vi "MC_8_28_12a_JW - Copy.vi"() -> ()   [LabVIEW 2011]
uses:
  <vilib>/Utility/file.llb/Read From Spreadsheet File (string).vi
  <vilib>/regexp/Match Regular Expression.xnode
  <vilib>/Utility/file.llb/Write To Spreadsheet File (string).vi
  <vilib>/Utility/file.llb/Write To Spreadsheet File (DBL).vi
  <vilib>/Utility/inputDevices.llb/keyboardAcquire.vi
panel:
  out "Vg Column":dbl[](array[numeric])
  out "Data Length":dbl
  out "X Axis Display Type":string
  out "Opj X Axis":string
  in  "Room Temp":dbl=294.0
  out "No Image 2":path=path "\\\\acad1\\physics/Jurchescu-group/JW-PD/Image Not Found.png"
  out "Save1 Array":string[][](array[string])
  out "Lin Vd":dbl
  out "Lin-Vg Array-Used":dbl[](array[numeric])
  out "Lin Id-Used":dbl[](array[numeric])
  out "Rec: Comments":string
  out "Folder Index":dbl caption="Length"
  out "Current \nRecord":string[](array[string])
  out "Transformer \nHeaders":string[](array[string])
  out "Current Device ID":string
  out "Column":string
  out "Row":string
  out "Rec: Concentration":dbl
  out "Rec: Solvent":string
  out "Rec: Method":string
  in  "?":T1(tab)
  in  "Transport File":path
  out "Transport Folder":path
  out "Rec: Material":string
  out "Accel (RPM/s):":dbl
  in  "Transfer File":path
  out "Transfer Folder":path
  in  "Image Folder":path
  out "Image File":path=path "D:/UserData/Desktop/Jeremy/WFU/Research/Programs/VI mods/Image Not Found.png"
  in  "Manual Comments":bool
  in  "Comments:":string
  out "Calc: On/Off":dbl caption="On/Off-Sat" format="%#.2e"
  out "Calc: Off I-Sat":dbl caption="Off I-Sat" format="%#.2e"
  in  "Manuel-Dielectric":bool
  in  "Manuel-Length":bool
  out "Calc: VT-Lin":dbl
  out "New: VT-Lin":dbl
  out "Rec: VT-Lin":dbl caption="VT-Lin" format="%#_3g"
  out "Calc: Trap Density-STS":dbl format="%#.2e"
  out "New: Trap Density-STS":dbl format="%#.2e"
  out "Rec: Trap Density-STS":dbl caption="N-Sat (STS)" format="%#.2e"
  out "Calc: Trap Density-VT":dbl format="%#.2e"
  out "New: Trap Density-VT":dbl format="%#.2e"
  out "Rec: Trap Density-VT":dbl caption="N-Sat (VT)" format="%#.2e"
  out "Calc: Mobility-Lin":dbl format="%#.2e"
  out "New: Mobility-Lin":dbl format="%#_4e"
  out "Rec: Mobility-Lin":dbl caption="Mobility-Lin" format="%#_3e"
  out "Calc: Mobility-Sat":dbl format="%#.2e"
  out "Rec: Length":dbl caption="Length" format="%#_3g"
  out "Rec: Width":dbl caption="Width" format="%#_4g"
  out "Rec: Dielectric (d)":dbl caption="Dielectric (d)" format="%#_3g"
  in  "Cancel Button":bool
  in  "Up Button":bool
  in  "Down Button":bool
  out "Data Name:":string
  in  "Save Changes?":bool
  in  "New: Dielectric":dbl
  in  "New: Length":dbl
  in  "New: Width":dbl
  out "New: Mobility-Sat":dbl format="%#.2e"
  in  "Blank Button":bool
  in  "Zoom":i16(slide)=-3 scale=-5.0..5.0
  out "Image Out 2":T2(plugin-control)
  out "Image Out":T2(plugin-control)
  in  "Magnification":u16(ring) items=["5x", "10x", "20x", "50x", "80x"]
  out "Total Width":dbl
  out "Distances":dbl[](array[numeric])
  in  "Undo Button":bool
  in  "Remove Button":bool
  out "Rec: Mobility-Sat":dbl caption="Mobility-Sat" format="%#.2e"
  in  "Export":bool
  out "Calc: VT-Sat":dbl format="%#.2g"
  out "New: VT-Sat":dbl format="%#.2g"
  in  "Manual-Width":bool caption="Manual"
  out "Calc: STS":dbl format="%#.2g"
  out "New: STS":dbl format="%#.2g"
  out "Rec: VT-Sat":dbl caption="VT-Sat" format="%#.2g"
  out "Rec: STS":dbl caption="STS-Sat" format="%#.2g"
  out "Rec: On/Off":dbl caption="On/Off-Sat" format="%#.2e"
  in  "Save Changes? 2":bool
  in  "Save Changes? 3":bool
  out "Rec: Temp":dbl caption="Sample Temp" format="%.1f"
  in  "New: Temp":dbl format="%.1f"
  out "Rec: Off I-Sat":dbl caption="Off I-Sat" format="%#.2e"
  in  "Independant Variable":string(combo)="Length (um):"
  in  "Transfer Plots":T3(tab)=enum."Saturation"
  in  "Lin-Trans Slider":dbl(slide) step=1.0 scale=-22.0..89.0 scale format="%#_1p"
  out "Sqrt-Lin":cluster{dbl[], dbl[]}[](graph)
  in  "Next Sqrt Lin":bool
  in  "Previous Sqrt Lin":bool
  in  "Sat-Trans Slider":dbl(slide) step=1.0 scale=-40.0..40.0 scale format="%#_1p"
  out "Sqrt-Sat":cluster{dbl[], dbl[]}[](graph)
  in  "Previous Sqrt Sat":bool
  in  "Next Sqrt Sat":bool
  out "Raw- Lin":cluster{dbl[], dbl[]}[](graph)
  out "Raw- Sat":cluster{dbl[], dbl[]}[](graph)
  in  "Log Plots":enum32{"Linear", "Saturation", "Transport"}(tab)=enum."Saturation"
  in  "Lin-Log Slider":dbl(slide) step=1.0 scale=-1.0..82.0 scale format="%#_1p"
  in  "Previous Log Lin":bool
  in  "Next Log Lin":bool
  out "Log-Lin":cluster{dbl[], dbl[]}[](graph)
  in  "Sat-Log Slider":dbl(slide) step=1.0 scale=-1.0..82.0 scale format="%#_1p"
  in  "Previous Log Sat":bool
  in  "Next Log Sat":bool
  out "Sat-Log":cluster{dbl[], dbl[]}[](graph)
  out "Transport":cluster{dbl[], dbl[]}[](graph)
  in  "Manual-Temp":bool caption="Manual"
  out "Date Created":string caption="Fabricated"
  out "Date Recorded":string="Date Recorded" caption="Measured"
  out "Image Name":string
  out "Index":string
  in  "Num Pts":dbl=5.0
  in  "NumPoints Log":dbl=5.0 caption="Num Pts"
  in  "Transport Style Controls":T4 {"Transport Line Size" items=["Extra Small", "Small", "Medium", "Large", "Extra Large"]}
  in  "Origin Project File":path=path "\\\\acad1\\physics/Jurchescu-group/JW-PD/Group Library/Origin Project Files/DeviceData_8_10_12a_JW.opj"
  in  "No Image File":path=path "\\\\acad1\\physics/Jurchescu-group/JW-PD/Mega Awesome/Image Not Found.png"
  in  "Ramp (s):":dbl=3.0
  in  "Fabricator:":string="NaN"
  in  "Sample #:":dbl=1.0
  in  "Wait Time (s):":dbl=nan
  in  "RPM:":dbl=nan
  in  "Time (s):":dbl=nan
  in  "Room Temp (F):":dbl=nan
  in  "Relative Humidity (%):":dbl=nan
  in  "Solution Temp (C):":dbl=nan
  in  "# Drops*:":dbl=inf
  in  "Surface Treatment:":string="NaN"
  in  "Treatment Concentration (mM):":dbl=nan
  out "String":string
  out "Index 2":dbl
  out "Sat Id-Log-Used":dbl[](array[numeric])
  out "Vg Array-Log-Used":dbl[](array[numeric])
  out "ROI Descriptor out":T5 {"Contours"."Type" items=["No Selection", "Point", "Line", "Rectangle", "Oval", "Polygon", "Freehand Region", "Annulus", "Unused2", "Unused3", "Broken Line", "Freehand Line", "Rotated Rectangle"]}
  out "ROI Descriptor":T5 {"Contours"."Type" items=["No Selection", "Point", "Line", "Rectangle", "Oval", "Polygon", "Freehand Region", "Annulus", "Unused2", "Unused3", "Broken Line", "Freehand Line", "Rotated Rectangle"]}
  out "Numeric 3":dbl
  out "Array 6":dbl[][](array[numeric])
  out "Cluster":T6
  out "Array 5":dbl[](array[numeric])
  out "Array 4":dbl[](array[numeric])
  out "Array 3":dbl[](array[numeric])
  out "Numeric 2":dbl
  out "Numeric":dbl
  out "Sat Id-Used":dbl[](array[numeric])
  out "Sat Vg Array-Used":dbl[](array[numeric])
  out "MobVi Index":dbl
  in  "Row Start":dbl=20.0
  # "Data Locations"
  # "Transfer Location"
  # "Image Location"
  # "Recorded"
  # "Calculated"
  # "Re-Calculated"
  # "Manual"
  # "Used points display at y=0"
  # "Slider\nDoesn't\nWork"
  # "Slider\nDoesn't\nWork"
  # "No new points displayed"
  # "Sample Properties"
  # "*     Inf = Full coverage\n   NaN = Unknown or Not Applicable"
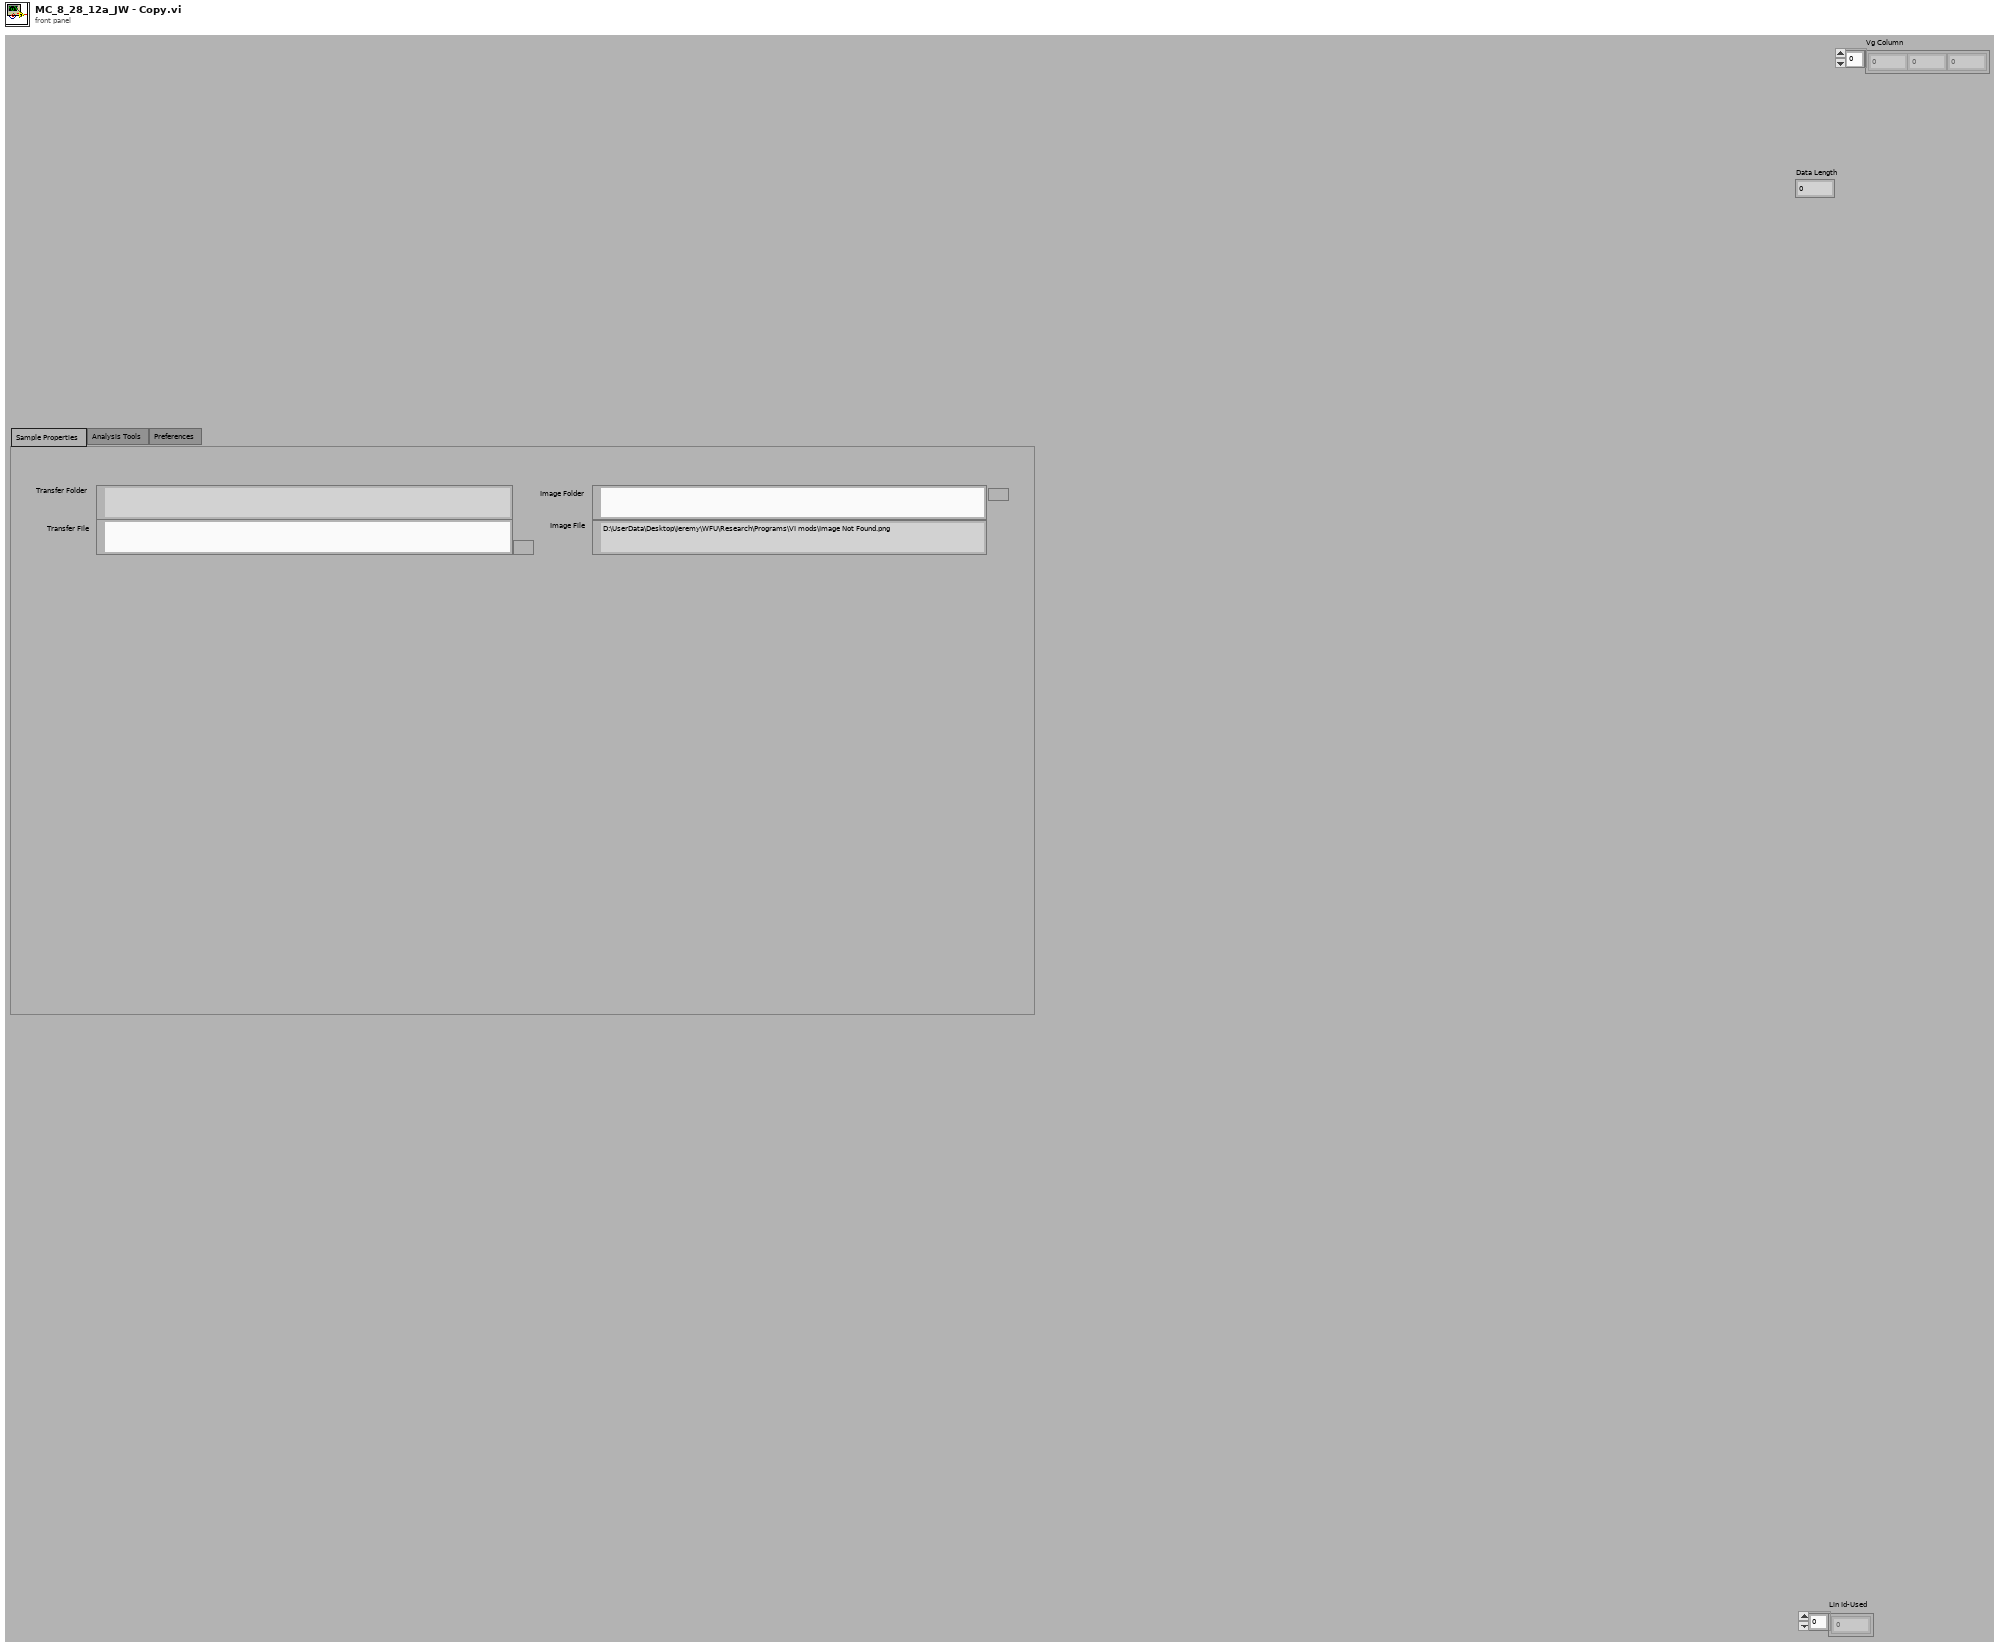
[diagram p1: front panel]
types:
  T1 = enum32{"Sample Properties", "Analysis Tools", "Preferences", "Current Database"}
  T2 = typedef "IMAQ Image.ctl" = refnum<image>
  T3 = enum32{"Linear", "Saturation", "Raw-Linear", "Raw-Saturation"}
  T4 = cluster{"Transport Line Size":u16, "Transport Line Color":u32}
  T5 = typedef "ROI Descriptor" = cluster{"Global Rectangle":i32[], "Contours":cluster{"ID":enum32{"External", "Internal"}, "Type":u32, "Coordinates":i32[]}[]}
  T6 = cluster{"Numeric":dbl, "Numeric 2":dbl, "Numeric 3":dbl, "Numeric 4":dbl}
  T7 = cluster{"Mobility-Sat":dbl, "Moblitity-Lin":dbl, "On/Off":dbl, "Off Current":dbl, "Vt-Sat":dbl, "STS":dbl, "Trap Density-VT":dbl, "Trap Density-STS":dbl}
  T8 = cluster{"Date Recorded":string, "Index":string, "Length":dbl, "Width":dbl, "Sample Temp":dbl}
  T9 = cluster{"Date Created":string, "Material":string, "Solvent":string, "Concentration":dbl, "Method":string, "Dielectric (nm)":dbl, "Treatment":string, "Comments":string}
  T10 = cluster{"Sat Vg Used":dbl[], "Sat Log(Id) Used":dbl[], "Lin Vg Used":dbl[], "Lin Log(Id) Used":dbl[], "STS Index-Sat":dbl, "STS Index-Lin":dbl}
  T11 = cluster{"Raw Sat":cluster{dbl[], dbl[]}[], "Sqrt Sat":cluster{dbl[], dbl[]}[], "Log Sat":cluster{dbl[], dbl[]}[], "Raw Lin":cluster{dbl[], dbl[]}[], "Sqrt Lin":cluster{dbl[], dbl[]}[], "Log Lin":cluster{dbl[], dbl[]}[]}
  T12 = cluster{"Mobility-Sat":dbl, "Vt-Sat":dbl, "Mobility-Lin":dbl, "Vt-Lin":dbl, "Off I-Sat":dbl, "On/Off I-Sat":dbl}
  T13 = cluster{"[0]":cluster{dbl[], dbl[]}, "[1]":cluster{dbl[], dbl[]}, "[2]":cluster{dbl[], dbl[]}, "[3]":cluster{dbl[], dbl[]}, "[4]":cluster{dbl[], dbl[]}, "[5]":cluster{dbl[], dbl[]}, "[6]":cluster{dbl[], dbl[]}, "[7]":cluster{dbl[], dbl[]}, "[8]":cluster{dbl[], dbl[]}}
  T14 = typedef "LVBoundsTypeDef.ctl" = cluster{"Width":u32, "Height":u32}
  T15 = cluster{"Global Rectangle":i32[], "Contours":cluster{"Contour Type":u32, "ROI Type":u32, "Points":i32[]}[]}
  T16 = cluster{"Contour Type":u32, "ROI Type":u32, "Points":i32[]}[]
  T17 = cluster{i32[], cluster{"Contour Type":u32, "ROI Type":u32, "Points":i32[]}[]}
  T18 = enum16{"0", "1", "2", "3", "4", "5", "6", "7", "8", "9", "A", "B", "C", "D", "E", "F", "G", "H", "I", "J", "K", "L", "M", "N", "O", "P", "Q", "R", "S", "T", "U", "V", "W", "X", "Y", "Z", "F1", "F2", "F3", "F4", "F5", "F6", "F7", "F8", "F9", "F10", "F11", "F12", "F13", "F14", "F15", "ADD", "BACK", "BACKSLASH", "CAPITAL", "COMMA", "DECIMAL", "DELETE", "DIVIDE", "DOWN", "END", "EQUALS", "ESCAPE", "GRAVE (`)", "HOME", "INSERT", "LBRACKET", "LCONTROL", "LEFT", "L ALT", "LSHIFT", "LWIN", "MINUS", "MULTIPLY", "NEXT", "NUMLOCK", "NUMPAD_0", "NUMPAD_1", "NUMPAD_2", "NUMPAD_3", "NUMPAD_4", "NUMPAD_5", "NUMPAD_6", "NUMPAD_7", "NUMPAD_8", "NUMPAD_9", "PAUSE", "PERIOD", "PRIOR (PG UP)", "RBRACKET", "RCONTROL", "RETURN", "RIGHT", "R ALT", "RSHIFT", "RWIN", "SCROLL", "SEMICOLON", "SLASH", "SPACE", "SUBTRACT", "TAB", "UP", "ENTER (num pad)", "' (quote)"}[]
  T19 = enum16{"0", "1", "2", "3", "4", "5", "6", "7", "8", "9", "A", "B", "C", "D", "E", "F", "G", "H", "I", "J", "K", "L", "M", "N", "O", "P", "Q", "R", "S", "T", "U", "V", "W", "X", "Y", "Z", "F1", "F2", "F3", "F4", "F5", "F6", "F7", "F8", "F9", "F10", "F11", "F12", "F13", "F14", "F15", "ADD", "BACK", "BACKSLASH", "CAPITAL", "COMMA", "DECIMAL", "DELETE", "DIVIDE", "DOWN", "END", "EQUALS", "ESCAPE", "GRAVE (`)", "HOME", "INSERT", "LBRACKET", "LCONTROL", "LEFT", "L ALT", "LSHIFT", "LWIN", "MINUS", "MULTIPLY", "NEXT", "NUMLOCK", "NUMPAD_0", "NUMPAD_1", "NUMPAD_2", "NUMPAD_3", "NUMPAD_4", "NUMPAD_5", "NUMPAD_6", "NUMPAD_7", "NUMPAD_8", "NUMPAD_9", "PAUSE", "PERIOD", "PRIOR (PG UP)", "RBRACKET", "RCONTROL", "RETURN", "RIGHT", "R ALT", "RSHIFT", "RWIN", "SCROLL", "SEMICOLON", "SLASH", "SPACE", "SUBTRACT", "TAB", "UP", "ENTER (num pad)", "' (quote)"}
  T20 = cluster{"Independant  Variable Indicator":string, "Parameter String Indicator":string}
  T21 = cluster{string, sgl, bool, bool, bool, bool, bool, bool, i32}
  T22 = cluster{i32, cluster{string, sgl, bool, bool, bool, bool, bool, bool, i32}, i32, i32}
  T23 = cluster{"Contour Type":u32, "ROI Type":u32, "Points":i32[]}
  T24 = cluster{"Points[0]":i32, "Points[1]":i32, "Points[2]":i32, "Points[3]":i32, "Points[4]":i32, "Points[5]":i32, "Points[6]":i32, "Points[7]":i32, "Points[8]":i32}
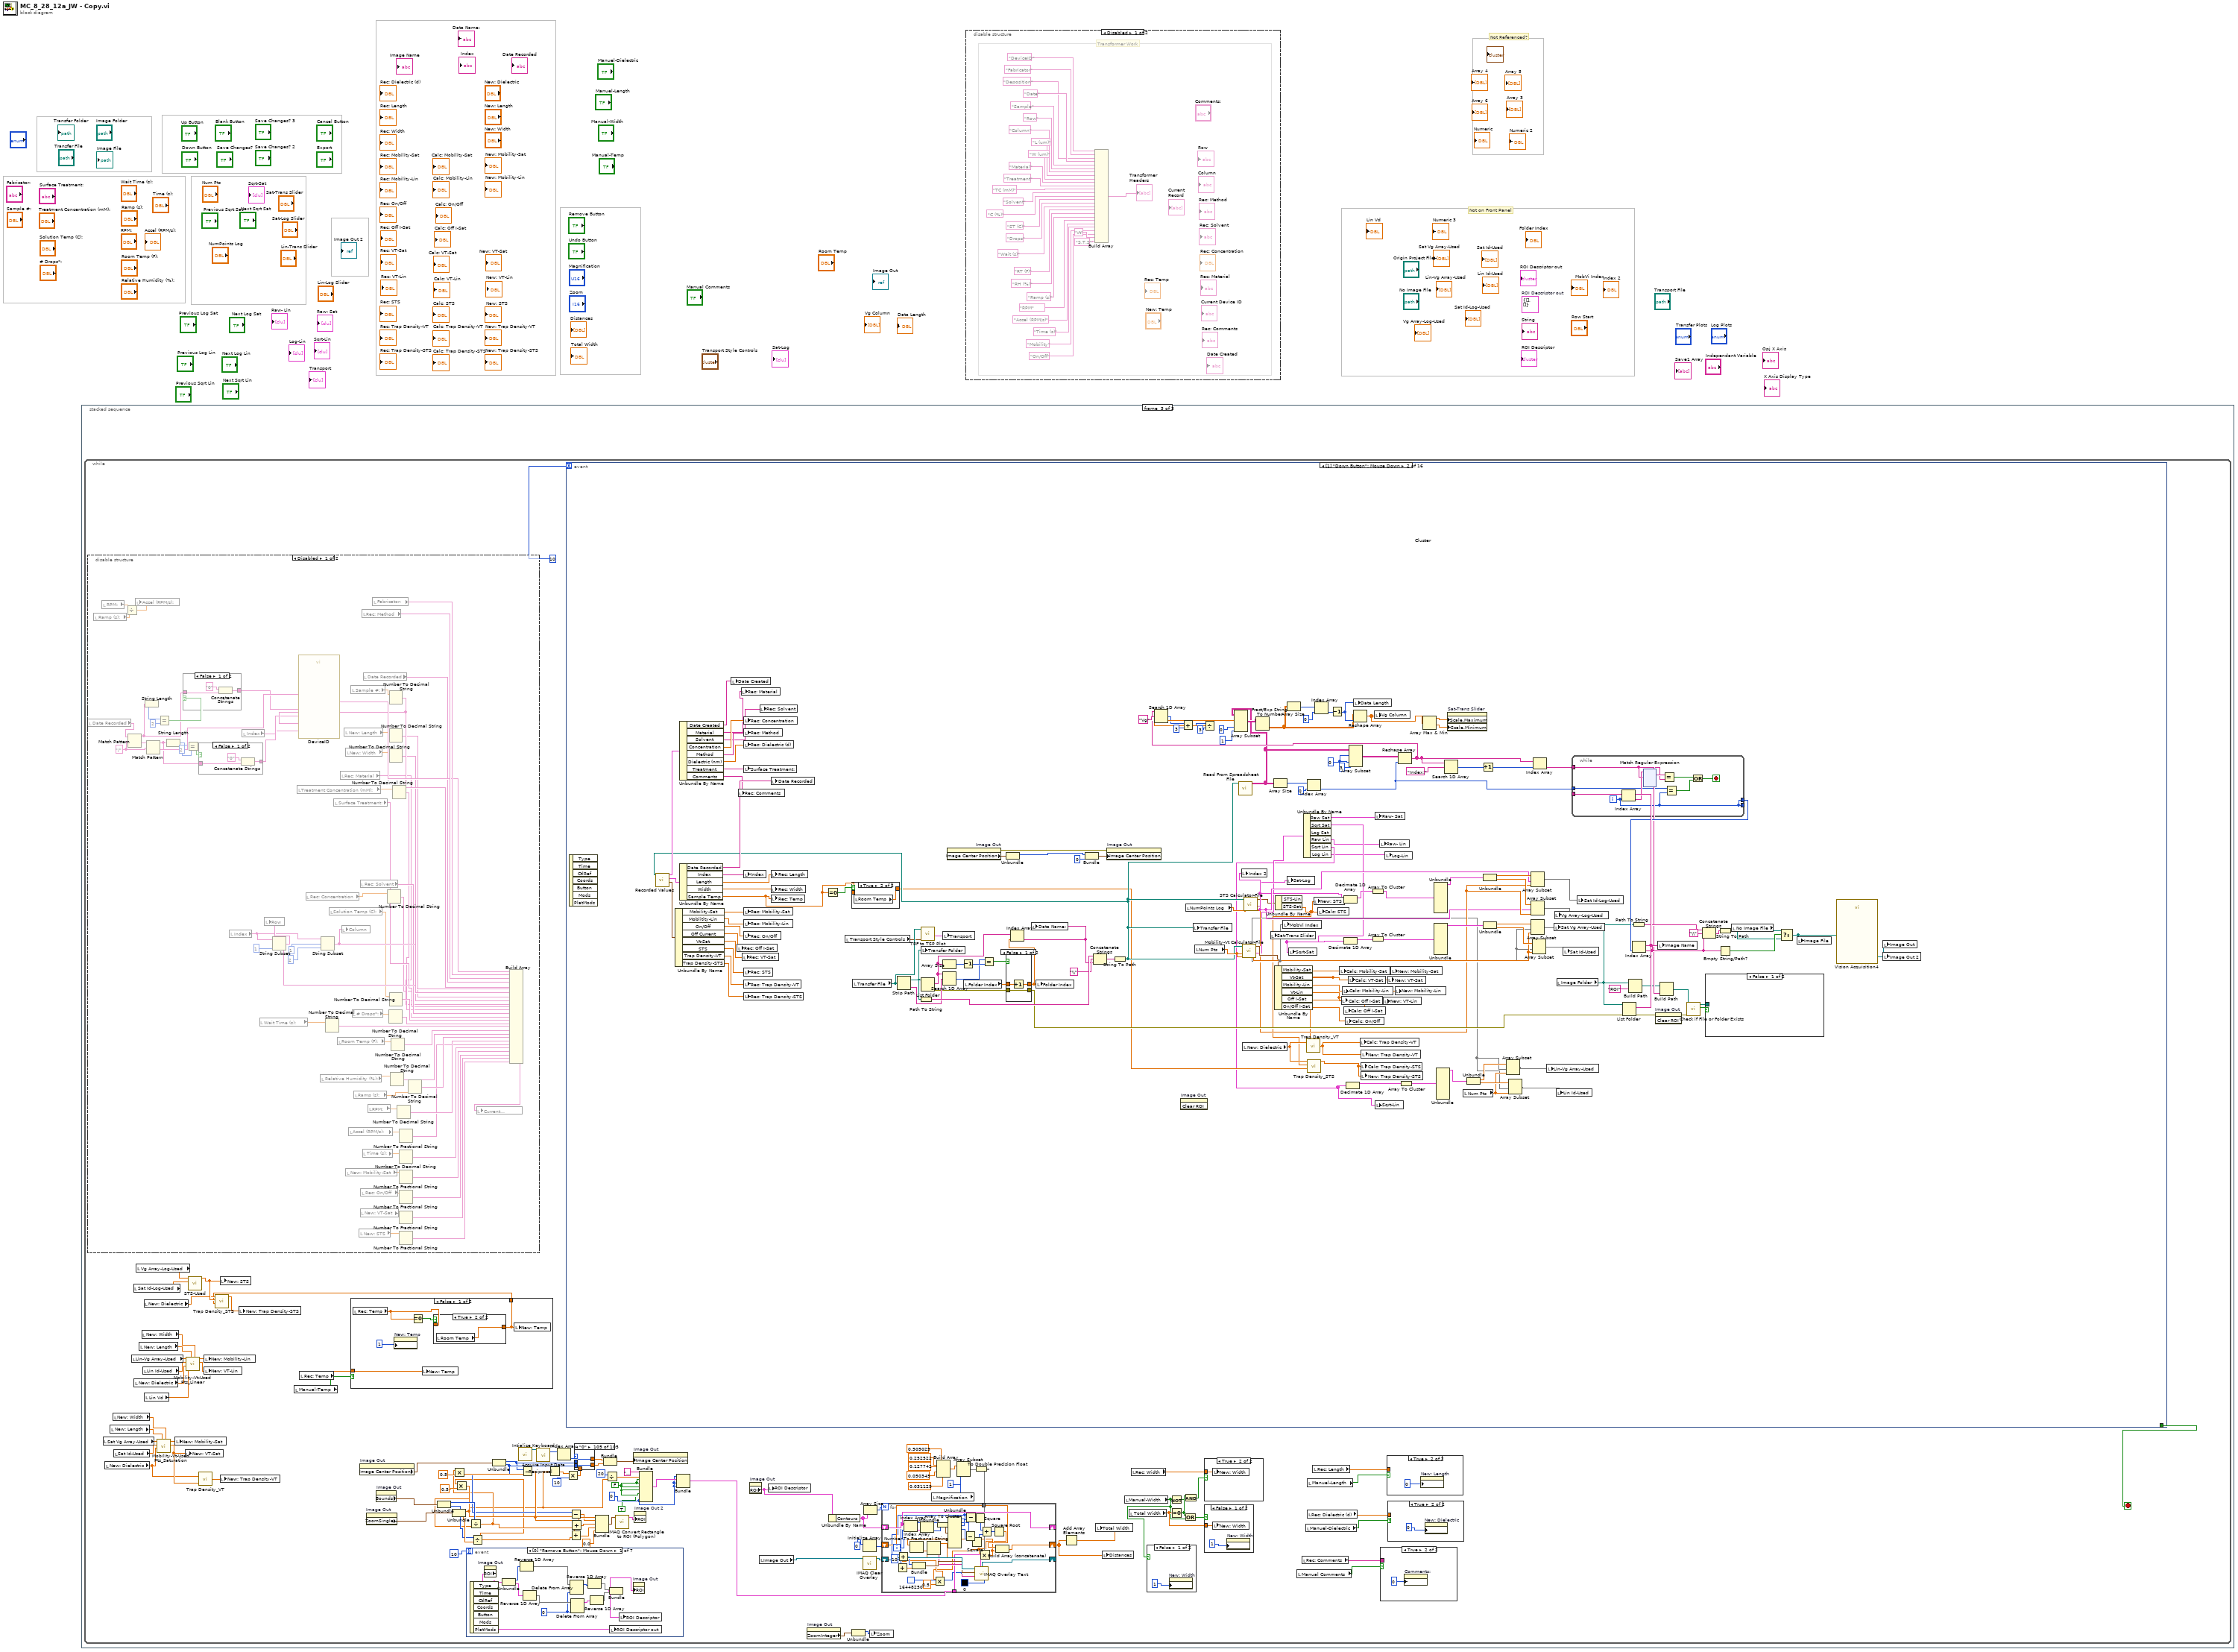
[diagram p0: block diagram]
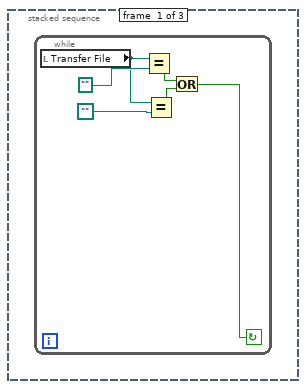
[diagram p3: hidden frame]
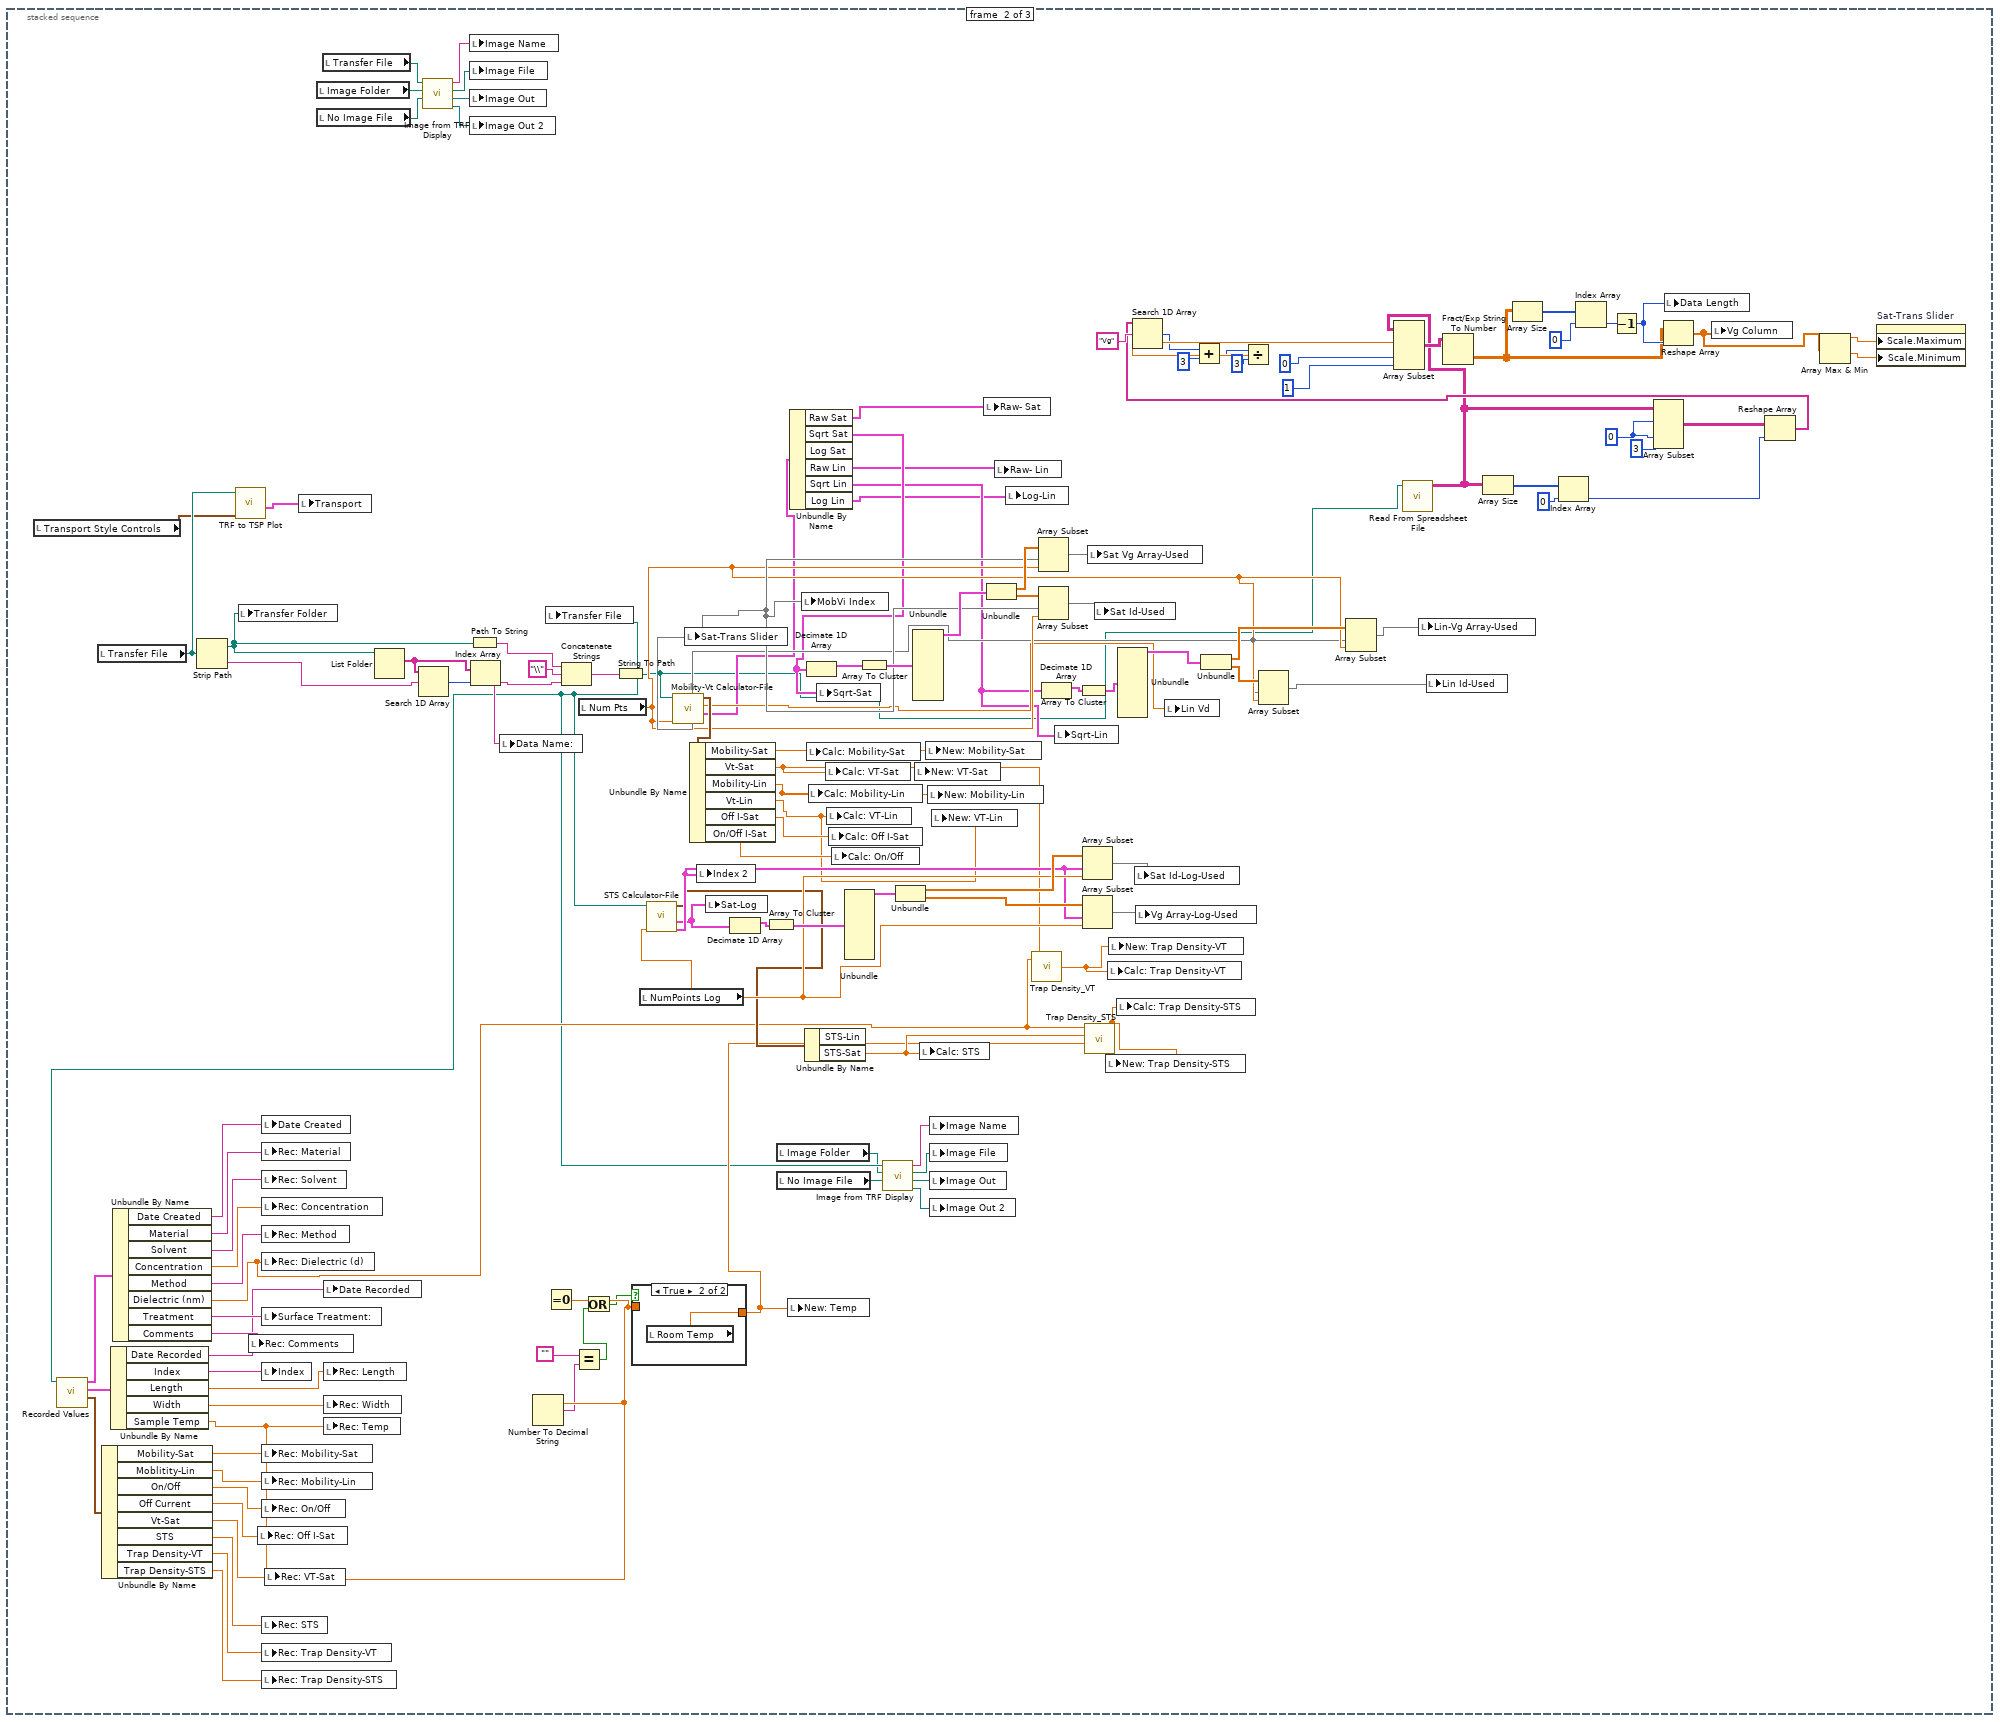
[diagram p4: hidden frame]
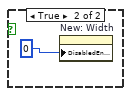
[diagram p9: hidden frame]
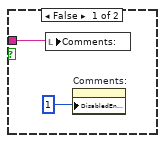
[diagram p10: hidden frame]
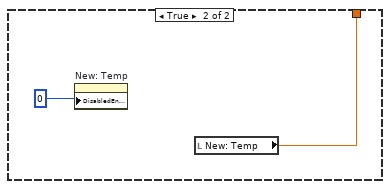
[diagram p12: hidden frame]
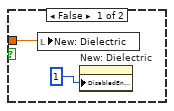
[diagram p13: hidden frame]
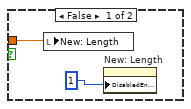
[diagram p14: hidden frame]
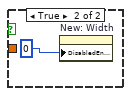
[diagram p16: hidden frame]
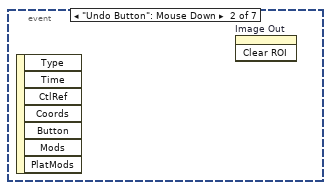
[diagram p17: hidden frame]
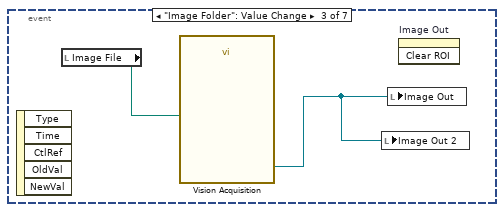
[diagram p18: hidden frame]
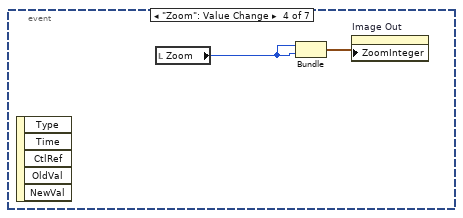
[diagram p19: hidden frame]
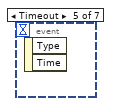
[diagram p20: hidden frame]
diagram:
  (unwired) T5 {"Global Rectangle"=[], "Contours"=[]}  # ROI Descriptor out
  # "Not Referenced?"
  # "Not on Front Panel"
  n1 = stacked-sequence {
    frame #0 {
      n2 = while {
        stop <- w1 continue-if-true
        n3 = local read "Transfer File"() -> (w3:path)
        n4 = Equal?(x=w3, y=path "") -> (x = y?=w5:bool)
        n5 = Equal?(x=w3, y=path "") -> (x = y?=w4:bool)
        n6 = Or(x=w5, y=w4) -> (x .or. y?=w1:bool)
      }
    }
    frame #1 {
      w45 = 0
      n7 = local read "Transport Style Controls"() -> (w7:T4)
      n8 = local read "Transfer File"() -> (w9:path)
      n9 = Strip Path(path=w9) -> (stripped path=w51:path, name=w124:string)
      n10 = call "TRF to TSP Plot.vi"("Transport Graph Properties"=w7, "Transfer File"=w9) -> ("Transport"=w8:cluster{ext[], ext[]}[])  [unwired: 7 in, 2 out]
      n11 = local write "Transfer Folder"(w51) -> ()
      n12 = local write "Transport"(w8) -> ()
      n13 = local read "Image Folder"() -> (w18:path)
      n14 = local read "No Image File"() -> (w17:path)
      n15 = local read "Transfer File"() -> (w23:path)
      n16 = List Folder(path=w51) -> (filenames=w128:string[])  [unwired: 3 in, 3 out]
      n17 = Search 1D Array(1D array=w128, element=w124) -> (index of element=w127:i32)  [unwired: 1 in]
      n18 = call "Image from TRF Display.vi"("No Image File"=w17, "Image Folder"=w18, "Transfer File"=w23) -> ("Image Out 2"=w19:T2, "Image Out"=w20:T2, "Image File"=w21:path, "Image Name"=w22:string)  [unwired: 5 in]
      n19 = local write "Image Name"(w22) -> ()
      n20 = local write "Image File"(w21) -> ()
      n21 = local write "Image Out"(w20) -> ()
      n22 = local write "Image Out 2"(w19) -> ()
      n23 = Path To String(path=w51) -> (string=w123:string)
      n24 = Index Array(array=w128, index=w127) -> (element=w50:string)
      n25 = local write "Data Name:"(w50) -> ()
      n26 = Concatenate Strings(w123, "\\", w50) -> (w125:string)
      n27 = local read "Num Pts"() -> (w80:dbl)
      n28 = String To Path(string=w125) -> (path=w16:path)
      n29 = call "Recorded Values.vi"("Path"=w16) -> ("Recorded Char"=w110:T7, "Recorded Prop"=w109:T8, "Fabrication Prop"=w111:T9)  [unwired: 8 in]
      n30 = Unbundle By Name(w110) -> ("Mobility-Sat"=w98:dbl, "Moblitity-Lin"=w97:dbl, "On/Off"=w96:dbl, "Off Current"=w95:dbl, "Vt-Sat"=w61:dbl, "STS"=w94:dbl, "Trap Density-VT"=w93:dbl, "Trap Density-STS"=w92:dbl)
      n31 = Unbundle By Name(w109) -> ("Date Recorded"=w102:string, "Index"=w101:string, "Length"=w100:dbl, "Width"=w99:dbl, "Sample Temp"=w67:dbl)
      n32 = Unbundle By Name(w111) -> ("Date Created"=w91:string, "Material"=w108:string, "Solvent"=w107:string, "Concentration"=w106:dbl, "Method"=w105:string, "Dielectric (nm)"=w71:dbl, "Treatment"=w104:string, "Comments"=w103:string)
      n33 = local write "Rec: Comments"(w103) -> ()
      n34 = local write "Rec: Off I-Sat"(w95) -> ()
      n35 = local write "Date Created"(w91) -> ()
      n36 = local write "Rec: Material"(w108) -> ()
      n37 = local write "Rec: Solvent"(w107) -> ()
      n38 = local write "Rec: Concentration"(w106) -> ()
      n39 = local write "Rec: Method"(w105) -> ()
      n40 = local write "Rec: Dielectric (d)"(w71) -> ()
      n41 = local write "Surface Treatment:"(w104) -> ()
      n42 = local write "Index"(w101) -> ()
      n43 = local write "Rec: Mobility-Sat"(w98) -> ()
      n44 = local write "Rec: Mobility-Lin"(w97) -> ()
      n45 = local write "Rec: On/Off"(w96) -> ()
      n46 = local write "Rec: STS"(w94) -> ()
      n47 = local write "Rec: Trap Density-VT"(w93) -> ()
      n48 = local write "Rec: Trap Density-STS"(w92) -> ()
      n49 = local write "Rec: VT-Sat"(w61) -> ()
      n50 = local write "Date Recorded"(w102) -> ()
      n51 = local write "Rec: Length"(w100) -> ()
      n52 = local write "Rec: Width"(w99) -> ()
      n53 = local write "Rec: Temp"(w67) -> ()
      n54 = Number To Decimal String(number=w67) -> (decimal integer string=w65:string)  [unwired: 1 in]
      n55 = local write "Transfer File"(w16) -> ()
      n56 = Equal To 0?(x=w67) -> (x = 0?=w66:bool)
      n57 = Equal?(x="", y=w65) -> (x = y?=w63:bool)
      n58 = Or(x=w66, y=w63) -> (x .or. y?=w62:bool)
      n59 = case shown="True" w62 {
        tunnel: [w132 w133] -> w73
        tunnel: w67 -> [w132 _]
        frame False {
        }
        frame True {
          n60 = local read "Room Temp"() -> (w133:dbl)
        }
      }
      n61 = local read "NumPoints Log"() -> (w88:dbl)
      n62 = call "STS Calculator-File.vi"("NumPts"=w88, "Path"=w16) -> ("Used Points"=w87:T10, "XY Graph-Sat"=w49:cluster{dbl[], dbl[]}[], "Ouput"=w86:cluster{"STS-Sat":dbl, "STS-Lin":dbl})  [unwired: 6 in, 1 out]
      n63 = call "Mobility-Vt Calculator-File.vi"("NumPts"=w80, "Path"=w16) -> ("Graph Cluster"=w52:T11, "Lin Vd"=w76:dbl, "Output"=w90:T12, 4:w89, 5:w79)  [unwired: 4 in, 1 out]
      n64 = local write "Sat-Trans Slider"(w89) -> ()
      n65 = Unbundle By Name(w90) -> ("Mobility-Sat"=w70:dbl, "Vt-Sat"=w69:dbl, "Mobility-Lin"=w60:dbl, "Vt-Lin"=w58:dbl, "Off I-Sat"=w75:dbl, "On/Off I-Sat"=w59:dbl)
      n66 = local write "Index 2"(w87) -> ()
      n67 = local write "Sat-Log"(w49) -> ()
      n68 = Decimate 1D Array(w49) -> (w115:cluster{dbl[], dbl[]}[])  [unwired: 1 out]
      n69 = Array To Cluster(array=w115) -> (cluster=w117:T13)
      n70 = local read "Image Folder"() -> (w15:path)
      n71 = local read "No Image File"() -> (w14:path)
      n72 = local write "New: Temp"(w73) -> ()
      n73 = Unbundle By Name(w52) -> ("Raw Sat"=w55:cluster{dbl[], dbl[]}[], "Sqrt Sat"=w57:cluster{dbl[], dbl[]}[], "Raw Lin"=w54:cluster{dbl[], dbl[]}[], "Sqrt Lin"=w56:cluster{dbl[], dbl[]}[], "Log Lin"=w53:cluster{dbl[], dbl[]}[])  [unwired: 1 out]
      n74 = local write "MobVi Index"(w89) -> ()
      n75 = Unbundle By Name(w86) -> ("STS-Sat"=w74:dbl)  [unwired: 1 out]
      n76 = Decimate 1D Array(w57) -> (w131:cluster{dbl[], dbl[]}[])  [unwired: 1 out]
      n77 = local write "Calc: Mobility-Sat"(w70) -> ()
      n78 = local write "Calc: Mobility-Lin"(w60) -> ()
      n79 = local write "Sqrt-Sat"(w57) -> ()
      n80 = local write "Calc: VT-Sat"(w69) -> ()
      n81 = local write "Calc: VT-Lin"(w58) -> ()
      n82 = local write "Calc: Off I-Sat"(w75) -> ()
      n83 = local write "Calc: On/Off"(w59) -> ()
      n84 = Unbundle(w117) -> ("[0]"=w116:cluster{dbl[], dbl[]})  [unwired: 8 out]
      n85 = Array To Cluster(array=w131) -> (cluster=w129:T13)
      n86 = call "Image from TRF Display.vi"("No Image File"=w14, "Image Folder"=w15, "Transfer File"=w16) -> ("Image Out 2"=w10:T2, "Image Out"=w11:T2, "Image File"=w13:path, "Image Name"=w12:string)  [unwired: 5 in]
      n87 = Unbundle(w116) -> (w113:dbl[], w112:dbl[])
      n88 = Unbundle(w129) -> ("[0]"=w130:cluster{dbl[], dbl[]})  [unwired: 8 out]
      n89 = local write "New: VT-Sat"(w69) -> ()
      n90 = local write "Calc: STS"(w74) -> ()
      n91 = local write "New: Mobility-Sat"(w70) -> ()
      n92 = local write "New: Mobility-Lin"(w60) -> ()
      n93 = local write "Image Name"(w12) -> ()
      n94 = local write "Image File"(w13) -> ()
      n95 = local write "Image Out"(w11) -> ()
      n96 = local write "Image Out 2"(w10) -> ()
      n97 = local write "New: VT-Lin"(w58) -> ()
      n98 = local write "Raw- Sat"(w55) -> ()
      n99 = Unbundle(w130) -> (w114:dbl[], w118:dbl[])
      n100 = local write "Raw- Lin"(w54) -> ()
      n101 = local write "Log-Lin"(w53) -> ()
      n102 = call "Trap Density_VT.vi"("VT"=w69, "Dielectric"=w71) -> ("Trap Density-VT"=w68:dbl)
      n103 = Array Subset(array=w114, index=w89, length=w80) -> (w121:dbl[])
      n104 = Array Subset(array=w118, index=w89, length=w80) -> (w122:dbl[])
      n105 = Decimate 1D Array(w56) -> (w85:cluster{dbl[], dbl[]}[])  [unwired: 1 out]
      n106 = local write "Sqrt-Lin"(w56) -> ()
      n107 = Array To Cluster(array=w85) -> (cluster=w84:T13)
      n108 = Array Subset(array=w113, index=w87, length=w88) -> (w120:dbl[])
      n109 = Array Subset(array=w112, index=w87, length=w88) -> (w119:dbl[])
      n110 = call "Trap Density_STS.vi"("Temp (T) [K]"=w73, "S.T.S. (S)"=w74, "Dielectric"=w71) -> ("Trap Density (N)"=w72:dbl)  [unwired: 8 in]
      n111 = local write "Sat Vg Array-Used"(w121) -> ()
      n112 = local write "Sat Id-Used"(w122) -> ()
      n113 = local write "New: Trap Density-STS"(w72) -> ()
      n114 = local write "Calc: Trap Density-VT"(w68) -> ()
      n115 = local write "New: Trap Density-VT"(w68) -> ()
      n116 = local write "Calc: Trap Density-STS"(w72) -> ()
      n117 = Unbundle(w84) -> ("[0]"=w83:cluster{dbl[], dbl[]})  [unwired: 8 out]
      n118 = local write "Sat Id-Log-Used"(w120) -> ()
      n119 = local write "Vg Array-Log-Used"(w119) -> ()
      n120 = local write "Lin Vd"(w76) -> ()
      n121 = Unbundle(w83) -> (w82:dbl[], w81:dbl[])
      n122 = Array Subset(array=w81, index=w79, length=w80) -> (w77:dbl[])
      n123 = Array Subset(array=w82, index=w79, length=w80) -> (w78:dbl[])
      n124 = call-poly <vilib>:"Read From Spreadsheet File.vi"("file path (dialog if empty)"=w16) -> ("all rows"=w27:string[][])  [unwired: 6 in, 4 out]
      n125 = local write "Lin-Vg Array-Used"(w78) -> ()
      n126 = local write "Lin Id-Used"(w77) -> ()
      n127 = Array Size(array=w27) -> (size(s)=w46:i32[])
      n128 = Index Array(array=w46, index=0) -> (element=w44:i32)
      n129 = Array Subset(array=w27, index (row)=w45, index (col)=w45, length (col)=3) -> (w47:string[][])  [unwired: 1 in]
      n130 = Reshape Array(w47, w44) -> (w29:string[])
      n131 = Search 1D Array(1D array=w29, element="Vg") -> (index of element=w33:i32)  [unwired: 1 in]
      n132 = Add(x=w33, y=3) -> (x+y=w31:i32)
      n133 = Divide(x=w31, y=3) -> (x/y=w38:dbl)
      n134 = Array Subset(array=w27, index (row)=w38, index (col)=0, length (col)=1) -> (w37:string[][])  [unwired: 1 in]
      n135 = Fract/Exp String To Number(string=w37) -> (number=w41:dbl[][])  [unwired: 3 in, 1 out]
      n136 = Array Size(array=w41) -> (size(s)=w28:i32[])
      n137 = Index Array(array=w28, index=0) -> (element=w39:i32)
      n138 = Decrement(x=w39) -> (x-1=w42:i32)
      n139 = Reshape Array(w41, w42) -> (w26:dbl[])
      n140 = local write "Data Length"(w42) -> ()
      n141 = local write "Vg Column"(w26) -> ()
      n142 = Array Max & Min(array=w26) -> (max value=w25:dbl, min value=w24:dbl)  [unwired: 2 out]
      n143 = property on="Sat-Trans Slider" class="Slide (strict)"("Scale.Maximum"=w25, "Scale.Minimum"=w24) -> ()  [unwired: 2 in, 2 out]
    }
    frame #2 {
      n144 = while {
        stop <- w233 stop-if-true
        w183 = FALSE
        w181 = 0
        n145 = disable-structure shown="Disabled" {
          frame Disabled {
            w267 = "/"
            n146 = local read "Date Recorded"() -> (w270:string)
            n147 = local read "Ramp (s):"() -> (w237:dbl)
            n148 = local read "RPM:"() -> (w238:dbl)
            n149 = Divide(x=w238, y=w237) -> (x/y=w236:dbl)
            n150 = Match Pattern(string=w270, regular expression=w267) -> (before substring=w261:string, after substring=w268:string)  [unwired: 1 in, 2 out]
            n151 = local write "Accel (RPM/s):"(w236) -> ()
            n152 = String Length(string=w261) -> (length=w264:i32)
            n153 = Match Pattern(string=w268, regular expression=w267) -> (before substring=w255:string, after substring=w266:string)  [unwired: 1 in, 2 out]
            n154 = Equal?(x=w264, y=2) -> (x = y?=w262:bool)
            n155 = String Length(string=w255) -> (length=w257:i32)
            n156 = case shown="False" w262 {
              tunnel: w261 -> [w307 w309]
              tunnel: [w306 w309] -> w260
              frame False {
                n157 = Concatenate Strings("0", w307) -> (w306:string)
              }
              frame True {
              }
            }
            n158 = Equal?(x=w257, y=2) -> (x = y?=w259:bool)
            n159 = case shown="False" w259 {
              tunnel: w255 -> [w303 w305]
              tunnel: [w302 w305] -> w256
              frame False {
                n160 = Concatenate Strings("0", w303) -> (w302:string)
              }
              frame True {
              }
            }
            n161 = local read "Index"() -> (w240:string)
            n162 = local read "Index"() -> (w254:string)
            n163 = local read "Wait Time (s):"() -> (w300:dbl)
            n164 = String Subset(string=w240, length (rest)=1) -> (substring=w295:string)  [unwired: 1 in]
            n165 = local write "Row"(w295) -> ()
            n166 = local read "Treatment Concentration (mM):"() -> (w248:dbl)
            n167 = local read "Rec: Concentration"() -> (w235:dbl)
            n168 = local read "Relative Humidity (%):"() -> (w245:dbl)
            n169 = String Subset(string=w240, offset (0)=1, length (rest)=2) -> (substring=w296:string)
            n170 = Number To Decimal String(number=w300) -> (decimal integer string=w301:string)  [unwired: 1 in]
            n171 = local read "Solution Temp (C):"() -> (w289:dbl)
            n172 = local read "Surface Treatment:"() -> (w247:string)
            n173 = local read "Room Temp (F):"() -> (w293:dbl)
            n174 = local read "Rec: Material"() -> (w243:string)
            n175 = local write "Column"(w296) -> ()
            n176 = local read "New: Length"() -> (w253:dbl)
            n177 = local read "New: Width"() -> (w252:dbl)
            n178 = local read "New: Mobility-Sat"() -> (w282:dbl)
            n179 = local read "Accel (RPM/s):"() -> (w280:dbl)
            n180 = local read "Sample #:"() -> (w272:dbl)
            n181 = local read "# Drops*:"() -> (w290:dbl)
            n182 = local read "Ramp (s):"() -> (w298:dbl)
            n183 = local read "New: STS"() -> (w274:dbl)
            n184 = local read "Rec: Solvent"() -> (w249:string)
            n185 = local read "New: VT-Sat"() -> (w276:dbl)
            n186 = local read "Rec: On/Off"() -> (w278:dbl)
            n187 = local read "Rec: Method"() -> (w273:string)
            n188 = local read "Time (s):"() -> (w285:dbl)
            n189 = local read "Date Recorded"() -> (w269:string)
            n190 = local read "RPM:"() -> (w286:dbl)
            n191 = local read "Fabricator:"() -> (w294:string)
            n192 = Number To Decimal String(number=w235) -> (decimal integer string=w234:string)  [unwired: 1 in]
            n193 = Number To Decimal String(number=w290) -> (decimal integer string=w291:string)  [unwired: 1 in]
            n194 = Number To Decimal String(number=w272) -> (decimal integer string=w265:string)  [unwired: 1 in]
            n195 = call "DeviceID"("Sample"=w265, "Year"=w266, "Month"=w260, "Day"=w256, "Index"=w254) -> ("Result"=w271:string)  [unwired: 9 in, 1 out]
            n196 = Number To Decimal String(number=w253) -> (decimal integer string=w251:string)  [unwired: 1 in]
            n197 = Number To Decimal String(number=w252) -> (decimal integer string=w250:string)  [unwired: 1 in]
            n198 = Number To Decimal String(number=w289) -> (decimal integer string=w288:string)  [unwired: 1 in]
            n199 = Number To Decimal String(number=w245) -> (decimal integer string=w244:string)  [unwired: 1 in]
            n200 = Number To Decimal String(number=w293) -> (decimal integer string=w292:string)  [unwired: 1 in]
            n201 = Number To Decimal String(number=w248) -> (decimal integer string=w246:string)  [unwired: 1 in]
            n202 = Number To Decimal String(number=w286) -> (decimal integer string=w287:string)  [unwired: 1 in]
            n203 = Number To Fractional String(number=w280) -> (F-format string=w281:string)  [unwired: 3 in]
            n204 = Number To Decimal String(number=w285) -> (decimal integer string=w284:string)  [unwired: 1 in]
            n205 = Number To Fractional String(number=w282) -> (F-format string=w283:string)  [unwired: 3 in]
            n206 = Number To Fractional String(number=w278) -> (F-format string=w279:string)  [unwired: 3 in]
            n207 = Number To Fractional String(number=w276) -> (F-format string=w277:string)  [unwired: 3 in]
            n208 = Number To Fractional String(number=w274) -> (F-format string=w275:string)  [unwired: 3 in]
            n209 = Number To Decimal String(number=w298) -> (decimal integer string=w299:string)  [unwired: 1 in]
            n210 = Build Array(w271, w294, w273, w269, w265, w295, w296, w251, w250, w243, w247, w246, w249, w234, w288, w291, w301, w292, w244, w299, w287, w281, w284, w283, w279, w277, w275) -> (w297:string[])
            n211 = local write "Current \nRecord"(w297) -> ()
          }
          frame Enabled {
          }
        }
        n212 = local read "Sat Vg Array-Used"() -> (w157:dbl[])
        n213 = local read "New: Dielectric"() -> (w142:dbl)
        n214 = local read "New: Length"() -> (w158:dbl)
        n215 = local read "New: Width"() -> (w160:dbl)
        n216 = local read "Sat Id-Used"() -> (w156:dbl[])
        n217 = local read "Lin-Vg Array-Used"() -> (w151:dbl[])
        n218 = local read "Sat Id-Log-Used"() -> (w155:dbl[])
        n219 = local read "New: Dielectric"() -> (w148:dbl)
        n220 = local read "Vg Array-Log-Used"() -> (w154:dbl[])
        n221 = local read "New: Length"() -> (w150:dbl)
        n222 = local read "New: Width"() -> (w147:dbl)
        n223 = local read "Lin Id-Used"() -> (w152:dbl[])
        n224 = local read "New: Dielectric"() -> (w144:dbl)
        n225 = local read "Lin Vd"() -> (w146:dbl)
        n226 = call "Mobility-Vt-Used Pts_Saturation.vi"("Width"=w160, "Length"=w158, "Dielectric (d)"=w142, "Sat Id Used"=w156, "Vg Used"=w157) -> ("Vt"=w143:dbl, "Mobility"=w159:dbl)  [unwired: 4 in, 1 out]
        n227 = local write "New: Mobility-Sat"(w159) -> ()
        n228 = local write "New: VT-Sat"(w143) -> ()
        n229 = call "Mobility-Vt-Used Pts_Linear.vi"("Width"=w147, "Length"=w150, "Vd"=w146, "Dielectric (d)"=w148, "Id Used"=w152, "Vg Used"=w151) -> ("Vt"=w153:dbl, "Mobility"=w149:dbl)  [unwired: 3 in, 1 out]
        n230 = call "STS-Used.vi"("Id Used"=w155, "Vg-Used"=w154) -> ("STS"=w145:dbl)  [unwired: 9 in]
        n231 = call "Trap Density_VT.vi"("VT"=w143, "Dielectric"=w142) -> ("Trap Density-VT"=w141:dbl)
        n232 = local write "New: Mobility-Lin"(w149) -> ()
        n233 = local write "New: VT-Lin"(w153) -> ()
        n234 = local write "New: STS"(w145) -> ()
        n235 = local write "New: Trap Density-VT"(w141) -> ()
        n236 = local read "Manual-Temp"() -> (w138:bool)
        n237 = local read "Rec: Temp"() -> (w139:dbl)
        n238 = case shown="False" w138 {
          tunnel: w139 -> [w319 _]
          tunnel: [w316 w323] -> w137
          frame False {
            n239 = local read "Rec: Temp"() -> (w317:dbl)
            n240 = property on="New: Temp" class="DigNum (strict)"("DisabledEnum"=1) -> ()  [unwired: 2 in, 2 out]
            n241 = Equal To 0?(x=w317) -> (x = 0?=w318:bool)
            n242 = local write "New: Temp"(w319) -> ()
            n243 = case shown="True" w318 {
              tunnel: [w320 w321] -> w316
              tunnel: w317 -> [w320 _]
              frame False {
              }
              frame True {
                n244 = local read "Room Temp"() -> (w321:dbl)
              }
            }
            n245 = local write "New: Temp"(w316) -> ()
          }
          frame True {
            n246 = property on="New: Temp" class="DigNum (strict)"("DisabledEnum"=0) -> ()  [unwired: 2 in, 2 out]
            n247 = local read "New: Temp"() -> (w323:dbl)
          }
        }
        n248 = call "Trap Density_STS.vi"("Temp (T) [K]"=w137, "S.T.S. (S)"=w145, "Dielectric"=w144) -> ("Trap Density (N)"=w140:dbl)  [unwired: 8 in]
        n249 = local write "New: Trap Density-STS"(w140) -> ()
        n250 = property on="Image Out" class="ImageControl"() -> ("Image Center Position"=w208:cluster{"X":u32, "Y":u32})  [unwired: 2 in, 2 out]
        n251 = property on="Image Out" class="ImageControl"() -> ("ZoomSingle"=w201:cluster{"X":sgl, "Y":sgl})  [unwired: 2 in, 2 out]
        n252 = property on="Image Out" class="ImageControl"() -> ("Bounds"=w202:T14)  [unwired: 2 in, 2 out]
        n253 = Unbundle(w202) -> ("Width"=w199:u32, "Height"=w198:u32)
        n254 = Unbundle(w201) -> ("X"=w176:sgl, "Y"=w200:sgl)
        n255 = event shown="[0] \"Remove Button\": Mouse Down" {
          selector: _ -> [_ _ _ _ _ _ _]
          dyn-events: _ -> [_ _ _ _ _ _ _]
          timeout: 10 -> [_ _ _ _ _ _ _]
          event "Remove Button": Mouse Down {
            w336 = 0
            n256 = event-data() -> ()  [unwired: 1 in, 7 out]
            n257 = property on="Image Out" class="ImageControl"() -> ("ROI"=w334:T15)  [unwired: 2 in, 2 out]
            n258 = Unbundle(w334) -> ("Global Rectangle"=w337:i32[], "Contours"=w339:T16)
            n259 = Reverse 1D Array(array=w337) -> (reversed array=w338:i32[])
            n260 = Reverse 1D Array(array=w339) -> (reversed array=w340:T16)
            n261 = Delete From Array(array=w338, index=w336) -> (array with subset deleted=w341:i32[])  [unwired: 1 in, 1 out]
            n262 = Delete From Array(array=w340, index=w336) -> (array with subset deleted=w342:T16)  [unwired: 1 in, 1 out]
            n263 = Reverse 1D Array(array=w341) -> (reversed array=w343:i32[])
            n264 = Reverse 1D Array(array=w342) -> (reversed array=w344:T16)
            n265 = Bundle(w343, w344) -> (w335:T17)  [unwired: 1 in]
            n266 = local write "ROI Descriptor out"(w334) -> ()
            n267 = local write "ROI Descriptor"(w335) -> ()
            n268 = property on="Image Out" class="ImageControl"("ROI"=w335) -> ()  [unwired: 2 in, 2 out]
          }
          event "Undo Button": Mouse Down {
            n269 = event-data() -> ()  [unwired: 1 in, 7 out]
            n270 = invoke on="Image Out" class="ImageControl" method="Clear ROI"() -> ()  [unwired: 3 in, 3 out]
          }
          event "Image Folder": Value Change {
            n271 = event-data() -> ()  [unwired: 1 in, 5 out]
            n272 = local read "Image File"() -> (w346:path)
            n273 = call "Vision Acquisition"("Image Path"=w346) -> ("Image Out"=w345:T2)  [unwired: 25 in, 1 out]
            n274 = local write "Image Out 2"(w345) -> ()
            n275 = local write "Image Out"(w345) -> ()
            n276 = invoke on="Image Out" class="ImageControl" method="Clear ROI"() -> ()  [unwired: 3 in, 3 out]
          }
          event "Zoom": Value Change {
            n277 = event-data() -> ()  [unwired: 1 in, 5 out]
            n278 = local read "Zoom"() -> (w347:i16)
            n279 = Bundle("Zoom"=w347, "Zoom"=w347) -> (w348:cluster{"Zoom":i16, "Zoom":i16})  [unwired: 1 in]
            n280 = property on="Image Out" class="ImageControl"("ZoomInteger"=w348) -> ()  [unwired: 2 in, 2 out]
          }
          event Timeout {
            n281 = event-data() -> ()  [unwired: 1 in, 2 out]
          }
          event "Image Out": Mouse Enter {
            (unwired) 6
            n282 = event-data() -> ()  [unwired: 1 in, 3 out]
            n283 = call "Simulate_Keyboard.vi"("Action"=0, "Virtual Key"=162) -> ()  [unwired: 7 in, 1 out]
          }
          event "Image Out": Mouse Leave {
            n284 = event-data() -> ()  [unwired: 1 in, 3 out]
            n285 = flat-sequence {
              frame #0 {
                n286 = Wait (ms)(milliseconds to wait=10) -> ()  [unwired: 1 out]
              }
              frame #1 {
                (unwired) 6
                n287 = call "Simulate_Keyboard.vi"("Action"=2, "Virtual Key"=162) -> ()  [unwired: 7 in, 1 out]
              }
            }
          }
        }
        n288 = Divide(x=w199, y=w176) -> (x/y=w189:sgl)
        n289 = Multiply(x=w189, y=0.5) -> (x*y=w195:dbl)
        n290 = Divide(x=w198, y=w200) -> (x/y=w188:sgl)
        n291 = Multiply(x=w188, y=0.5) -> (x*y=w194:dbl)
        n292 = Unbundle(w208) -> ("X"=w190:u32, "Y"=w191:u32)
        n293 = call <vilib>:"Intialize Keyboard.vi"() -> ("device ID"=w213:refnum<k1>)  [unwired: 10 in, 1 out]
        n294 = Subtract(x=w190, y=w195) -> (x-y=w193:dbl)
        n295 = call-poly <vilib>:"Acquire Input Data.vi"("device ID"=w213) -> ("keys pressed"=w212:T18)  [unwired: 16 in, 2 out]
        n296 = Reciprocal(x=w176) -> (1/x=w175:sgl)
        n297 = Index Array(array=w212) -> (element=w216:T19)  [unwired: 1 in]
        n298 = event shown="[1] \"Down Button\": Mouse Down" {
          selector: _ -> [_ _ _ _ _ _ _ _ _ _ _ _ _ _ _ _]
          dyn-events: _ -> [_ _ _ _ _ _ _ _ _ _ _ _ _ _ _ _]
          timeout: 10 -> [_ _ _ _ _ _ _ _ _ _ _ _ _ _ _ _]
          tunnel: [_ _ _ _ _ _ _ _ _ _ _ _ _ TRUE _ TRUE] -> w233
          event Timeout {
            n299 = event-data() -> ()  [unwired: 1 in, 2 out]
          }
          event "Down Button": Mouse Down {
            w713 = 0
            n300 = event-data() -> ()  [unwired: 1 in, 7 out]
            n301 = local read "Transport Style Controls"() -> (w605:T4)
            n302 = local read "Transfer File"() -> (w606:path)
            n303 = Strip Path(path=w606) -> (stripped path=w627:path, name=w724:string)
            n304 = Path To String(path=w627) -> (string=w725:string)
            n305 = call "TRF to TSP Plot.vi"("Transport Graph Properties"=w605, "Transfer File"=w606) -> ("Transport"=w604:cluster{ext[], ext[]}[])  [unwired: 7 in, 2 out]
            n306 = local write "Transfer Folder"(w627) -> ()
            n307 = List Folder(path=w627) -> (filenames=w721:string[], error out=w667:errorcluster)  [unwired: 3 in, 2 out]
            n308 = local write "Transport"(w604) -> ()
            n309 = Array Size(array=w721) -> (size(s)=w717:i32)
            n310 = Search 1D Array(1D array=w721, element=w724) -> (index of element=w718:i32)  [unwired: 1 in]
            n311 = property on="Image Out" class="ImageControl"() -> (error out=w670:errorcluster, "Image Center Position"=w674:cluster{"X":u32, "Y":u32})  [unwired: 2 in, 1 out]
            n312 = Decrement(x=w717) -> (x-1=w719:i32)
            n313 = local read "Folder Index"() -> (w669:dbl)
            n314 = Equal?(x=w718, y=w719) -> (x = y?=w720:bool)
            n315 = Unbundle(w674) -> ("X"=w672:u32)  [unwired: 1 out]
            n316 = case shown="False" w720 {
              tunnel: w669 -> [w877 _]
              tunnel: [w876 0] -> w668
              tunnel: w667 -> [w875 w878]
              tunnel: [w875 w878] -> w666
              frame False {
                n317 = Increment(x=w877) -> (x+1=w876:dbl)
              }
              frame True {
              }
            }
            n318 = Index Array(array=w721, index=w668) -> (element=w628:string)
            n319 = local write "Data Name:"(w628) -> ()
            n320 = local write "Folder Index"(w668) -> ()
            n321 = Bundle("X"=w672, 0) -> (w673:cluster{"X":u32, i32})  [unwired: 1 in]
            n322 = Concatenate Strings(w725, "\\", w628) -> (w723:string)
            n323 = property on="Image Out" class="ImageControl"(error in=w670, "Image Center Position"=w673) -> ()  [unwired: 1 in, 2 out]
            n324 = String To Path(string=w723) -> (path=w641:path)
            n325 = call "Recorded Values.vi"("Path"=w641) -> ("Recorded Char"=w727:T7, "Recorded Prop"=w728:T8, "Fabrication Prop"=w726:T9)  [unwired: 8 in]
            n326 = Unbundle By Name(w727) -> ("Mobility-Sat"=w740:dbl, "Moblitity-Lin"=w741:dbl, "On/Off"=w742:dbl, "Off Current"=w743:dbl, "Vt-Sat"=w636:dbl, "STS"=w744:dbl, "Trap Density-VT"=w745:dbl, "Trap Density-STS"=w746:dbl)
            n327 = Unbundle By Name(w726) -> ("Date Created"=w747:string, "Material"=w729:string, "Solvent"=w730:string, "Concentration"=w731:dbl, "Method"=w732:string, "Dielectric (nm)"=w733:dbl, "Treatment"=w734:string, "Comments"=w735:string)
            n328 = Unbundle By Name(w728) -> ("Date Recorded"=w736:string, "Index"=w737:string, "Length"=w738:dbl, "Width"=w739:dbl, "Sample Temp"=w638:dbl)
            n329 = local write "Date Created"(w747) -> ()
            n330 = local write "Rec: Off I-Sat"(w743) -> ()
            n331 = local write "Rec: Comments"(w735) -> ()
            n332 = local write "Rec: Material"(w729) -> ()
            n333 = local write "Rec: VT-Sat"(w636) -> ()
            n334 = local write "Rec: Concentration"(w731) -> ()
            n335 = local write "Rec: Method"(w732) -> ()
            n336 = local write "Rec: Dielectric (d)"(w733) -> ()
            n337 = local write "Surface Treatment:"(w734) -> ()
            n338 = local write "Index"(w737) -> ()
            n339 = local write "Rec: Mobility-Sat"(w740) -> ()
            n340 = local write "Rec: Mobility-Lin"(w741) -> ()
            n341 = local write "Rec: On/Off"(w742) -> ()
            n342 = local write "Rec: STS"(w744) -> ()
            n343 = local write "Rec: Trap Density-VT"(w745) -> ()
            n344 = local write "Rec: Trap Density-STS"(w746) -> ()
            n345 = local write "Rec: Solvent"(w730) -> ()
            n346 = local write "Date Recorded"(w736) -> ()
            n347 = local write "Rec: Length"(w738) -> ()
            n348 = local write "Rec: Width"(w739) -> ()
            n349 = local write "Rec: Temp"(w638) -> ()
            n350 = Equal To 0?(x=w638) -> (x = 0?=w639:bool)
            n351 = case shown="True" w639 {
              tunnel: [w748 w749] -> w637
              tunnel: w638 -> [w748 _]
              frame False {
              }
              frame True {
                n352 = local read "Room Temp"() -> (w749:dbl)
              }
            }
            n353 = invoke on="Image Out" class="ImageControl" method="Clear ROI"() -> ()  [unwired: 3 in, 3 out]
            n354 = local read "NumPoints Log"() -> (w662:dbl)
            n355 = local write "Transfer File"(w641) -> ()
            n356 = local read "Num Pts"() -> (w665:dbl)
            n357 = call-poly <vilib>:"Read From Spreadsheet File.vi"("file path (dialog if empty)"=w641) -> ("all rows"=w610:string[][])  [unwired: 6 in, 4 out]
            n358 = call "Mobility-Vt Calculator-File.vi"("NumPts"=w665, "Path"=w641) -> ("Graph Cluster"=w634:T11, "Output"=w664:T12, 4:w663, 5:w649)  [unwired: 4 in, 2 out]
            n359 = local read "New: Dielectric"() -> (w646:dbl)
            n360 = call "STS Calculator-File.vi"("NumPts"=w662, "Path"=w641) -> ("Used Points"=w661:T10, "XY Graph-Sat"=w660:cluster{dbl[], dbl[]}[], "Ouput"=w659:cluster{"STS-Sat":dbl, "STS-Lin":dbl})  [unwired: 6 in, 1 out]
            n361 = local write "Index 2"(w661) -> ()
            n362 = local write "Sat-Trans Slider"(w663) -> ()
            n363 = Array Size(array=w610) -> (size(s)=w714:i32[])
            n364 = Unbundle By Name(w664) -> ("Mobility-Sat"=w658:dbl, "Vt-Sat"=w645:dbl, "Mobility-Lin"=w657:dbl, "Vt-Lin"=w656:dbl, "Off I-Sat"=w642:dbl, "On/Off I-Sat"=w635:dbl)
            n365 = Unbundle By Name(w659) -> ("STS-Sat"=w640:dbl)  [unwired: 1 out]
            n366 = local write "MobVi Index"(w663) -> ()
            n367 = local write "Sat-Log"(w660) -> ()
            n368 = Unbundle By Name(w634) -> ("Raw Sat"=w631:cluster{dbl[], dbl[]}[], "Sqrt Sat"=w633:cluster{dbl[], dbl[]}[], "Raw Lin"=w630:cluster{dbl[], dbl[]}[], "Sqrt Lin"=w632:cluster{dbl[], dbl[]}[], "Log Lin"=w629:cluster{dbl[], dbl[]}[])  [unwired: 1 out]
            n369 = local write "Sqrt-Sat"(w633) -> ()
            n370 = call "Trap Density_VT.vi"("VT"=w645, "Dielectric"=w646) -> ("Trap Density-VT"=w644:dbl)
            n371 = Index Array(array=w714, index=0) -> (element=w698:i32)
            n372 = call "Trap Density_STS.vi"("Temp (T) [K]"=w637, "S.T.S. (S)"=w640, "Dielectric"=w646) -> ("Trap Density (N)"=w643:dbl)  [unwired: 8 in]
            n373 = local write "New: STS"(w640) -> ()
            n374 = local write "Calc: STS"(w640) -> ()
            n375 = local write "Calc: Mobility-Sat"(w658) -> ()
            n376 = local write "Calc: Off I-Sat"(w656) -> ()
            n377 = local write "Calc: Mobility-Lin"(w657) -> ()
            n378 = Decimate 1D Array(w660) -> (w693:cluster{dbl[], dbl[]}[])  [unwired: 1 out]
            n379 = Decimate 1D Array(w633) -> (w701:cluster{dbl[], dbl[]}[])  [unwired: 1 out]
            n380 = local write "Calc: Off I-Sat"(w642) -> ()
            n381 = local write "Calc: On/Off"(w635) -> ()
            n382 = Decimate 1D Array(w632) -> (w655:cluster{dbl[], dbl[]}[])  [unwired: 1 out]
            n383 = local write "Calc: VT-Sat"(w645) -> ()
            n384 = Array Subset(array=w610, index (row)=w713, index (col)=w713, length (col)=3) -> (w715:string[][])  [unwired: 1 in]
            n385 = local write "Calc: Trap Density-VT"(w644) -> ()
            n386 = local write "Calc: Trap Density-STS"(w643) -> ()
            n387 = local write "New: Trap Density-STS"(w643) -> ()
            n388 = local write "New: Trap Density-VT"(w644) -> ()
            n389 = Array To Cluster(array=w693) -> (cluster=w691:T13)
            n390 = Array To Cluster(array=w701) -> (cluster=w703:T13)
            n391 = local write "Raw- Sat"(w631) -> ()
            n392 = local write "Sqrt-Lin"(w632) -> ()
            n393 = local write "Raw- Lin"(w630) -> ()
            n394 = local write "New: VT-Lin"(w656) -> ()
            n395 = local write "Log-Lin"(w629) -> ()
            n396 = local write "New: VT-Sat"(w645) -> ()
            n397 = local write "New: Mobility-Sat"(w658) -> ()
            n398 = local write "New: Mobility-Lin"(w657) -> ()
            n399 = Reshape Array(w715, w698) -> (w612:string[])
            n400 = Search 1D Array(1D array=w612, element="Vg") -> (index of element=w616:i32)  [unwired: 1 in]
            n401 = Add(x=w616, y=3) -> (x+y=w614:i32)
            n402 = Divide(x=w614, y=3) -> (x/y=w621:dbl)
            n403 = Array Subset(array=w610, index (row)=w621, index (col)=0, length (col)=1) -> (w620:string[][])  [unwired: 1 in]
            n404 = Fract/Exp String To Number(string=w620) -> (number=w624:dbl[][])  [unwired: 3 in, 1 out]
            n405 = Array Size(array=w624) -> (size(s)=w611:i32[])
            n406 = Index Array(array=w611, index=0) -> (element=w622:i32)
            n407 = Decrement(x=w622) -> (x-1=w625:i32)
            n408 = Reshape Array(w624, w625) -> (w609:dbl[])
            n409 = local write "Data Length"(w625) -> ()
            n410 = local write "Vg Column"(w609) -> ()
            n411 = Array To Cluster(array=w655) -> (cluster=w654:T13)
            n412 = Array Max & Min(array=w609) -> (max value=w608:dbl, min value=w607:dbl)  [unwired: 2 out]
            n413 = Unbundle(w691) -> ("[0]"=w692:cluster{dbl[], dbl[]})  [unwired: 8 out]
            n414 = Unbundle(w703) -> ("[0]"=w702:cluster{dbl[], dbl[]})  [unwired: 8 out]
            n415 = Unbundle(w654) -> ("[0]"=w651:cluster{dbl[], dbl[]})  [unwired: 8 out]
            n416 = Search 1D Array(1D array=w612, element="Index:") -> (index of element=w710:i32)  [unwired: 1 in]
            n417 = property on="Sat-Trans Slider" class="Slide (strict)"("Scale.Maximum"=w608, "Scale.Minimum"=w607) -> ()  [unwired: 2 in, 2 out]
            n418 = local read "Num Pts"() -> (w650:dbl)
            n419 = Unbundle(w651) -> (w653:dbl[], w652:dbl[])
            n420 = Increment(x=w710) -> (x+1=w711:i32)
            n421 = Unbundle(w692) -> (w690:dbl[], w689:dbl[])
            n422 = Unbundle(w702) -> (w695:dbl[], w694:dbl[])
            n423 = Array Subset(array=w653, index=w649, length=w650) -> (w648:dbl[])
            n424 = Array Subset(array=w652, index=w649, length=w650) -> (w647:dbl[])
            n425 = Array Subset(array=w690, index=w661, length=w662) -> (w697:dbl[])
            n426 = Array Subset(array=w689, index=w661, length=w662) -> (w696:dbl[])
            n427 = Array Subset(array=w695, index=w663, length=w665) -> (w700:dbl[])
            n428 = Array Subset(array=w694, index=w663, length=w665) -> (w699:dbl[])
            n429 = Index Array(array=w612, index=w711) -> (element=w678:string)
            n430 = local write "Lin-Vg Array-Used"(w648) -> ()
            n431 = local write "Sat Vg Array-Used"(w700) -> ()
            n432 = local write "Vg Array-Log-Used"(w696) -> ()
            n433 = local write "Lin Id-Used"(w647) -> ()
            n434 = local read "Image Folder"() -> (w676:path)
            n435 = local write "Sat Id-Used"(w699) -> ()
            n436 = local write "Sat Id-Log-Used"(w697) -> ()
            n437 = List Folder(path=w676, error in=w666) -> (filenames=w709:string[], error out=w679:errorcluster)  [unwired: 2 in, 2 out]
            n438 = while {
              tunnel: w709 -> [w762]
              tunnel: w678 -> [w760]
              tunnel: [w759] -> _
              tunnel: [w759] -> w708
              tunnel: w698 -> [w758]
              i -> [w759]
              stop <- w755 stop-if-true
              n439 = Index Array(array=w762, index=w759) -> (element=w763:string)
              n440 = xnode "Match Regular Expression"("input string"=w763, "regular expression"=w760) -> ("whole match"=w761:string)  [unwired: 4 in, 4 out]
              n441 = Equal?(x=w761, y=w760) -> (x = y?=w757:bool)
              n442 = Equal?(x=w758, y=w759) -> (x = y?=w756:bool)
              n443 = Or(x=w757, y=w756) -> (x .or. y?=w755:bool)
            }
            n444 = Build Path(base path=w676, name or relative path="ROI") -> (appended path=w675:path)
            n445 = Path To String(path=w676) -> (string=w706:string)
            n446 = Index Array(array=w709, index=w708) -> (element=w687:string)
            n447 = invoke on="Image Out" class="ImageControl" method="Clear ROI"(error in=w679) -> (error out=w682:errorcluster)  [unwired: 2 in, 2 out]
            n448 = local write "Image Name"(w687) -> ()
            n449 = Build Path(base path=w675, name or relative path=w678) -> (appended path=w683:path)
            n450 = call <vilib>:"Check if File or Folder Exists.vi"("error in (no error)"=w682, "path"=w683) -> ("file or folder exists?"=w680:bool, "dup path"=w681:path)  [unwired: 7 in, 1 out]
            n451 = Concatenate Strings(w706, "\\", w687) -> (w705:string)
            n452 = case shown="False" w680 {
              tunnel: w681 -> [_ w750]
              frame False {
              }
              frame True {
                n453 = Read from Text File(file (use dialog)=w750) -> (text=w754:string)  [unwired: 3 in, 3 out]
                n454 = property on="Image Out" class="ImageControl"() -> ("ROI"=w751:T15)  [unwired: 2 in, 2 out]
                n455 = Unflatten From String(type=w751, binary string=w754) -> (value=w752:T15, error out=w753:errorcluster)  [unwired: 3 in, 1 out]
                n456 = property on="Image Out" class="ImageControl"(error in=w753, "ROI"=w752) -> ()  [unwired: 1 in, 2 out]
              }
            }
            n457 = String To Path(string=w705) -> (path=w686:path)
            n458 = Empty String/Path?(string/path=w687) -> (empty?=w688:bool)
            n459 = local read "No Image File"() -> (w684:path)
            n460 = Select(t=w684, s=w688, f=w686) -> (s? t:f=w685:path)
            n461 = local write "Image File"(w685) -> ()
            n462 = call "Vision Acquisition4"("Image Path"=w685) -> ("Image Out"=w707:T2)  [unwired: 25 in, 1 out]
            n463 = local write "Image Out"(w707) -> ()
            n464 = local write "Image Out 2"(w707) -> ()
          }
          event "Transfer File": Value Change {
            w905 = 0
            w1016 = 0
            n465 = event-data() -> ()  [unwired: 1 in, 5 out]
            n466 = local read "Transfer File"() -> (w882:path)
            n467 = local read "Transport Style Controls"() -> (w881:T4)
            n468 = Strip Path(path=w882) -> (stripped path=w909:path, name=w1024:string)
            n469 = call "TRF to TSP Plot.vi"("Transport Graph Properties"=w881, "Transfer File"=w882) -> ("Transport"=w880:cluster{ext[], ext[]}[])  [unwired: 7 in, 2 out]
            n470 = local write "Transfer Folder"(w909) -> ()
            n471 = local write "Transport"(w880) -> ()
            n472 = property on="Image Out" class="ImageControl"() -> (error out=w971:errorcluster, "Image Center Position"=w975:cluster{"X":u32, "Y":u32})  [unwired: 2 in, 1 out]
            n473 = List Folder(path=w909) -> (filenames=w1021:string[], error out=w981:errorcluster)  [unwired: 3 in, 2 out]
            n474 = Search 1D Array(1D array=w1021, element=w1024) -> (index of element=w970:i32)  [unwired: 1 in]
            n475 = local write "Folder Index"(w970) -> ()
            n476 = Unbundle(w975) -> ("X"=w973:u32)  [unwired: 1 out]
            n477 = Path To String(path=w909) -> (string=w1025:string)
            n478 = Index Array(array=w1021, index=w970) -> (element=w910:string)
            n479 = Bundle("X"=w973, 0) -> (w974:cluster{"X":u32, i32})  [unwired: 1 in]
            n480 = local write "Data Name:"(w910) -> ()
            n481 = property on="Image Out" class="ImageControl"(error in=w971, "Image Center Position"=w974) -> ()  [unwired: 1 in, 2 out]
            n482 = Concatenate Strings(w1025, "\\", w910) -> (w1023:string)
            n483 = String To Path(string=w1023) -> (path=w883:path)
            n484 = call "Recorded Values.vi"("Path"=w883) -> ("Recorded Char"=w968:T7, "Recorded Prop"=w967:T8, "Fabrication Prop"=w969:T9)  [unwired: 8 in]
            n485 = Unbundle By Name(w968) -> ("Mobility-Sat"=w955:dbl, "Moblitity-Lin"=w954:dbl, "On/Off"=w953:dbl, "Off Current"=w952:dbl, "Vt-Sat"=w919:dbl, "STS"=w951:dbl, "Trap Density-VT"=w950:dbl, "Trap Density-STS"=w949:dbl)
            n486 = Unbundle By Name(w969) -> ("Date Created"=w948:string, "Material"=w966:string, "Solvent"=w965:string, "Concentration"=w964:dbl, "Method"=w963:string, "Dielectric (nm)"=w962:dbl, "Treatment"=w961:string, "Comments"=w960:string)
            n487 = Unbundle By Name(w967) -> ("Date Recorded"=w959:string, "Index"=w958:string, "Length"=w957:dbl, "Width"=w956:dbl, "Sample Temp"=w921:dbl)
            n488 = local write "Date Created"(w948) -> ()
            n489 = local write "Rec: Material"(w966) -> ()
            n490 = local write "Rec: Off I-Sat"(w952) -> ()
            n491 = local write "Rec: Comments"(w960) -> ()
            n492 = local write "Rec: VT-Sat"(w919) -> ()
            n493 = local write "Rec: Concentration"(w964) -> ()
            n494 = local write "Rec: Method"(w963) -> ()
            n495 = local write "Rec: Dielectric (d)"(w962) -> ()
            n496 = local write "Surface Treatment:"(w961) -> ()
            n497 = local write "Index"(w958) -> ()
            n498 = local write "Rec: Mobility-Sat"(w955) -> ()
            n499 = local write "Rec: Mobility-Lin"(w954) -> ()
            n500 = local write "Rec: On/Off"(w953) -> ()
            n501 = local write "Rec: STS"(w951) -> ()
            n502 = local write "Rec: Trap Density-VT"(w950) -> ()
            n503 = local write "Rec: Trap Density-STS"(w949) -> ()
            n504 = local write "Rec: Solvent"(w965) -> ()
            n505 = local write "Date Recorded"(w959) -> ()
            n506 = local write "Rec: Length"(w957) -> ()
            n507 = local write "Rec: Width"(w956) -> ()
            n508 = local write "Rec: Temp"(w921) -> ()
            n509 = Equal To 0?(x=w921) -> (x = 0?=w922:bool)
            n510 = case shown="True" w922 {
              tunnel: [w1026 w1027] -> w920
              tunnel: w921 -> [w1026 _]
              frame False {
              }
              frame True {
                n511 = local read "Room Temp"() -> (w1027:dbl)
              }
            }
            n512 = local read "NumPoints Log"() -> (w944:dbl)
            n513 = local write "Transfer File"(w883) -> ()
            n514 = local read "Num Pts"() -> (w945:dbl)
            n515 = call-poly <vilib>:"Read From Spreadsheet File.vi"("file path (dialog if empty)"=w883) -> ("all rows"=w1018:string[][])  [unwired: 6 in, 4 out]
            n516 = local read "New: Dielectric"() -> (w928:dbl)
            n517 = call "STS Calculator-File.vi"("NumPts"=w944, "Path"=w883) -> ("Used Points"=w942:T10, "XY Graph-Sat"=w943:cluster{dbl[], dbl[]}[], "Ouput"=w941:cluster{"STS-Sat":dbl, "STS-Lin":dbl})  [unwired: 6 in, 1 out]
            n518 = call "Mobility-Vt Calculator-File.vi"("NumPts"=w945, "Path"=w883) -> ("Graph Cluster"=w916:T11, "Output"=w946:T12, 4:w947, 5:w934)  [unwired: 4 in, 2 out]
            n519 = Unbundle By Name(w946) -> ("Mobility-Sat"=w930:dbl, "Vt-Sat"=w924:dbl, "Mobility-Lin"=w929:dbl, "Vt-Lin"=w917:dbl, "Off I-Sat"=w923:dbl, "On/Off I-Sat"=w918:dbl)
            n520 = local write "Index 2"(w942) -> ()
            n521 = Unbundle By Name(w941) -> ("STS-Sat"=w925:dbl)  [unwired: 1 out]
            n522 = local write "MobVi Index"(w947) -> ()
            n523 = local write "Sat-Log"(w943) -> ()
            n524 = local write "Sat-Trans Slider"(w947) -> ()
            n525 = Array Size(array=w1018) -> (size(s)=w1017:i32[])
            n526 = call "Trap Density_VT.vi"("VT"=w924, "Dielectric"=w928) -> ("Trap Density-VT"=w927:dbl)
            n527 = call "Trap Density_STS.vi"("Temp (T) [K]"=w920, "S.T.S. (S)"=w925, "Dielectric"=w928) -> ("Trap Density (N)"=w926:dbl)  [unwired: 8 in]
            n528 = local write "Calc: Mobility-Lin"(w929) -> ()
            n529 = local write "Calc: Mobility-Sat"(w930) -> ()
            n530 = local write "Calc: VT-Sat"(w924) -> ()
            n531 = local write "Calc: Off I-Sat"(w923) -> ()
            n532 = local write "Calc: VT-Lin"(w917) -> ()
            n533 = local write "Calc: On/Off"(w918) -> ()
            n534 = local write "Calc: STS"(w925) -> ()
            n535 = Unbundle By Name(w916) -> ("Raw Sat"=w913:cluster{dbl[], dbl[]}[], "Sqrt Sat"=w914:cluster{dbl[], dbl[]}[], "Raw Lin"=w912:cluster{dbl[], dbl[]}[], "Sqrt Lin"=w915:cluster{dbl[], dbl[]}[], "Log Lin"=w911:cluster{dbl[], dbl[]}[])  [unwired: 1 out]
            n536 = Decimate 1D Array(w915) -> (w940:cluster{dbl[], dbl[]}[])  [unwired: 1 out]
            n537 = local write "Calc: Trap Density-VT"(w927) -> ()
            n538 = local write "Calc: Trap Density-STS"(w926) -> ()
            n539 = local write "New: Trap Density-STS"(w926) -> ()
            n540 = local write "New: Trap Density-VT"(w927) -> ()
            n541 = local write "Sqrt-Lin"(w915) -> ()
            n542 = local write "New: VT-Sat"(w924) -> ()
            n543 = Decimate 1D Array(w943) -> (w996:cluster{dbl[], dbl[]}[])  [unwired: 1 out]
            n544 = Index Array(array=w1017, index=w1016) -> (element=w1000:i32)
            n545 = Decimate 1D Array(w914) -> (w1003:cluster{dbl[], dbl[]}[])  [unwired: 1 out]
            n546 = local write "Sqrt-Sat"(w914) -> ()
            n547 = local write "New: Mobility-Lin"(w929) -> ()
            n548 = Array Subset(array=w1018, index (row)=w1016, index (col)=w1016, length (col)=3) -> (w1019:string[][])  [unwired: 1 in]
            n549 = local write "New: VT-Lin"(w917) -> ()
            n550 = Array To Cluster(array=w940) -> (cluster=w939:T13)
            n551 = local write "New: STS"(w925) -> ()
            n552 = local write "New: Mobility-Sat"(w930) -> ()
            n553 = Array To Cluster(array=w996) -> (cluster=w994:T13)
            n554 = Array To Cluster(array=w1003) -> (cluster=w1005:T13)
            n555 = Reshape Array(w1019, w1000) -> (w1006:string[])
            n556 = local write "Raw- Sat"(w913) -> ()
            n557 = Unbundle(w939) -> ("[0]"=w938:cluster{dbl[], dbl[]})  [unwired: 8 out]
            n558 = local write "Raw- Lin"(w912) -> ()
            n559 = local read "Num Pts"() -> (w935:dbl)
            n560 = local write "Log-Lin"(w911) -> ()
            n561 = Unbundle(w938) -> (w937:dbl[], w936:dbl[])
            n562 = Unbundle(w994) -> ("[0]"=w995:cluster{dbl[], dbl[]})  [unwired: 8 out]
            n563 = Unbundle(w1005) -> ("[0]"=w1004:cluster{dbl[], dbl[]})  [unwired: 8 out]
            n564 = Search 1D Array(1D array=w1006, element="Index:") -> (index of element=w1013:i32)  [unwired: 1 in]
            n565 = local read "Num Pts"() -> (w931:dbl)
            n566 = Array Subset(array=w937, index=w934, length=w935) -> (w933:dbl[])
            n567 = Array Subset(array=w936, index=w934, length=w935) -> (w932:dbl[])
            n568 = Increment(x=w1013) -> (x+1=w1014:i32)
            n569 = Unbundle(w995) -> (w992:dbl[], w991:dbl[])
            n570 = Unbundle(w1004) -> (w993:dbl[], w997:dbl[])
            n571 = local read "Image Folder"() -> (w977:path)
            n572 = local write "Lin-Vg Array-Used"(w933) -> ()
            n573 = Array Subset(array=w992, index=w942, length=w944) -> (w999:dbl[])
            n574 = Array Subset(array=w991, index=w942, length=w944) -> (w998:dbl[])
            n575 = Array Subset(array=w993, index=w947, length=w931) -> (w1002:dbl[])
            n576 = Array Subset(array=w997, index=w947, length=w931) -> (w1001:dbl[])
            n577 = Index Array(array=w1006, index=w1014) -> (element=w979:string)
            n578 = local write "Lin Id-Used"(w932) -> ()
            n579 = local write "Sat Vg Array-Used"(w1002) -> ()
            n580 = local write "Vg Array-Log-Used"(w998) -> ()
            n581 = local write "Sat Id-Log-Used"(w999) -> ()
            n582 = local write "Sat Id-Used"(w1001) -> ()
            n583 = local write "Index"(w979) -> ()
            n584 = List Folder(path=w977, error in=w981) -> (filenames=w1011:string[], error out=w980:errorcluster)  [unwired: 2 in, 2 out]
            n585 = Build Path(base path=w977, name or relative path="ROI") -> (appended path=w976:path)
            n586 = invoke on="Image Out" class="ImageControl" method="Clear ROI"(error in=w980) -> (error out=w984:errorcluster)  [unwired: 2 in, 2 out]
            n587 = Build Path(base path=w976, name or relative path=w979) -> (appended path=w985:path)
            n588 = while {
              tunnel: w1011 -> [w1040]
              tunnel: w979 -> [w1038]
              tunnel: [w1037] -> _
              tunnel: [w1037] -> w1010
              tunnel: w1000 -> [w1036]
              i -> [w1037]
              stop <- w1033 stop-if-true
              n589 = Index Array(array=w1040, index=w1037) -> (element=w1041:string)
              n590 = xnode "Match Regular Expression"("input string"=w1041, "regular expression"=w1038) -> ("whole match"=w1039:string)  [unwired: 4 in, 4 out]
              n591 = Equal?(x=w1039, y=w1038) -> (x = y?=w1035:bool)
              n592 = Equal?(x=w1036, y=w1037) -> (x = y?=w1034:bool)
              n593 = Or(x=w1035, y=w1034) -> (x .or. y?=w1033:bool)
            }
            n594 = call <vilib>:"Check if File or Folder Exists.vi"("error in (no error)"=w984, "path"=w985) -> ("file or folder exists?"=w982:bool, "dup path"=w983:path)  [unwired: 7 in, 1 out]
            n595 = case shown="True" w982 {
              tunnel: w983 -> [_ w1028]
              frame False {
              }
              frame True {
                n596 = Read from Text File(file (use dialog)=w1028) -> (text=w1032:string)  [unwired: 3 in, 3 out]
                n597 = property on="Image Out" class="ImageControl"() -> ("ROI"=w1029:T15)  [unwired: 2 in, 2 out]
                n598 = Unflatten From String(type=w1029, binary string=w1032) -> (value=w1030:T15, error out=w1031:errorcluster)  [unwired: 3 in, 1 out]
                n599 = property on="Image Out" class="ImageControl"(error in=w1031, "ROI"=w1030) -> ()  [unwired: 1 in, 2 out]
              }
            }
            n600 = invoke on="Image Out" class="ImageControl" method="Clear ROI"() -> ()  [unwired: 3 in, 3 out]
            n601 = call-poly <vilib>:"Read From Spreadsheet File.vi"("file path (dialog if empty)"=w883) -> ("all rows"=w887:string[][])  [unwired: 6 in, 4 out]
            n602 = Array Size(array=w887) -> (size(s)=w906:i32[])
            n603 = Index Array(array=w906, index=0) -> (element=w904:i32)
            n604 = Path To String(path=w977) -> (string=w1009:string)
            n605 = Index Array(array=w1011, index=w1010) -> (element=w989:string)
            n606 = Concatenate Strings(w1009, "\\", w989) -> (w1008:string)
            n607 = Array Subset(array=w887, index (row)=w905, index (col)=w905, length (col)=3) -> (w907:string[][])  [unwired: 1 in]
            n608 = local write "Image Name"(w989) -> ()
            n609 = String To Path(string=w1008) -> (path=w988:path)
            n610 = Empty String/Path?(string/path=w989) -> (empty?=w990:bool)
            n611 = local read "No Image File"() -> (w986:path)
            n612 = Reshape Array(w907, w904) -> (w889:string[])
            n613 = Search 1D Array(1D array=w889, element="Vg") -> (index of element=w893:i32)  [unwired: 1 in]
            n614 = Add(x=w893, y=3) -> (x+y=w891:i32)
            n615 = Divide(x=w891, y=3) -> (x/y=w898:dbl)
            n616 = Array Subset(array=w887, index (row)=w898, index (col)=0, length (col)=1) -> (w897:string[][])  [unwired: 1 in]
            n617 = Fract/Exp String To Number(string=w897) -> (number=w901:dbl[][])  [unwired: 3 in, 1 out]
            n618 = Array Size(array=w901) -> (size(s)=w888:i32[])
            n619 = Index Array(array=w888, index=0) -> (element=w899:i32)
            n620 = Decrement(x=w899) -> (x-1=w902:i32)
            n621 = Reshape Array(w901, w902) -> (w886:dbl[])
            n622 = local write "Data Length"(w902) -> ()
            n623 = local write "Vg Column"(w886) -> ()
            n624 = Select(t=w986, s=w990, f=w988) -> (s? t:f=w987:path)
            n625 = local write "Image File"(w987) -> ()
            n626 = Array Max & Min(array=w886) -> (max value=w885:dbl, min value=w884:dbl)  [unwired: 2 out]
            n627 = property on="Sat-Trans Slider" class="Slide (strict)"("Scale.Maximum"=w885, "Scale.Minimum"=w884) -> ()  [unwired: 2 in, 2 out]
            n628 = call "Vision Acquisition3"("Image Path"=w987) -> ("Image Out"=w1012:T2)  [unwired: 25 in, 1 out]
            n629 = local write "Image Out"(w1012) -> ()
            n630 = local write "Image Out 2"(w1012) -> ()
          }
          event "Up Button": Mouse Down {
            w1178 = 0
            w1292 = 0
            n631 = event-data() -> ()  [unwired: 1 in, 5 out]
            n632 = local read "Transfer File"() -> (w1155:path)
            n633 = Strip Path(path=w1155) -> (stripped path=w1182:path, name=w1302:string)
            n634 = local read "Transport Style Controls"() -> (w1154:T4)
            n635 = local write "Transfer Folder"(w1182) -> ()
            n636 = List Folder(path=w1182) -> (filenames=w1297:string[], error out=w1256:errorcluster)  [unwired: 3 in, 2 out]
            n637 = Array Size(array=w1297) -> (size(s)=w1244:i32)
            n638 = Search 1D Array(1D array=w1297, element=w1302) -> (index of element=w1298:i32)  [unwired: 1 in]
            n639 = call "TRF to TSP Plot.vi"("Transport Graph Properties"=w1154, "Transfer File"=w1155) -> ("Transport"=w1153:cluster{ext[], ext[]}[])  [unwired: 7 in, 2 out]
            n640 = Equal To 0?(x=w1298) -> (x = 0?=w1299:bool)
            n641 = local write "Transport"(w1153) -> ()
            n642 = local read "Folder Index"() -> (w1243:dbl)
            n643 = property on="Image Out" class="ImageControl"() -> (error out=w1246:errorcluster, "Image Center Position"=w1250:cluster{"X":u32, "Y":u32})  [unwired: 2 in, 1 out]
            n644 = case shown="True" w1299 {
              tunnel: w1243 -> [w1432 _]
              tunnel: [w1431 w1433] -> w1242
              tunnel: w1244 -> [_ w1434]
              frame False {
                n645 = Decrement(x=w1432) -> (x-1=w1431:dbl)
              }
              frame True {
                n646 = Decrement(x=w1434) -> (x-1=w1433:i32)
              }
            }
            n647 = Unbundle(w1250) -> ("X"=w1248:u32)  [unwired: 1 out]
            n648 = local write "Folder Index"(w1242) -> ()
            n649 = Bundle("X"=w1248, 0) -> (w1249:cluster{"X":u32, i32})  [unwired: 1 in]
            n650 = Path To String(path=w1182) -> (string=w1303:string)
            n651 = Index Array(array=w1297, index=w1242) -> (element=w1183:string)
            n652 = local write "Data Name:"(w1183) -> ()
            n653 = property on="Image Out" class="ImageControl"(error in=w1246, "Image Center Position"=w1249) -> ()  [unwired: 1 in, 2 out]
            n654 = Concatenate Strings(w1303, "\\", w1183) -> (w1301:string)
            n655 = String To Path(string=w1301) -> (path=w1156:path)
            n656 = call "Recorded Values.vi"("Path"=w1156) -> ("Recorded Char"=w1240:T7, "Recorded Prop"=w1239:T8, "Fabrication Prop"=w1241:T9)  [unwired: 8 in]
            n657 = Unbundle By Name(w1240) -> ("Mobility-Sat"=w1227:dbl, "Moblitity-Lin"=w1226:dbl, "On/Off"=w1225:dbl, "Off Current"=w1224:dbl, "Vt-Sat"=w1191:dbl, "STS"=w1223:dbl, "Trap Density-VT"=w1222:dbl, "Trap Density-STS"=w1221:dbl)
            n658 = Unbundle By Name(w1241) -> ("Date Created"=w1220:string, "Material"=w1238:string, "Solvent"=w1237:string, "Concentration"=w1236:dbl, "Method"=w1235:string, "Dielectric (nm)"=w1234:dbl, "Treatment"=w1233:string, "Comments"=w1232:string)
            n659 = Unbundle By Name(w1239) -> ("Date Recorded"=w1231:string, "Index"=w1230:string, "Length"=w1229:dbl, "Width"=w1228:dbl, "Sample Temp"=w1192:dbl)
            n660 = local write "Date Created"(w1220) -> ()
            n661 = local write "Rec: Material"(w1238) -> ()
            n662 = local write "Rec: Off I-Sat"(w1224) -> ()
            n663 = local write "Rec: Comments"(w1232) -> ()
            n664 = local write "Rec: VT-Sat"(w1191) -> ()
            n665 = local write "Rec: Solvent"(w1237) -> ()
            n666 = local write "Rec: Concentration"(w1236) -> ()
            n667 = local write "Rec: Method"(w1235) -> ()
            n668 = local write "Rec: Dielectric (d)"(w1234) -> ()
            n669 = local write "Surface Treatment:"(w1233) -> ()
            n670 = local write "Index"(w1230) -> ()
            n671 = local write "Rec: Mobility-Sat"(w1227) -> ()
            n672 = local write "Rec: Mobility-Lin"(w1226) -> ()
            n673 = local write "Rec: On/Off"(w1225) -> ()
            n674 = local write "Rec: STS"(w1223) -> ()
            n675 = local write "Rec: Trap Density-VT"(w1222) -> ()
            n676 = local write "Rec: Trap Density-STS"(w1221) -> ()
            n677 = local write "Date Recorded"(w1231) -> ()
            n678 = local write "Rec: Length"(w1229) -> ()
            n679 = local write "Rec: Width"(w1228) -> ()
            n680 = local write "Rec: Temp"(w1192) -> ()
            n681 = Equal To 0?(x=w1192) -> (x = 0?=w1194:bool)
            n682 = case shown="False" w1194 {
              tunnel: [w1304 w1305] -> w1193
              tunnel: w1192 -> [w1304 _]
              frame False {
              }
              frame True {
                n683 = local read "Room Temp"() -> (w1305:dbl)
              }
            }
            n684 = local read "NumPoints Log"() -> (w1216:dbl)
            n685 = local write "Transfer File"(w1156) -> ()
            n686 = local read "Num Pts"() -> (w1219:dbl)
            n687 = local read "New: Dielectric"() -> (w1200:dbl)
            n688 = call "Mobility-Vt Calculator-File.vi"("NumPts"=w1219, "Path"=w1156) -> ("Graph Cluster"=w1189:T11, "Output"=w1218:T12, 4:w1217, 5:w1204)  [unwired: 4 in, 2 out]
            n689 = call "STS Calculator-File.vi"("NumPts"=w1216, "Path"=w1156) -> ("Used Points"=w1215:T10, "XY Graph-Sat"=w1214:cluster{dbl[], dbl[]}[], "Ouput"=w1213:cluster{"STS-Sat":dbl, "STS-Lin":dbl})  [unwired: 6 in, 1 out]
            n690 = call-poly <vilib>:"Read From Spreadsheet File.vi"("file path (dialog if empty)"=w1156) -> ("all rows"=w1294:string[][])  [unwired: 6 in, 4 out]
            n691 = Unbundle By Name(w1218) -> ("Mobility-Sat"=w1203:dbl, "Vt-Sat"=w1196:dbl, "Mobility-Lin"=w1202:dbl, "Vt-Lin"=w1201:dbl, "Off I-Sat"=w1195:dbl, "On/Off I-Sat"=w1190:dbl)
            n692 = local write "Sat-Trans Slider"(w1217) -> ()
            n693 = Unbundle By Name(w1213) -> ("STS-Sat"=w1197:dbl)  [unwired: 1 out]
            n694 = local write "Index 2"(w1215) -> ()
            n695 = local write "MobVi Index"(w1217) -> ()
            n696 = local write "Sat-Log"(w1214) -> ()
            n697 = local write "Calc: Mobility-Sat"(w1203) -> ()
            n698 = local write "Calc: VT-Sat"(w1196) -> ()
            n699 = local write "Calc: Mobility-Lin"(w1202) -> ()
            n700 = local write "Calc: Off I-Sat"(w1195) -> ()
            n701 = local write "Calc: On/Off"(w1190) -> ()
            n702 = Array Size(array=w1294) -> (size(s)=w1293:i32[])
            n703 = local write "Calc: VT-Lin"(w1201) -> ()
            n704 = call "Trap Density_VT.vi"("VT"=w1196, "Dielectric"=w1200) -> ("Trap Density-VT"=w1199:dbl)
            n705 = call "Trap Density_STS.vi"("Temp (T) [K]"=w1193, "S.T.S. (S)"=w1197, "Dielectric"=w1200) -> ("Trap Density (N)"=w1198:dbl)  [unwired: 8 in]
            n706 = Unbundle By Name(w1189) -> ("Raw Sat"=w1186:cluster{dbl[], dbl[]}[], "Sqrt Sat"=w1187:cluster{dbl[], dbl[]}[], "Raw Lin"=w1185:cluster{dbl[], dbl[]}[], "Sqrt Lin"=w1188:cluster{dbl[], dbl[]}[], "Log Lin"=w1184:cluster{dbl[], dbl[]}[])  [unwired: 1 out]
            n707 = local write "Sqrt-Sat"(w1187) -> ()
            n708 = local write "Calc: STS"(w1197) -> ()
            n709 = local write "New: STS"(w1197) -> ()
            n710 = Decimate 1D Array(w1188) -> (w1212:cluster{dbl[], dbl[]}[])  [unwired: 1 out]
            n711 = local write "Calc: Trap Density-VT"(w1199) -> ()
            n712 = local write "New: VT-Sat"(w1196) -> ()
            n713 = local write "Calc: Trap Density-STS"(w1198) -> ()
            n714 = local write "New: Trap Density-STS"(w1198) -> ()
            n715 = local write "New: Trap Density-VT"(w1199) -> ()
            n716 = local write "New: VT-Lin"(w1201) -> ()
            n717 = local write "Sqrt-Lin"(w1188) -> ()
            n718 = local write "New: Mobility-Sat"(w1203) -> ()
            n719 = local write "New: Mobility-Lin"(w1202) -> ()
            n720 = Decimate 1D Array(w1214) -> (w1273:cluster{dbl[], dbl[]}[])  [unwired: 1 out]
            n721 = Index Array(array=w1293, index=w1292) -> (element=w1279:i32)
            n722 = Decimate 1D Array(w1187) -> (w1283:cluster{dbl[], dbl[]}[])  [unwired: 1 out]
            n723 = Array To Cluster(array=w1212) -> (cluster=w1211:T13)
            n724 = Array Subset(array=w1294, index (row)=w1292, index (col)=w1292, length (col)=3) -> (w1295:string[][])  [unwired: 1 in]
            n725 = local write "Raw- Sat"(w1186) -> ()
            n726 = local write "Raw- Lin"(w1185) -> ()
            n727 = local write "Log-Lin"(w1184) -> ()
            n728 = Array To Cluster(array=w1273) -> (cluster=w1271:T13)
            n729 = Array To Cluster(array=w1283) -> (cluster=w1285:T13)
            n730 = Reshape Array(w1295, w1279) -> (w1286:string[])
            n731 = Subtract(x=w1279, y=20) -> (x-y=w1278:i32)
            n732 = Unbundle(w1211) -> ("[0]"=w1208:cluster{dbl[], dbl[]})  [unwired: 8 out]
            n733 = property on="Sat-Trans Slider" class="Slide (strict)"("Scale.Maximum"=w1278) -> ()  [unwired: 2 in, 2 out]
            n734 = local read "Num Pts"() -> (w1205:dbl)
            n735 = Unbundle(w1271) -> ("[0]"=w1272:cluster{dbl[], dbl[]})  [unwired: 8 out]
            n736 = Unbundle(w1285) -> ("[0]"=w1284:cluster{dbl[], dbl[]})  [unwired: 8 out]
            n737 = Unbundle(w1208) -> (w1207:dbl[], w1206:dbl[])
            n738 = Search 1D Array(1D array=w1286, element="Index:") -> (index of element=w1289:i32)  [unwired: 1 in]
            n739 = Increment(x=w1289) -> (x+1=w1290:i32)
            n740 = Unbundle(w1272) -> (w1270:dbl[], w1269:dbl[])
            n741 = Unbundle(w1284) -> (w1277:dbl[], w1276:dbl[])
            n742 = Array Subset(array=w1207, index=w1204, length=w1205) -> (w1209:dbl[])
            n743 = Array Subset(array=w1206, index=w1204, length=w1205) -> (w1210:dbl[])
            n744 = local read "Image Folder"() -> (w1245:path)
            n745 = local write "Lin-Vg Array-Used"(w1209) -> ()
            n746 = Array Subset(array=w1270, index=w1215, length=w1216) -> (w1275:dbl[])
            n747 = Array Subset(array=w1269, index=w1215, length=w1216) -> (w1274:dbl[])
            n748 = Array Subset(array=w1277, index=w1217, length=w1219) -> (w1282:dbl[])
            n749 = Array Subset(array=w1276, index=w1217, length=w1219) -> (w1281:dbl[])
            n750 = local write "Lin Id-Used"(w1210) -> ()
            n751 = Index Array(array=w1286, index=w1290) -> (element=w1252:string)
            n752 = local write "Sat Vg Array-Used"(w1282) -> ()
            n753 = local write "Vg Array-Log-Used"(w1274) -> ()
            n754 = local write "Sat Id-Log-Used"(w1275) -> ()
            n755 = local write "Sat Id-Used"(w1281) -> ()
            n756 = local write "Index"(w1252) -> ()
            n757 = List Folder(path=w1245, error in=w1256) -> (filenames=w1288:string[], error out=w1255:errorcluster)  [unwired: 2 in, 2 out]
            n758 = Build Path(base path=w1245, name or relative path="ROI") -> (appended path=w1253:path)
            n759 = invoke on="Image Out" class="ImageControl" method="Clear ROI"(error in=w1255) -> (error out=w1259:errorcluster)  [unwired: 2 in, 2 out]
            n760 = while {
              tunnel: w1288 -> [w1318]
              tunnel: w1252 -> [w1316]
              tunnel: [w1315] -> w1287
              tunnel: w1279 -> [w1314]
              i -> [w1315]
              stop <- w1311 stop-if-true
              n761 = Index Array(array=w1318, index=w1315) -> (element=w1319:string)
              n762 = xnode "Match Regular Expression"("input string"=w1319, "regular expression"=w1316) -> ("whole match"=w1317:string)  [unwired: 4 in, 4 out]
              n763 = Equal?(x=w1317, y=w1316) -> (x = y?=w1313:bool)
              n764 = Equal?(x=w1314, y=w1315) -> (x = y?=w1312:bool)
              n765 = Or(x=w1313, y=w1312) -> (x .or. y?=w1311:bool)
            }
            n766 = Build Path(base path=w1253, name or relative path=w1252) -> (appended path=w1251:path)
            n767 = call <vilib>:"Check if File or Folder Exists.vi"("error in (no error)"=w1259, "path"=w1251) -> ("file or folder exists?"=w1257:bool, "dup path"=w1258:path)  [unwired: 7 in, 1 out]
            n768 = case shown="True" w1257 {
              tunnel: w1258 -> [_ w1306]
              frame False {
              }
              frame True {
                n769 = Read from Text File(file (use dialog)=w1306) -> (text=w1310:string)  [unwired: 3 in, 3 out]
                n770 = property on="Image Out" class="ImageControl"() -> ("ROI"=w1307:T15)  [unwired: 2 in, 2 out]
                n771 = Unflatten From String(type=w1307, binary string=w1310) -> (value=w1308:T15, error out=w1309:errorcluster)  [unwired: 3 in, 1 out]
                n772 = property on="Image Out" class="ImageControl"(error in=w1309, "ROI"=w1308) -> ()  [unwired: 1 in, 2 out]
              }
            }
            n773 = call-poly <vilib>:"Read From Spreadsheet File.vi"("file path (dialog if empty)"=w1156) -> ("all rows"=w1160:string[][])  [unwired: 6 in, 4 out]
            n774 = Array Size(array=w1160) -> (size(s)=w1179:i32[])
            n775 = Index Array(array=w1179, index=0) -> (element=w1177:i32)
            n776 = Index Array(array=w1288, index=w1287) -> (element=w1261:string)
            n777 = local write "Image Name"(w1261) -> ()
            n778 = Array Subset(array=w1160, index (row)=w1178, index (col)=w1178, length (col)=3) -> (w1180:string[][])  [unwired: 1 in]
            n779 = Empty String/Path?(string/path=w1261) -> (empty?=w1268:bool)
            n780 = Build Path(base path=w1245, name or relative path=w1261) -> (appended path=w1260:path)
            n781 = local read "No Image File"() -> (w1267:path)
            n782 = Reshape Array(w1180, w1177) -> (w1162:string[])
            n783 = Search 1D Array(1D array=w1162, element="Vg") -> (index of element=w1166:i32)  [unwired: 1 in]
            n784 = Add(x=w1166, y=3) -> (x+y=w1164:i32)
            n785 = Divide(x=w1164, y=3) -> (x/y=w1171:dbl)
            n786 = Array Subset(array=w1160, index (row)=w1171, index (col)=0, length (col)=1) -> (w1170:string[][])  [unwired: 1 in]
            n787 = Fract/Exp String To Number(string=w1170) -> (number=w1174:dbl[][])  [unwired: 3 in, 1 out]
            n788 = Array Size(array=w1174) -> (size(s)=w1161:i32[])
            n789 = Index Array(array=w1161, index=0) -> (element=w1172:i32)
            n790 = Decrement(x=w1172) -> (x-1=w1175:i32)
            n791 = Reshape Array(w1174, w1175) -> (w1159:dbl[])
            n792 = local write "Data Length"(w1175) -> ()
            n793 = local write "Vg Column"(w1159) -> ()
            n794 = Array Max & Min(array=w1159) -> (max value=w1158:dbl, min value=w1157:dbl)  [unwired: 2 out]
            n795 = Select(t=w1267, s=w1268, f=w1260) -> (s? t:f=w1262:path)
            n796 = call <vilib>:"Get File Extension.vi"("file"=w1262) -> ("lowercase file extension"=w1264:string)  [unwired: 7 in, 3 out]
            n797 = local write "Image File"(w1262) -> ()
            n798 = local write "String"(w1264) -> ()
            n799 = property on="Sat-Trans Slider" class="Slide (strict)"("Scale.Maximum"=w1158, "Scale.Minimum"=w1157) -> ()  [unwired: 2 in, 2 out]
            n800 = Search 1D Array(1D array=string[] ["bmp", "jpeg", "png", "jpg", "gif"], element=w1264) -> (index of element=w1263:i32)  [unwired: 1 in]
            n801 = call "Vision Acquisition5"("Image Path"=w1262) -> ("Image Out"=w1266:T2)  [unwired: 25 in, 1 out]
            n802 = Less Than 0?(x=w1263) -> ()  [unwired: 1 out]
            n803 = local write "Image Out"(w1266) -> ()
            n804 = local write "Image Out 2"(w1266) -> ()
          }
          event "Save Changes? 3": Mouse Down {
            n805 = event-data() -> ()  [unwired: 1 in, 7 out]
            n806 = local read "Image Folder"() -> (w1435:path)
            n807 = Build Path(base path=w1435, name or relative path="ROI") -> (appended path=w1442:path)
            n808 = call <vilib>:"Check if File or Folder Exists.vi"("path"=w1442) -> ("file or folder exists?"=w1444:bool, "dup path"=w1441:path)  [unwired: 8 in, 1 out]
            n809 = case shown="False" w1444 {
              tunnel: w1441 -> [w1446 w1447]
              tunnel: [w1445 w1447] -> w1436
              frame False {
                n810 = Create Folder(path (use dialog)=w1446) -> (created path=w1445:path)  [unwired: 2 in, 2 out]
              }
              frame True {
              }
            }
            n811 = local read "Index"() -> (w1438:string)
            n812 = property on="Image Out" class="ImageControl"() -> ("ROI"=w1440:T15)  [unwired: 2 in, 2 out]
            n813 = Build Path(base path=w1436, name or relative path=w1438) -> (appended path=w1437:path)
            n814 = Flatten To String(anything=w1440) -> (data string=w1439:string)  [unwired: 3 in, 2 out]
            n815 = Write to Text File(file (use dialog)=w1437, text=w1439) -> ()  [unwired: 2 in, 3 out]
          }
          event "Next Sqrt Sat": Mouse Down {
            n816 = event-data() -> ()  [unwired: 1 in, 5 out]
            n817 = local read "Sqrt-Sat"() -> (w1460:cluster{dbl[], dbl[]}[])
            n818 = Decimate 1D Array(w1460) -> (w1456:cluster{dbl[], dbl[]}[], w1455:cluster{dbl[], dbl[]}[])
            n819 = Array To Cluster(array=w1456) -> (cluster=w1466:T13)
            n820 = Unbundle(w1466) -> ("[0]"=w1465:cluster{dbl[], dbl[]})  [unwired: 8 out]
            n821 = local read "MobVi Index"() -> (w1462:dbl)
            n822 = local read "Num Pts"() -> (w1461:dbl)
            n823 = Unbundle(w1465) -> (w1464:dbl[], w1463:dbl[])
            n824 = Increment(x=w1462) -> (x+1=w1457:dbl)
            n825 = local read "New: Dielectric"() -> (w1451:dbl)
            n826 = local read "New: Length"() -> (w1450:dbl)
            n827 = local read "New: Width"() -> (w1449:dbl)
            n828 = local write "MobVi Index"(w1457) -> ()
            n829 = Array Subset(array=w1464, index=w1457, length=w1461) -> (w1453:dbl[])
            n830 = Array Subset(array=w1463, index=w1457, length=w1461) -> (w1452:dbl[])
            n831 = local write "Sat Vg Array-Used"(w1453) -> ()
            n832 = local write "Sat Id-Used"(w1452) -> ()
            n833 = call "Mobility-Vt-Used Pts_Saturation.vi"("Width"=w1449, "Length"=w1450, "Dielectric (d)"=w1451, "Sat Id Used"=w1452, "Vg Used"=w1453) -> ("Vt"=w1448:dbl, "Mobility"=w1454:dbl)  [unwired: 4 in, 1 out]
            n834 = Bundle(w1453, w1452) -> (w1459:cluster{dbl[], dbl[]})  [unwired: 1 in]
            n835 = Build Array (concatenate)(w1456, w1455, w1459) -> (w1458:cluster{dbl[], dbl[]}[])
            n836 = local write "New: Mobility-Sat"(w1454) -> ()
            n837 = local write "New: VT-Sat"(w1448) -> ()
            n838 = local write "Sqrt-Sat"(w1458) -> ()
          }
          event "Next Log Sat": Mouse Down {
            n839 = event-data() -> ()  [unwired: 1 in, 7 out]
            n840 = local read "Sat-Log"() -> (w1475:cluster{dbl[], dbl[]}[])
            n841 = Decimate 1D Array(w1475) -> (w1471:cluster{dbl[], dbl[]}[], w1470:cluster{dbl[], dbl[]}[])
            n842 = Array To Cluster(array=w1471) -> (cluster=w1481:T13)
            n843 = local read "Index 2"() -> (w1477:dbl)
            n844 = local read "NumPoints Log"() -> (w1476:dbl)
            n845 = Unbundle(w1481) -> ("[0]"=w1480:cluster{dbl[], dbl[]})  [unwired: 8 out]
            n846 = Unbundle(w1480) -> (w1479:dbl[], w1478:dbl[])
            n847 = Increment(x=w1477) -> (x+1=w1472:dbl)
            n848 = local write "Index 2"(w1472) -> ()
            n849 = Array Subset(array=w1478, index=w1472, length=w1476) -> (w1467:dbl[])
            n850 = Array Subset(array=w1479, index=w1472, length=w1476) -> (w1468:dbl[])
            n851 = call "STS-Used.vi"("Id Used"=w1468, "Vg-Used"=w1467) -> ("STS"=w1469:dbl)  [unwired: 9 in]
            n852 = Bundle(w1468, w1467) -> (w1474:cluster{dbl[], dbl[]})  [unwired: 1 in]
            n853 = local write "Vg Array-Log-Used"(w1467) -> ()
            n854 = local write "Sat Id-Log-Used"(w1468) -> ()
            n855 = local write "New: STS"(w1469) -> ()
            n856 = Build Array (concatenate)(w1471, w1470, w1474) -> (w1473:cluster{dbl[], dbl[]}[])
            n857 = local write "Sat-Log"(w1473) -> ()
          }
          event "Previous Log Sat": Mouse Down {
            n858 = event-data() -> ()  [unwired: 1 in, 7 out]
            n859 = local read "Sat-Log"() -> (w1491:cluster{dbl[], dbl[]}[])
            n860 = Decimate 1D Array(w1491) -> (w1488:cluster{dbl[], dbl[]}[], w1487:cluster{dbl[], dbl[]}[])
            n861 = Array To Cluster(array=w1488) -> (cluster=w1496:T13)
            n862 = local read "Index 2"() -> (w1484:dbl)
            n863 = local read "NumPoints Log"() -> (w1492:dbl)
            n864 = Unbundle(w1496) -> ("[0]"=w1495:cluster{dbl[], dbl[]})  [unwired: 8 out]
            n865 = Unbundle(w1495) -> (w1494:dbl[], w1493:dbl[])
            n866 = Decrement(x=w1484) -> (x-1=w1485:dbl)
            n867 = local write "Index 2"(w1485) -> ()
            n868 = Array Subset(array=w1494, index=w1485, length=w1492) -> (w1482:dbl[])
            n869 = Array Subset(array=w1493, index=w1485, length=w1492) -> (w1483:dbl[])
            n870 = local write "Sat Id-Log-Used"(w1482) -> ()
            n871 = Bundle(w1482, w1483) -> (w1490:cluster{dbl[], dbl[]})  [unwired: 1 in]
            n872 = call "STS-Used.vi"("Id Used"=w1482, "Vg-Used"=w1483) -> ("STS"=w1486:dbl)  [unwired: 9 in]
            n873 = local write "Vg Array-Log-Used"(w1483) -> ()
            n874 = Build Array (concatenate)(w1488, w1487, w1490) -> (w1489:cluster{dbl[], dbl[]}[])
            n875 = local write "New: STS"(w1486) -> ()
            n876 = local write "Sat-Log"(w1489) -> ()
          }
          event "Previous Sqrt Sat": Mouse Down {
            n877 = event-data() -> ()  [unwired: 1 in, 5 out]
            n878 = local read "Sqrt-Sat"() -> (w1510:cluster{dbl[], dbl[]}[])
            n879 = Decimate 1D Array(w1510) -> (w1507:cluster{dbl[], dbl[]}[], w1506:cluster{dbl[], dbl[]}[])
            n880 = Array To Cluster(array=w1507) -> (cluster=w1515:T13)
            n881 = local read "MobVi Index"() -> (w1505:dbl)
            n882 = Unbundle(w1515) -> ("[0]"=w1514:cluster{dbl[], dbl[]})  [unwired: 8 out]
            n883 = local read "Num Pts"() -> (w1511:dbl)
            n884 = Unbundle(w1514) -> (w1513:dbl[], w1512:dbl[])
            n885 = Decrement(x=w1505) -> (x-1=w1504:dbl)
            n886 = local read "New: Dielectric"() -> (w1498:dbl)
            n887 = local read "New: Length"() -> (w1499:dbl)
            n888 = local read "New: Width"() -> (w1500:dbl)
            n889 = local write "MobVi Index"(w1504) -> ()
            n890 = Array Subset(array=w1513, index=w1504, length=w1511) -> (w1503:dbl[])
            n891 = Array Subset(array=w1512, index=w1504, length=w1511) -> (w1502:dbl[])
            n892 = local write "Sat Vg Array-Used"(w1503) -> ()
            n893 = local write "Sat Id-Used"(w1502) -> ()
            n894 = call "Mobility-Vt-Used Pts_Linear.vi"("Width"=w1500, "Length"=w1499, "Dielectric (d)"=w1498, "Id Used"=w1502, "Vg Used"=w1503) -> ("Vt"=w1497:dbl, "Mobility"=w1501:dbl)  [unwired: 4 in, 1 out]
            n895 = Bundle(w1503, w1502) -> (w1509:cluster{dbl[], dbl[]})  [unwired: 1 in]
            n896 = local write "New: VT-Sat"(w1497) -> ()
            n897 = Build Array (concatenate)(w1507, w1506, w1509) -> (w1508:cluster{dbl[], dbl[]}[])
            n898 = local write "New: Mobility-Sat"(w1501) -> ()
            n899 = local write "Sqrt-Sat"(w1508) -> ()
          }
          event "Sat-Trans Slider": Value Change {
            n900 = event-data() -> ()  [unwired: 1 in, 5 out]
            n901 = local read "Sqrt-Sat"() -> (w1528:cluster{dbl[], dbl[]}[])
            n902 = Decimate 1D Array(w1528) -> (w1525:cluster{dbl[], dbl[]}[], w1524:cluster{dbl[], dbl[]}[])
            n903 = Array To Cluster(array=w1525) -> (cluster=w1533:T13)
            n904 = Unbundle(w1533) -> ("[0]"=w1532:cluster{dbl[], dbl[]})  [unwired: 8 out]
            n905 = local read "Sat-Trans Slider"() -> (w1517:dbl)
            n906 = local read "Num Pts"() -> (w1529:dbl)
            n907 = Unbundle(w1532) -> (w1531:dbl[], w1530:dbl[])
            n908 = local read "New: Dielectric"() -> (w1518:dbl)
            n909 = local read "New: Length"() -> (w1519:dbl)
            n910 = local read "New: Width"() -> (w1520:dbl)
            n911 = local write "MobVi Index"(w1517) -> ()
            n912 = Array Subset(array=w1531, index=w1517, length=w1529) -> (w1523:dbl[])
            n913 = Array Subset(array=w1530, index=w1517, length=w1529) -> (w1522:dbl[])
            n914 = local write "Sat Vg Array-Used"(w1523) -> ()
            n915 = local write "Sat Id-Used"(w1522) -> ()
            n916 = call "Mobility-Vt-Used Pts_Linear.vi"("Width"=w1520, "Length"=w1519, "Dielectric (d)"=w1518, "Id Used"=w1522, "Vg Used"=w1523) -> ("Vt"=w1516:dbl, "Mobility"=w1521:dbl)  [unwired: 4 in, 1 out]
            n917 = Bundle(w1523, w1522) -> (w1527:cluster{dbl[], dbl[]})  [unwired: 1 in]
            n918 = local write "New: VT-Sat"(w1516) -> ()
            n919 = Build Array (concatenate)(w1525, w1524, w1527) -> (w1526:cluster{dbl[], dbl[]}[])
            n920 = local write "New: Mobility-Sat"(w1521) -> ()
            n921 = local write "Sqrt-Sat"(w1526) -> ()
          }
          event "Sat-Log Slider": Value Change {
            n922 = event-data() -> ()  [unwired: 1 in, 5 out]
            n923 = local read "Sat-Log"() -> (w1542:cluster{dbl[], dbl[]}[])
            n924 = Decimate 1D Array(w1542) -> (w1539:cluster{dbl[], dbl[]}[], w1538:cluster{dbl[], dbl[]}[])
            n925 = Array To Cluster(array=w1539) -> (cluster=w1547:T13)
            n926 = Unbundle(w1547) -> ("[0]"=w1546:cluster{dbl[], dbl[]})  [unwired: 8 out]
            n927 = local read "NumPoints Log"() -> (w1543:dbl)
            n928 = local read "Sat-Log Slider"() -> (w1537:dbl)
            n929 = Unbundle(w1546) -> (w1545:dbl[], w1544:dbl[])
            n930 = local write "Index 2"(w1537) -> ()
            n931 = Array Subset(array=w1545, index=w1537, length=w1543) -> (w1535:dbl[])
            n932 = Array Subset(array=w1544, index=w1537, length=w1543) -> (w1534:dbl[])
            n933 = local write "Vg Array-Log-Used"(w1534) -> ()
            n934 = local write "Sat Id-Log-Used"(w1535) -> ()
            n935 = call "STS-Used.vi"("Id Used"=w1535, "Vg-Used"=w1534) -> ("STS"=w1536:dbl)  [unwired: 9 in]
            n936 = Bundle(w1535, w1534) -> (w1541:cluster{dbl[], dbl[]})  [unwired: 1 in]
            n937 = local write "New: STS"(w1536) -> ()
            n938 = Build Array (concatenate)(w1539, w1538, w1541) -> (w1540:cluster{dbl[], dbl[]}[])
            n939 = local write "Sat-Log"(w1540) -> ()
          }
          event "Save Changes?": Mouse Down {
            n940 = event-data() -> ()  [unwired: 1 in, 5 out]
            n941 = flat-sequence {
              tunnel: [w1554] -> w1552
              tunnel: [w1562] -> w1551
              tunnel: [w1555] -> w1550
              tunnel: w1552 -> [w2094]
              tunnel: w1551 -> [w2091]
              tunnel: [w2092] -> w1549
              tunnel: w1550 -> [w2092]
              tunnel: [w2091] -> w1548
              tunnel: w1549 -> [w2099]
              tunnel: w1548 -> [w2098]
              frame #0 {
                n942 = Wait (ms)(milliseconds to wait=1) -> ()  [unwired: 1 out]
              }
              frame #1 {
                n943 = local read "Transfer File"() -> (w1554:path)
                n944 = local read "New: Temp"() -> (w1556:dbl)
                n945 = local read "New: Length"() -> (w1560:dbl)
                n946 = local read "New: Width"() -> (w1558:dbl)
                n947 = To Single Precision Float(number=w1556) -> (single precision float=w1557:sgl)
                n948 = Number To Decimal String(number=w1557) -> (decimal integer string=w1565:string)  [unwired: 1 in]
                n949 = To Single Precision Float(number=w1558) -> (single precision float=w1559:sgl)
                n950 = To Single Precision Float(number=w1560) -> (single precision float=w1561:sgl)
                n951 = local read "Index"() -> (w1570:string)
                n952 = Strip Path(path=w1554) -> (stripped path=w1575:path)  [unwired: 1 out]
                n953 = Number To Decimal String(number=w1561) -> (decimal integer string=w1568:string)  [unwired: 1 in]
                n954 = Number To Decimal String(number=w1559) -> (decimal integer string=w1569:string)  [unwired: 1 in]
                n955 = Concatenate Strings("_", w1565, "K") -> (w1563:string)
                n956 = call "Build Text"("Temp"=w1563, "Index"=w1570, "Length"=w1568, "Width"=w1569) -> ("Result"=w1571:string)  [unwired: 10 in, 1 out]
                n957 = flat-sequence {
                  tunnel: [w2048] -> w1567
                  tunnel: w1567 -> [w2065]
                  frame #0 {
                    # "Makes Empty File for Transformer Data"
                    n958 = local read "Transfer Folder"() -> (w2037:path)
                    n959 = Build Path(base path=w2037, name or relative path="Stats") -> (appended path=w2039:path)
                    n960 = call <vilib>:"Check if File or Folder Exists.vi"("path"=w2039) -> ("file or folder exists?"=w2040:bool, "dup path"=w2041:path)  [unwired: 8 in, 1 out]
                    n961 = case shown="False" w2040 {
                      tunnel: [w2045 w2047] -> w2042
                      tunnel: w2041 -> [w2046 w2047]
                      frame False {
                        n962 = Create Folder(path (use dialog)=w2046) -> (created path=w2045:path)  [unwired: 2 in, 2 out]
                      }
                      frame True {
                      }
                    }
                    n963 = Build Path(base path=w2042, name or relative path="Tranformer Data.txt") -> (appended path=w2044:path)
                    n964 = call-poly <vilib>:"Write To Spreadsheet File.vi"("append to file? (new file:F)"=TRUE, "file path (dialog if empty)"=w2044) -> ()  [unwired: 6 in, 1 out]
                  }
                  frame #1 {
                    # "Adds Headers if they don't exist"
                    n965 = local read "Transfer Folder"() -> (w2054:path)
                    n966 = Concatenate Strings("Stats\\", "Tranformer Data.txt") -> (w2055:string)
                    n967 = Build Path(base path=w2054, name or relative path=w2055) -> (appended path=w2048:path)
                    n968 = call-poly <vilib>:"Read From Spreadsheet File.vi"("file path (dialog if empty)"=w2048) -> ("first row"=w2053:string[])  [unwired: 6 in, 4 out]
                    n969 = Search 1D Array(1D array=w2053, element="DeviceID") -> (index of element=w2051:i32)  [unwired: 1 in]
                    n970 = Equal?(x=w2051, y=0) -> (x = y?=w2049:bool)
                    n971 = case shown="False" w2049 {
                      tunnel: w2048 -> [w2059 _]
                      frame False {
                        n972 = local read "Transformer \nHeaders"() -> (w2058:string[])
                        n973 = call-poly <vilib>:"Write To Spreadsheet File.vi"("1D data"=w2058, "file path (dialog if empty)"=w2059) -> ()  [unwired: 6 in, 1 out]
                      }
                      frame True {
                      }
                    }
                  }
                  frame #2 {
                    # "Adds current device if it doesn't exist"
                    n974 = local read "Current \nRecord"() -> (w2064:string[])
                    n975 = Index Array(array=w2064, index=0) -> (element=w2063:string)
                    n976 = local read "Transfer Folder"() -> (w2067:path)
                    n977 = Concatenate Strings("Stats\\", "Tranformer Data.txt") -> (w2068:string)
                    n978 = local write "Current Device ID"(w2063) -> ()
                    n979 = local read "Current Device ID"() -> (w2073:string)
                    n980 = Build Path(base path=w2067, name or relative path=w2068) -> (appended path=w2066:path)
                    n981 = call-poly <vilib>:"Read From Spreadsheet File.vi"("file path (dialog if empty)"=w2066) -> ("all rows"=w2060:string[][])  [unwired: 6 in, 4 out]
                    n982 = Index Array(array=w2060, index (col)=0) -> (element=w2061:string[])  [unwired: 1 in]
                    n983 = Search 1D Array(1D array=w2061, element=w2073) -> (index of element=w2062:i32)  [unwired: 1 in]
                    n984 = Equal?(x=w2062, y=-1) -> (x = y?=w2075:bool)
                    n985 = case shown="False" w2075 {
                      tunnel: w2065 -> [w2078 w2089]
                      tunnel: w2062 -> [w2081 _]
                      tunnel: w2060 -> [w2082 _]
                      frame False {
                        n986 = local read "Current \nRecord"() -> (w2080:string[])
                        n987 = Replace Array Subset(array=w2082, new element=w2080, index (row)=w2081) -> (w2079:string[][])  [unwired: 1 in]
                        n988 = flat-sequence {
                          tunnel: w2078 -> [w2083]
                          tunnel: w2079 -> [w2084]
                          tunnel: [w2084] -> w2077
                          tunnel: [w2083] -> w2076
                          tunnel: w2077 -> [w2086]
                          tunnel: w2076 -> [w2085]
                          frame #0 {
                            n989 = Delete(path (use dialog)=w2083) -> ()  [unwired: 4 in, 3 out]
                          }
                          frame #1 {
                            n990 = call-poly <vilib>:"Write To Spreadsheet File.vi"("append to file? (new file:F)"=TRUE, "2D data"=w2086, "file path (dialog if empty)"=w2085) -> ()  [unwired: 5 in, 1 out]
                          }
                        }
                      }
                      frame True {
                        n991 = local read "Current \nRecord"() -> (w2088:string[])
                        n992 = call-poly <vilib>:"Write To Spreadsheet File.vi"("append to file? (new file:F)"=TRUE, "1D data"=w2088, "file path (dialog if empty)"=w2089) -> ()  [unwired: 5 in, 1 out]
                      }
                    }
                  }
                }
                n993 = Path To String(path=w1575) -> (string=w1573:string)
                n994 = stacked-sequence {
                  tunnel: [_ _ _ _ _ _ _ _ _ _ _ _ _ w2008] -> w1555
                  tunnel: w1554 -> [w1577 _ _ _ _ _ _ _ _ _ _ _ _ _]
                  frame #0 {
                    n995 = call-poly <vilib>:"Read From Spreadsheet File.vi"("file path (dialog if empty)"=w1577) -> ("all rows"=w1576:string[][])  [unwired: 6 in, 4 out]
                    n996 = Array Size(array=w1576) -> (size(s)=w1581:i32[])
                    n997 = Array Subset(array=w1576, index (row)=0, index (col)=0, length (col)=3) -> (w1585:string[][])  [unwired: 1 in]
                    n998 = Index Array(array=w1581, index=0) -> (element=w1579:i32)
                    n999 = Reshape Array(w1585, w1579) -> (w1578:string[])
                    n1000 = Search 1D Array(1D array=w1578, element="Dielectric (nm):") -> (index of element=w1588:i32)  [unwired: 1 in]
                    n1001 = Equal?(x=w1588, y=-1) -> (x = y?=w1587:bool)
                    n1002 = case shown="False" w1587 {
                      tunnel: w1576 -> [w1596 w1600]
                      tunnel: w1588 -> [w1592 _]
                      tunnel: [w1591 w1600] -> w1586
                      frame False {
                        n1003 = local read "New: Dielectric"() -> (w1598:dbl)
                        n1004 = Number To Fractional String(number=w1598) -> (F-format string=w1593:string)  [unwired: 3 in]
                        n1005 = Divide(x=w1592, y=3) -> (x/y=w1595:dbl)
                        n1006 = To Word Integer(number=w1595) -> (16bit integer=w1594:i16)
                        n1007 = Replace Array Subset(array=w1596, new element=w1593, index (row)=w1594, index (col)=1) -> (w1591:string[][])
                      }
                      frame True {
                      }
                    }
                    n1008 = local write "Save1 Array"(w1586) -> ()
                  }
                  frame #1 {
                    n1009 = local read "Save1 Array"() -> (w1602:string[][])
                    n1010 = Array Size(array=w1602) -> (size(s)=w1605:i32[])
                    n1011 = Array Subset(array=w1602, index (row)=0, index (col)=0, length (col)=3) -> (w1609:string[][])  [unwired: 1 in]
                    n1012 = Index Array(array=w1605, index=0) -> (element=w1603:i32)
                    n1013 = Reshape Array(w1609, w1603) -> (w1601:string[])
                    n1014 = Search 1D Array(1D array=w1601, element="Comments:") -> (index of element=w1612:i32)  [unwired: 1 in]
                    n1015 = Equal?(x=w1612, y=-1) -> (x = y?=w1611:bool)
                    n1016 = case shown="False" w1611 {
                      tunnel: w1602 -> [w1620 w1623]
                      tunnel: w1612 -> [w1617 _]
                      tunnel: [w1616 w1623] -> w1610
                      frame False {
                        n1017 = local read "Comments:"() -> (w1615:string)
                        n1018 = Divide(x=w1617, y=3) -> (x/y=w1619:dbl)
                        n1019 = To Word Integer(number=w1619) -> (16bit integer=w1618:i16)
                        n1020 = Replace Array Subset(array=w1620, new element=w1615, index (row)=w1618, index (col)=1) -> (w1616:string[][])
                      }
                      frame True {
                      }
                    }
                    n1021 = local write "Save1 Array"(w1610) -> ()
                  }
                  frame #2 {
                    n1022 = local read "Save1 Array"() -> (w1625:string[][])
                    n1023 = Array Size(array=w1625) -> (size(s)=w1628:i32[])
                    n1024 = Array Subset(array=w1625, index (row)=0, index (col)=0, length (col)=3) -> (w1632:string[][])  [unwired: 1 in]
                    n1025 = Index Array(array=w1628, index=0) -> (element=w1626:i32)
                    n1026 = Reshape Array(w1632, w1626) -> (w1624:string[])
                    n1027 = Search 1D Array(1D array=w1624, element="Length (um):") -> (index of element=w1635:i32)  [unwired: 1 in]
                    n1028 = Equal?(x=w1635, y=-1) -> (x = y?=w1634:bool)
                    n1029 = case shown="False" w1634 {
                      tunnel: w1625 -> [w1645 w1648]
                      tunnel: w1635 -> [w1642 _]
                      tunnel: [w1641 w1648] -> w1633
                      frame False {
                        n1030 = local read "New: Length"() -> (w1638:dbl)
                        n1031 = Divide(x=w1642, y=3) -> (x/y=w1644:dbl)
                        n1032 = Format Value(format string="%#g", value (0)=w1638) -> (output string=w1639:string)  [unwired: 1 in]
                        n1033 = To Word Integer(number=w1644) -> (16bit integer=w1643:i16)
                        n1034 = Replace Array Subset(array=w1645, new element=w1639, index (row)=w1643, index (col)=1) -> (w1641:string[][])
                      }
                      frame True {
                      }
                    }
                    n1035 = local write "Save1 Array"(w1633) -> ()
                  }
                  frame #3 {
                    n1036 = local read "Save1 Array"() -> (w1650:string[][])
                    n1037 = Array Size(array=w1650) -> (size(s)=w1655:i32[])
                    n1038 = Array Subset(array=w1650, index (row)=0, index (col)=0, length (col)=3) -> (w1651:string[][])  [unwired: 1 in]
                    n1039 = Index Array(array=w1655, index=0) -> (element=w1657:i32)
                    n1040 = Reshape Array(w1651, w1657) -> (w1649:string[])
                    n1041 = Search 1D Array(1D array=w1649, element="Width (um):") -> (index of element=w1660:i32)  [unwired: 1 in]
                    n1042 = Equal?(x=w1660, y=-1) -> (x = y?=w1659:bool)
                    n1043 = case shown="False" w1659 {
                      tunnel: w1660 -> [w1668 _]
                      tunnel: w1650 -> [w1667 w1673]
                      tunnel: [w1666 w1673] -> w1658
                      frame False {
                        n1044 = local read "New: Width"() -> (w1663:dbl)
                        n1045 = Divide(x=w1668, y=3) -> (x/y=w1670:dbl)
                        n1046 = To Word Integer(number=w1670) -> (16bit integer=w1669:i16)
                        n1047 = Format Value(format string="%#g", value (0)=w1663) -> (output string=w1664:string)  [unwired: 1 in]
                        n1048 = Replace Array Subset(array=w1667, new element=w1664, index (row)=w1669, index (col)=1) -> (w1666:string[][])
                      }
                      frame True {
                      }
                    }
                    n1049 = local write "Save1 Array"(w1658) -> ()
                  }
                  frame #4 {
                    w1683 = "Sample Temp (K):"
                    n1050 = local read "Save1 Array"() -> (w1675:string[][])
                    n1051 = Array Size(array=w1675) -> (size(s)=w1680:i32[])
                    n1052 = Array Subset(array=w1675, index (row)=0, index (col)=0, length (col)=3) -> (w1676:string[][])  [unwired: 1 in]
                    n1053 = Index Array(array=w1680, index=0) -> (element=w1682:i32)
                    n1054 = Reshape Array(w1676, w1682) -> (w1674:string[])
                    n1055 = Search 1D Array(1D array=w1674, element=w1683) -> (index of element=w1686:i32)  [unwired: 1 in]
                    n1056 = Equal?(x=w1686, y=-1) -> (x = y?=w1685:bool)
                    n1057 = case shown="True" w1685 {
                      tunnel: w1675 -> [w1695 w1709]
                      tunnel: w1686 -> [w1692 _]
                      tunnel: [w1691 w1708] -> w1684
                      tunnel: w1674 -> [_ w1711]
                      tunnel: w1683 -> [_ w1698]
                      frame False {
                        n1058 = local read "New: Temp"() -> (w1689:dbl)
                        n1059 = Divide(x=w1692, y=3) -> (x/y=w1694:dbl)
                        n1060 = Format Value(format string="%#g", value (0)=w1689) -> (output string=w1688:string)  [unwired: 1 in]
                        n1061 = To Word Integer(number=w1694) -> (16bit integer=w1693:i16)
                        n1062 = Replace Array Subset(array=w1695, new element=w1688, index (row)=w1693, index (col)=1) -> (w1691:string[][])
                      }
                      frame True {
                        n1063 = local read "New: Temp"() -> (w1700:dbl)
                        n1064 = Search 1D Array(1D array=w1711, element="Width (um):") -> (index of element=w1705:i32)  [unwired: 1 in]
                        n1065 = Divide(x=w1705, y=3) -> (x/y=w1706:dbl)
                        n1066 = To Word Integer(number=w1706) -> (16bit integer=w1704:i16)
                        n1067 = Format Value(format string="%#g", value (0)=w1700) -> (output string=w1699:string)  [unwired: 1 in]
                        n1068 = Build Array(w1698, w1699) -> (w1702:string[])
                        n1069 = Increment(x=w1704) -> (x+1=w1703:i16)
                        n1070 = Insert Into Array(array=w1709, index (row)=w1703, new element=w1702) -> (w1708:string[][])  [unwired: 1 in]
                      }
                    }
                    n1071 = local write "Save1 Array"(w1684) -> ()
                  }
                  frame #5 {
                    w1721 = "Mobility-Sat (cm^2/Vs):"
                    n1072 = local read "Save1 Array"() -> (w1713:string[][])
                    n1073 = Array Size(array=w1713) -> (size(s)=w1718:i32[])
                    n1074 = Array Subset(array=w1713, index (row)=0, index (col)=0, length (col)=3) -> (w1714:string[][])  [unwired: 1 in]
                    n1075 = Index Array(array=w1718, index=0) -> (element=w1720:i32)
                    n1076 = Reshape Array(w1714, w1720) -> (w1712:string[])
                    n1077 = Search 1D Array(1D array=w1712, element=w1721) -> (index of element=w1724:i32)  [unwired: 1 in]
                    n1078 = Equal?(x=w1724, y=-1) -> (x = y?=w1723:bool)
                    n1079 = case shown="True" w1723 {
                      tunnel: w1713 -> [w1733 w1741]
                      tunnel: w1724 -> [w1730 _]
                      tunnel: [w1729 w1740] -> w1722
                      tunnel: w1712 -> [_ w1738]
                      tunnel: w1721 -> [_ w1736]
                      frame False {
                        n1080 = local read "New: Mobility-Sat"() -> (w1726:dbl)
                        n1081 = Divide(x=w1730, y=3) -> (x/y=w1732:dbl)
                        n1082 = To Word Integer(number=w1732) -> (16bit integer=w1731:i16)
                        n1083 = Format Value(format string="%#g", value (0)=w1726) -> (output string=w1727:string)  [unwired: 1 in]
                        n1084 = Replace Array Subset(array=w1733, new element=w1727, index (row)=w1731, index (col)=1) -> (w1729:string[][])
                      }
                      frame True {
                        n1085 = local read "New: Mobility-Sat"() -> (w1742:dbl)
                        n1086 = Search 1D Array(1D array=w1738, element="Mobility (cm^2/Vs):") -> (index of element=w1745:i32)  [unwired: 1 in]
                        n1087 = Divide(x=w1745, y=3) -> (x/y=w1746:dbl)
                        n1088 = To Word Integer(number=w1746) -> (16bit integer=w1737:i16)
                        n1089 = Format Value(format string="%#g", value (0)=w1742) -> (output string=w1739:string)  [unwired: 1 in]
                        n1090 = Build Array(w1736, w1739) -> (w1744:string[])
                        n1091 = Replace Array Subset(array=w1741, new element=w1744, index (row)=w1737) -> (w1740:string[][])  [unwired: 1 in]
                      }
                    }
                    n1092 = local write "Save1 Array"(w1722) -> ()
                  }
                  frame #6 {
                    w1758 = "Mobility-Lin (cm^2/Vs):"
                    n1093 = local read "Save1 Array"() -> (w1749:string[][])
                    n1094 = Array Size(array=w1749) -> (size(s)=w1755:i32[])
                    n1095 = Array Subset(array=w1749, index (row)=0, index (col)=0, length (col)=3) -> (w1751:string[][])  [unwired: 1 in]
                    n1096 = Index Array(array=w1755, index=0) -> (element=w1757:i32)
                    n1097 = Reshape Array(w1751, w1757) -> (w1750:string[])
                    n1098 = Search 1D Array(1D array=w1750, element=w1758) -> (index of element=w1761:i32)  [unwired: 1 in]
                    n1099 = Equal?(x=w1761, y=-1) -> (x = y?=w1760:bool)
                    n1100 = case shown="True" w1760 {
                      tunnel: w1749 -> [w1770 w1776]
                      tunnel: w1761 -> [w1767 _]
                      tunnel: [w1766 w1775] -> w1759
                      tunnel: w1750 -> [_ w1774]
                      tunnel: w1758 -> [_ w1773]
                      frame False {
                        n1101 = local read "Calc: Mobility-Lin"() -> (w1763:dbl)
                        n1102 = Divide(x=w1767, y=3) -> (x/y=w1769:dbl)
                        n1103 = To Word Integer(number=w1769) -> (16bit integer=w1768:i16)
                        n1104 = Format Value(format string="%#g", value (0)=w1763) -> (output string=w1764:string)  [unwired: 1 in]
                        n1105 = Replace Array Subset(array=w1770, new element=w1764, index (row)=w1768, index (col)=1) -> (w1766:string[][])
                      }
                      frame True {
                        n1106 = local read "Calc: Mobility-Lin"() -> (w1777:dbl)
                        n1107 = Search 1D Array(1D array=w1774, element="Mobility-Sat (cm^2/Vs):") -> (index of element=w1782:i32)  [unwired: 1 in]
                        n1108 = Divide(x=w1782, y=3) -> (x/y=w1783:dbl)
                        n1109 = To Word Integer(number=w1783) -> (16bit integer=w1781:i16)
                        n1110 = Format Value(format string="%#g", value (0)=w1777) -> (output string=w1786:string)  [unwired: 1 in]
                        n1111 = Build Array(w1773, w1786) -> (w1779:string[])
                        n1112 = Increment(x=w1781) -> (x+1=w1780:i16)
                        n1113 = Insert Into Array(array=w1776, index (row)=w1780, new element=w1779) -> (w1775:string[][])  [unwired: 1 in]
                      }
                    }
                    n1114 = local write "Save1 Array"(w1759) -> ()
                  }
                  frame #7 {
                    w1796 = "On/Off I-Sat:"
                    n1115 = local read "Save1 Array"() -> (w1787:string[][])
                    n1116 = Array Size(array=w1787) -> (size(s)=w1793:i32[])
                    n1117 = Array Subset(array=w1787, index (row)=0, index (col)=0, length (col)=3) -> (w1789:string[][])  [unwired: 1 in]
                    n1118 = Index Array(array=w1793, index=0) -> (element=w1795:i32)
                    n1119 = Reshape Array(w1789, w1795) -> (w1788:string[])
                    n1120 = Search 1D Array(1D array=w1788, element=w1796) -> (index of element=w1799:i32)  [unwired: 1 in]
                    n1121 = Equal?(x=w1799, y=-1) -> (x = y?=w1798:bool)
                    n1122 = case shown="True" w1798 {
                      tunnel: w1787 -> [w1808 w1815]
                      tunnel: w1799 -> [w1805 _]
                      tunnel: [w1804 w1816] -> w1797
                      tunnel: w1788 -> [_ w1813]
                      tunnel: w1796 -> [_ w1811]
                      frame False {
                        n1123 = local read "Calc: On/Off"() -> (w1801:dbl)
                        n1124 = Divide(x=w1805, y=3) -> (x/y=w1807:dbl)
                        n1125 = To Word Integer(number=w1807) -> (16bit integer=w1806:i16)
                        n1126 = Format Value(format string="%#g", value (0)=w1801) -> (output string=w1802:string)  [unwired: 1 in]
                        n1127 = Replace Array Subset(array=w1808, new element=w1802, index (row)=w1806, index (col)=1) -> (w1804:string[][])
                      }
                      frame True {
                        n1128 = local read "Calc: On/Off"() -> (w1817:dbl)
                        n1129 = Search 1D Array(1D array=w1813, element="On/Off Current:") -> (index of element=w1820:i32)  [unwired: 1 in]
                        n1130 = Divide(x=w1820, y=3) -> (x/y=w1821:dbl)
                        n1131 = To Word Integer(number=w1821) -> (16bit integer=w1812:i16)
                        n1132 = Format Value(format string="%#g", value (0)=w1817) -> (output string=w1814:string)  [unwired: 1 in]
                        n1133 = Build Array(w1811, w1814) -> (w1819:string[])
                        n1134 = Replace Array Subset(array=w1815, new element=w1819, index (row)=w1812) -> (w1816:string[][])  [unwired: 1 in]
                      }
                    }
                    n1135 = local write "Save1 Array"(w1797) -> ()
                  }
                  frame #8 {
                    w1833 = "Off I-Sat (A):"
                    n1136 = local read "Save1 Array"() -> (w1824:string[][])
                    n1137 = Array Size(array=w1824) -> (size(s)=w1830:i32[])
                    n1138 = Array Subset(array=w1824, index (row)=0, index (col)=0, length (col)=3) -> (w1826:string[][])  [unwired: 1 in]
                    n1139 = Index Array(array=w1830, index=0) -> (element=w1832:i32)
                    n1140 = Reshape Array(w1826, w1832) -> (w1825:string[])
                    n1141 = Search 1D Array(1D array=w1825, element=w1833) -> (index of element=w1836:i32)  [unwired: 1 in]
                    n1142 = Equal?(x=w1836, y=-1) -> (x = y?=w1835:bool)
                    n1143 = case shown="True" w1835 {
                      tunnel: w1824 -> [w1845 w1851]
                      tunnel: w1836 -> [w1842 _]
                      tunnel: [w1841 w1850] -> w1834
                      tunnel: w1825 -> [_ w1849]
                      tunnel: w1833 -> [_ w1848]
                      frame False {
                        n1144 = local read "Calc: Off I-Sat"() -> (w1840:dbl)
                        n1145 = Divide(x=w1842, y=3) -> (x/y=w1844:dbl)
                        n1146 = Format Value(format string="%#g", value (0)=w1840) -> (output string=w1838:string)  [unwired: 1 in]
                        n1147 = To Word Integer(number=w1844) -> (16bit integer=w1843:i16)
                        n1148 = Replace Array Subset(array=w1845, new element=w1838, index (row)=w1843, index (col)=1) -> (w1841:string[][])
                      }
                      frame True {
                        n1149 = local read "Calc: Off I-Sat"() -> (w1852:dbl)
                        n1150 = Search 1D Array(1D array=w1849, element="On/Off I-Sat:") -> (index of element=w1857:i32)  [unwired: 1 in]
                        n1151 = Divide(x=w1857, y=3) -> (x/y=w1858:dbl)
                        n1152 = To Word Integer(number=w1858) -> (16bit integer=w1856:i16)
                        n1153 = Format Value(format string="%#g", value (0)=w1852) -> (output string=w1861:string)  [unwired: 1 in]
                        n1154 = Build Array(w1848, w1861) -> (w1854:string[])
                        n1155 = Increment(x=w1856) -> (x+1=w1855:i16)
                        n1156 = Insert Into Array(array=w1851, index (row)=w1855, new element=w1854) -> (w1850:string[][])  [unwired: 1 in]
                      }
                    }
                    n1157 = local write "Save1 Array"(w1834) -> ()
                  }
                  frame #9 {
                    w1863 = "Vt-Sat (V):"
                    n1158 = local read "Save1 Array"() -> (w1864:string[][])
                    n1159 = Array Size(array=w1864) -> (size(s)=w1869:i32[])
                    n1160 = Array Subset(array=w1864, index (row)=0, index (col)=0, length (col)=3) -> (w1865:string[][])  [unwired: 1 in]
                    n1161 = Index Array(array=w1869, index=0) -> (element=w1871:i32)
                    n1162 = Reshape Array(w1865, w1871) -> (w1862:string[])
                    n1163 = Search 1D Array(1D array=w1862, element=w1863) -> (index of element=w1874:i32)  [unwired: 1 in]
                    n1164 = Equal?(x=w1874, y=-1) -> (x = y?=w1873:bool)
                    n1165 = case shown="True" w1873 {
                      tunnel: w1864 -> [w1881 w1890]
                      tunnel: w1874 -> [w1877 _]
                      tunnel: [w1876 w1889] -> w1872
                      tunnel: w1863 -> [_ w1888]
                      tunnel: w1862 -> [_ w1887]
                      frame False {
                        n1166 = local read "New: VT-Sat"() -> (w1883:dbl)
                        n1167 = Number To Fractional String(number=w1883) -> (F-format string=w1878:string)  [unwired: 3 in]
                        n1168 = Divide(x=w1877, y=3) -> (x/y=w1880:dbl)
                        n1169 = To Word Integer(number=w1880) -> (16bit integer=w1879:i16)
                        n1170 = Replace Array Subset(array=w1881, new element=w1878, index (row)=w1879, index (col)=1) -> (w1876:string[][])
                      }
                      frame True {
                        n1171 = local read "New: VT-Sat"() -> (w1891:dbl)
                        n1172 = Search 1D Array(1D array=w1887, element="Threshold V (V):") -> (index of element=w1886:i32)  [unwired: 1 in]
                        n1173 = Divide(x=w1886, y=3) -> (x/y=w1894:dbl)
                        n1174 = To Word Integer(number=w1894) -> (16bit integer=w1885:i16)
                        n1175 = Format Value(format string="%#g", value (0)=w1891) -> (output string=w1897:string)  [unwired: 1 in]
                        n1176 = Build Array(w1888, w1897) -> (w1893:string[])
                        n1177 = Replace Array Subset(array=w1890, new element=w1893, index (row)=w1885) -> (w1889:string[][])  [unwired: 1 in]
                      }
                    }
                    n1178 = local write "Save1 Array"(w1872) -> ()
                  }
                  frame #10 {
                    n1179 = local read "Save1 Array"() -> (w1898:string[][])
                    n1180 = Array Size(array=w1898) -> (size(s)=w1904:i32[])
                    n1181 = Array Subset(array=w1898, index (row)=0, index (col)=0, length (col)=3) -> (w1900:string[][])  [unwired: 1 in]
                    n1182 = Index Array(array=w1904, index=0) -> (element=w1906:i32)
                    n1183 = Reshape Array(w1900, w1906) -> (w1899:string[])
                    n1184 = Search 1D Array(1D array=w1899, element="VT-Lin (V):") -> (index of element=w1909:i32)  [unwired: 1 in]
                    n1185 = Equal?(x=w1909, y=-1) -> (x = y?=w1908:bool)
                    n1186 = case shown="False" w1908 {
                      tunnel: w1898 -> [w1919 w1922]
                      tunnel: w1909 -> [w1916 _]
                      tunnel: [w1915 w1922] -> w1907
                      frame False {
                        n1187 = local read "New: VT-Lin"() -> (w1913:dbl)
                        n1188 = Divide(x=w1916, y=3) -> (x/y=w1918:dbl)
                        n1189 = Format Value(format string="%#g", value (0)=w1913) -> (output string=w1912:string)  [unwired: 1 in]
                        n1190 = To Word Integer(number=w1918) -> (16bit integer=w1917:i16)
                        n1191 = Replace Array Subset(array=w1919, new element=w1912, index (row)=w1917, index (col)=1) -> (w1915:string[][])
                      }
                      frame True {
                      }
                    }
                    n1192 = local write "Save1 Array"(w1907) -> ()
                  }
                  frame #11 {
                    w1923 = "STS-Sat (V/decade):"
                    n1193 = local read "Save1 Array"() -> (w1925:string[][])
                    n1194 = Array Size(array=w1925) -> (size(s)=w1930:i32[])
                    n1195 = Array Subset(array=w1925, index (row)=0, index (col)=0, length (col)=3) -> (w1926:string[][])  [unwired: 1 in]
                    n1196 = Index Array(array=w1930, index=0) -> (element=w1932:i32)
                    n1197 = Reshape Array(w1926, w1932) -> (w1924:string[])
                    n1198 = Search 1D Array(1D array=w1924, element=w1923) -> (index of element=w1935:i32)  [unwired: 1 in]
                    n1199 = Equal?(x=w1935, y=-1) -> (x = y?=w1934:bool)
                    n1200 = case shown="True" w1934 {
                      tunnel: w1925 -> [w1944 w1950]
                      tunnel: w1935 -> [w1941 _]
                      tunnel: [w1940 w1951] -> w1933
                      tunnel: w1924 -> [_ w1949]
                      tunnel: w1923 -> [_ w1948]
                      frame False {
                        n1201 = local read "New: STS"() -> (w1938:dbl)
                        n1202 = Divide(x=w1941, y=3) -> (x/y=w1943:dbl)
                        n1203 = Format Value(format string="%#g", value (0)=w1938) -> (output string=w1937:string)  [unwired: 1 in]
                        n1204 = To Word Integer(number=w1943) -> (16bit integer=w1942:i16)
                        n1205 = Replace Array Subset(array=w1944, new element=w1937, index (row)=w1942, index (col)=1) -> (w1940:string[][])
                      }
                      frame True {
                        n1206 = local read "New: STS"() -> (w1952:dbl)
                        n1207 = Search 1D Array(1D array=w1949, element="S.T.S. (V/decade):") -> (index of element=w1955:i32)  [unwired: 1 in]
                        n1208 = Divide(x=w1955, y=3) -> (x/y=w1956:dbl)
                        n1209 = To Word Integer(number=w1956) -> (16bit integer=w1947:i16)
                        n1210 = Format Value(format string="%#g", value (0)=w1952) -> (output string=w1959:string)  [unwired: 1 in]
                        n1211 = Build Array(w1948, w1959) -> (w1954:string[])
                        n1212 = Replace Array Subset(array=w1950, new element=w1954, index (row)=w1947) -> (w1951:string[][])  [unwired: 1 in]
                      }
                    }
                    n1213 = local write "Save1 Array"(w1933) -> ()
                  }
                  frame #12 {
                    w1960 = "Trap Density-VT (Traps/Vcm^2):"
                    n1214 = local read "Save1 Array"() -> (w1962:string[][])
                    n1215 = Array Size(array=w1962) -> (size(s)=w1967:i32[])
                    n1216 = Array Subset(array=w1962, index (row)=0, index (col)=0, length (col)=3) -> (w1963:string[][])  [unwired: 1 in]
                    n1217 = Index Array(array=w1967, index=0) -> (element=w1969:i32)
                    n1218 = Reshape Array(w1963, w1969) -> (w1961:string[])
                    n1219 = Search 1D Array(1D array=w1961, element=w1960) -> (index of element=w1972:i32)  [unwired: 1 in]
                    n1220 = Equal?(x=w1972, y=-1) -> (x = y?=w1971:bool)
                    n1221 = case shown="True" w1971 {
                      tunnel: w1962 -> [w1981 w1986]
                      tunnel: w1972 -> [w1977 _]
                      tunnel: [w1976 w1987] -> w1970
                      tunnel: w1961 -> [_ w1985]
                      tunnel: w1960 -> [_ w1984]
                      frame False {
                        n1222 = local read "New: Trap Density-VT"() -> (w1975:dbl)
                        n1223 = Format Value(format string="%#g", value (0)=w1975) -> (output string=w1978:string)  [unwired: 1 in]
                        n1224 = Divide(x=w1977, y=3) -> (x/y=w1980:dbl)
                        n1225 = To Word Integer(number=w1980) -> (16bit integer=w1979:i16)
                        n1226 = Replace Array Subset(array=w1981, new element=w1978, index (row)=w1979, index (col)=1) -> (w1976:string[][])
                      }
                      frame True {
                        n1227 = local read "New: Trap Density-VT"() -> (w1997:dbl)
                        n1228 = Search 1D Array(1D array=w1985, element="STS-Sat (V/decade):") -> (index of element=w1992:i32)  [unwired: 1 in]
                        n1229 = Divide(x=w1992, y=3) -> (x/y=w1991:dbl)
                        n1230 = To Word Integer(number=w1991) -> (16bit integer=w1993:i16)
                        n1231 = Format Value(format string="%#g", value (0)=w1997) -> (output string=w1988:string)  [unwired: 1 in]
                        n1232 = Build Array(w1984, w1988) -> (w1995:string[])
                        n1233 = Increment(x=w1993) -> (x+1=w1994:i16)
                        n1234 = Insert Into Array(array=w1986, index (row)=w1994, new element=w1995) -> (w1987:string[][])  [unwired: 1 in]
                      }
                    }
                    n1235 = local write "Save1 Array"(w1970) -> ()
                  }
                  frame #13 {
                    w1998 = "Trap Density-STS (Traps/Vcm^2):"
                    n1236 = local read "Save1 Array"() -> (w2000:string[][])
                    n1237 = Array Size(array=w2000) -> (size(s)=w2005:i32[])
                    n1238 = Array Subset(array=w2000, index (row)=0, index (col)=0, length (col)=3) -> (w2001:string[][])  [unwired: 1 in]
                    n1239 = Index Array(array=w2005, index=0) -> (element=w2007:i32)
                    n1240 = Reshape Array(w2001, w2007) -> (w1999:string[])
                    n1241 = Search 1D Array(1D array=w1999, element=w1998) -> (index of element=w2010:i32)  [unwired: 1 in]
                    n1242 = Equal?(x=w2010, y=-1) -> (x = y?=w2009:bool)
                    n1243 = case shown="True" w2009 {
                      tunnel: w2000 -> [w2019 w2024]
                      tunnel: w2010 -> [w2016 _]
                      tunnel: [w2015 w2025] -> w2008
                      tunnel: w1999 -> [_ w2023]
                      tunnel: w1998 -> [_ w2022]
                      frame False {
                        n1244 = local read "New: Trap Density-STS"() -> (w2013:dbl)
                        n1245 = Divide(x=w2016, y=3) -> (x/y=w2018:dbl)
                        n1246 = To Word Integer(number=w2018) -> (16bit integer=w2017:i16)
                        n1247 = Format Value(format string="%#g", value (0)=w2013) -> (output string=w2012:string)  [unwired: 1 in]
                        n1248 = Replace Array Subset(array=w2019, new element=w2012, index (row)=w2017, index (col)=1) -> (w2015:string[][])
                      }
                      frame True {
                        n1249 = local read "New: Trap Density-STS"() -> (w2026:dbl)
                        n1250 = Search 1D Array(1D array=w2023, element="Trap Density-VT (Traps/Vcm^2):") -> (index of element=w2031:i32)  [unwired: 1 in]
                        n1251 = Divide(x=w2031, y=3) -> (x/y=w2032:dbl)
                        n1252 = To Word Integer(number=w2032) -> (16bit integer=w2030:i16)
                        n1253 = Format Value(format string="%#g", value (0)=w2026) -> (output string=w2035:string)  [unwired: 1 in]
                        n1254 = Build Array(w2022, w2035) -> (w2028:string[])
                        n1255 = Increment(x=w2030) -> (x+1=w2029:i16)
                        n1256 = Insert Into Array(array=w2024, index (row)=w2029, new element=w2028) -> (w2025:string[][])  [unwired: 1 in]
                      }
                    }
                    n1257 = local write "Save1 Array"(w2008) -> ()
                  }
                }
                n1258 = Concatenate Strings(w1573, "\\", w1571) -> (w1572:string)
                n1259 = String To Path(string=w1572) -> (path=w1562:path)
                n1260 = disable-structure shown="Disabled" {
                  frame Disabled {
                  }
                  frame Enabled {
                  }
                }
              }
              frame #2 {
                n1261 = Equal?(x=w2094, y=w2091) -> (x = y?=w2093:bool)
                n1262 = case shown="False" w2093 {
                  tunnel: w2094 -> [w2097 _]
                  tunnel: w2091 -> [w2096 _]
                  frame False {
                    n1263 = Move(source path=w2097, 9:TRUE, 10:w2096) -> ()  [unwired: 2 in, 3 out]
                  }
                  frame True {
                  }
                }
              }
              frame #3 {
                n1264 = local write "Transfer File"(w2098) -> ()
                n1265 = call-poly <vilib>:"Write To Spreadsheet File.vi"("2D data"=w2099, "file path (dialog if empty)"=w2098) -> ()  [unwired: 6 in, 1 out]
              }
            }
          }
          event "Save Changes? 2": Mouse Down {
            n1266 = event-data() -> ()  [unwired: 1 in, 5 out]
            n1267 = stacked-sequence {
              seq-local: [w2157 _ _ _ _] -> [_ w2640 _ _ _]
              seq-local: [w2156 _ _ _ _] -> [_ w2641 _ _ _]
              seq-local: [w2156 _ _ _ _] -> [_ w2639 _ _ _]
              seq-local: [w2158 _ _ _ _] -> [_ w2637 _ _ _]
              seq-local: [_ w2641 _ _ _] -> [_ _ w2646 _ _]
              seq-local: [_ w2637 _ _ _] -> [_ _ w2645 _ _]
              frame #0 {
                n1268 = local read "Transfer File"() -> (w2157:path)
                n1269 = local read "New: Temp"() -> (w2160:dbl)
                n1270 = local read "New: Length"() -> (w2163:dbl)
                n1271 = local read "New: Width"() -> (w2161:dbl)
                n1272 = To Word Integer(number=w2160) -> (16bit integer=w2159:i16)
                n1273 = Number To Decimal String(number=w2159) -> (decimal integer string=w2167:string)  [unwired: 1 in]
                n1274 = To Single Precision Float(number=w2161) -> (single precision float=w2162:sgl)
                n1275 = To Single Precision Float(number=w2163) -> (single precision float=w2164:sgl)
                n1276 = local read "Index"() -> (w2171:string)
                n1277 = Strip Path(path=w2157) -> (stripped path=w2176:path)  [unwired: 1 out]
                n1278 = Number To Decimal String(number=w2164) -> (decimal integer string=w2169:string)  [unwired: 1 in]
                n1279 = Number To Decimal String(number=w2162) -> (decimal integer string=w2170:string)  [unwired: 1 in]
                n1280 = Concatenate Strings("_", w2167, "K") -> (w2165:string)
                n1281 = call "Build Text2"("Temp"=w2165, "Index"=w2171, "Length"=w2169, "Width"=w2170) -> ("Result"=w2172:string)  [unwired: 10 in, 1 out]
                n1282 = Path To String(path=w2176) -> (string=w2174:string)
                n1283 = Concatenate Strings(w2174, "\\", w2172) -> (w2173:string)
                n1284 = stacked-sequence {
                  tunnel: [_ _ _ _ _ _ _ _ _ _ _ _ _ w2599] -> _
                  tunnel: w2157 -> [w2178 _ _ _ _ _ _ _ _ _ _ _ _ _]
                  tunnel: [_ _ _ _ _ _ _ _ _ _ _ _ _ w2599] -> w2158
                  frame #0 {
                    n1285 = call-poly <vilib>:"Read From Spreadsheet File.vi"("file path (dialog if empty)"=w2178) -> ("all rows"=w2177:string[][])  [unwired: 6 in, 4 out]
                    n1286 = Array Size(array=w2177) -> (size(s)=w2182:i32[])
                    n1287 = Array Subset(array=w2177, index (row)=0, index (col)=0, length (col)=3) -> (w2186:string[][])  [unwired: 1 in]
                    n1288 = Index Array(array=w2182, index=0) -> (element=w2180:i32)
                    n1289 = Reshape Array(w2186, w2180) -> (w2179:string[])
                    n1290 = Search 1D Array(1D array=w2179, element="Dielectric (nm):") -> (index of element=w2189:i32)  [unwired: 1 in]
                    n1291 = Equal?(x=w2189, y=-1) -> (x = y?=w2188:bool)
                    n1292 = case shown="False" w2188 {
                      tunnel: w2177 -> [w2197 w2201]
                      tunnel: w2189 -> [w2193 _]
                      tunnel: [w2192 w2201] -> w2187
                      frame False {
                        n1293 = local read "New: Dielectric"() -> (w2199:dbl)
                        n1294 = Number To Fractional String(number=w2199) -> (F-format string=w2194:string)  [unwired: 3 in]
                        n1295 = Divide(x=w2193, y=3) -> (x/y=w2196:dbl)
                        n1296 = To Word Integer(number=w2196) -> (16bit integer=w2195:i16)
                        n1297 = Replace Array Subset(array=w2197, new element=w2194, index (row)=w2195, index (col)=1) -> (w2192:string[][])
                      }
                      frame True {
                      }
                    }
                    n1298 = local write "Save1 Array"(w2187) -> ()
                  }
                  frame #1 {
                    n1299 = local read "Save1 Array"() -> (w2203:string[][])
                    n1300 = Array Size(array=w2203) -> (size(s)=w2206:i32[])
                    n1301 = Array Subset(array=w2203, index (row)=0, index (col)=0, length (col)=3) -> (w2210:string[][])  [unwired: 1 in]
                    n1302 = Index Array(array=w2206, index=0) -> (element=w2204:i32)
                    n1303 = Reshape Array(w2210, w2204) -> (w2202:string[])
                    n1304 = Search 1D Array(1D array=w2202, element="Comments:") -> (index of element=w2213:i32)  [unwired: 1 in]
                    n1305 = Equal?(x=w2213, y=-1) -> (x = y?=w2212:bool)
                    n1306 = case shown="False" w2212 {
                      tunnel: w2203 -> [w2221 w2224]
                      tunnel: w2213 -> [w2218 _]
                      tunnel: [w2217 w2224] -> w2211
                      frame False {
                        n1307 = local read "Comments:"() -> (w2216:string)
                        n1308 = Divide(x=w2218, y=3) -> (x/y=w2220:dbl)
                        n1309 = To Word Integer(number=w2220) -> (16bit integer=w2219:i16)
                        n1310 = Replace Array Subset(array=w2221, new element=w2216, index (row)=w2219, index (col)=1) -> (w2217:string[][])
                      }
                      frame True {
                      }
                    }
                    n1311 = local write "Save1 Array"(w2211) -> ()
                  }
                  frame #2 {
                    n1312 = local read "Save1 Array"() -> (w2226:string[][])
                    n1313 = Array Size(array=w2226) -> (size(s)=w2229:i32[])
                    n1314 = Array Subset(array=w2226, index (row)=0, index (col)=0, length (col)=3) -> (w2233:string[][])  [unwired: 1 in]
                    n1315 = Index Array(array=w2229, index=0) -> (element=w2227:i32)
                    n1316 = Reshape Array(w2233, w2227) -> (w2225:string[])
                    n1317 = Search 1D Array(1D array=w2225, element="Length (um):") -> (index of element=w2236:i32)  [unwired: 1 in]
                    n1318 = Equal?(x=w2236, y=-1) -> (x = y?=w2235:bool)
                    n1319 = case shown="False" w2235 {
                      tunnel: w2226 -> [w2246 w2249]
                      tunnel: w2236 -> [w2243 _]
                      tunnel: [w2242 w2249] -> w2234
                      frame False {
                        n1320 = local read "New: Length"() -> (w2239:dbl)
                        n1321 = Divide(x=w2243, y=3) -> (x/y=w2245:dbl)
                        n1322 = Format Value(format string="%#g", value (0)=w2239) -> (output string=w2240:string)  [unwired: 1 in]
                        n1323 = To Word Integer(number=w2245) -> (16bit integer=w2244:i16)
                        n1324 = Replace Array Subset(array=w2246, new element=w2240, index (row)=w2244, index (col)=1) -> (w2242:string[][])
                      }
                      frame True {
                      }
                    }
                    n1325 = local write "Save1 Array"(w2234) -> ()
                  }
                  frame #3 {
                    n1326 = local read "Save1 Array"() -> (w2251:string[][])
                    n1327 = Array Size(array=w2251) -> (size(s)=w2256:i32[])
                    n1328 = Array Subset(array=w2251, index (row)=0, index (col)=0, length (col)=3) -> (w2252:string[][])  [unwired: 1 in]
                    n1329 = Index Array(array=w2256, index=0) -> (element=w2258:i32)
                    n1330 = Reshape Array(w2252, w2258) -> (w2250:string[])
                    n1331 = Search 1D Array(1D array=w2250, element="Width (um):") -> (index of element=w2261:i32)  [unwired: 1 in]
                    n1332 = Equal?(x=w2261, y=-1) -> (x = y?=w2260:bool)
                    n1333 = case shown="False" w2260 {
                      tunnel: w2261 -> [w2269 _]
                      tunnel: w2251 -> [w2268 w2274]
                      tunnel: [w2267 w2274] -> w2259
                      frame False {
                        n1334 = local read "New: Width"() -> (w2264:dbl)
                        n1335 = Divide(x=w2269, y=3) -> (x/y=w2271:dbl)
                        n1336 = To Word Integer(number=w2271) -> (16bit integer=w2270:i16)
                        n1337 = Format Value(format string="%#g", value (0)=w2264) -> (output string=w2265:string)  [unwired: 1 in]
                        n1338 = Replace Array Subset(array=w2268, new element=w2265, index (row)=w2270, index (col)=1) -> (w2267:string[][])
                      }
                      frame True {
                      }
                    }
                    n1339 = local write "Save1 Array"(w2259) -> ()
                  }
                  frame #4 {
                    w2284 = "Sample Temp (K):"
                    n1340 = local read "Save1 Array"() -> (w2276:string[][])
                    n1341 = Array Size(array=w2276) -> (size(s)=w2281:i32[])
                    n1342 = Array Subset(array=w2276, index (row)=0, index (col)=0, length (col)=3) -> (w2277:string[][])  [unwired: 1 in]
                    n1343 = Index Array(array=w2281, index=0) -> (element=w2283:i32)
                    n1344 = Reshape Array(w2277, w2283) -> (w2275:string[])
                    n1345 = Search 1D Array(1D array=w2275, element=w2284) -> (index of element=w2287:i32)  [unwired: 1 in]
                    n1346 = Equal?(x=w2287, y=-1) -> (x = y?=w2286:bool)
                    n1347 = case shown="True" w2286 {
                      tunnel: w2276 -> [w2296 w2310]
                      tunnel: w2287 -> [w2293 _]
                      tunnel: [w2292 w2309] -> w2285
                      tunnel: w2275 -> [_ w2312]
                      tunnel: w2284 -> [_ w2299]
                      frame False {
                        n1348 = local read "New: Temp"() -> (w2290:dbl)
                        n1349 = Divide(x=w2293, y=3) -> (x/y=w2295:dbl)
                        n1350 = Format Value(format string="%#g", value (0)=w2290) -> (output string=w2289:string)  [unwired: 1 in]
                        n1351 = To Word Integer(number=w2295) -> (16bit integer=w2294:i16)
                        n1352 = Replace Array Subset(array=w2296, new element=w2289, index (row)=w2294, index (col)=1) -> (w2292:string[][])
                      }
                      frame True {
                        n1353 = local read "New: Temp"() -> (w2301:dbl)
                        n1354 = Search 1D Array(1D array=w2312, element="Width (um):") -> (index of element=w2306:i32)  [unwired: 1 in]
                        n1355 = Divide(x=w2306, y=3) -> (x/y=w2307:dbl)
                        n1356 = To Word Integer(number=w2307) -> (16bit integer=w2305:i16)
                        n1357 = Format Value(format string="%#g", value (0)=w2301) -> (output string=w2300:string)  [unwired: 1 in]
                        n1358 = Build Array(w2299, w2300) -> (w2303:string[])
                        n1359 = Increment(x=w2305) -> (x+1=w2304:i16)
                        n1360 = Insert Into Array(array=w2310, index (row)=w2304, new element=w2303) -> (w2309:string[][])  [unwired: 1 in]
                      }
                    }
                    n1361 = local write "Save1 Array"(w2285) -> ()
                  }
                  frame #5 {
                    w2322 = "Mobility-Sat (cm^2/Vs):"
                    n1362 = local read "Save1 Array"() -> (w2314:string[][])
                    n1363 = Array Size(array=w2314) -> (size(s)=w2319:i32[])
                    n1364 = Array Subset(array=w2314, index (row)=0, index (col)=0, length (col)=3) -> (w2315:string[][])  [unwired: 1 in]
                    n1365 = Index Array(array=w2319, index=0) -> (element=w2321:i32)
                    n1366 = Reshape Array(w2315, w2321) -> (w2313:string[])
                    n1367 = Search 1D Array(1D array=w2313, element=w2322) -> (index of element=w2325:i32)  [unwired: 1 in]
                    n1368 = Equal?(x=w2325, y=-1) -> (x = y?=w2324:bool)
                    n1369 = case shown="True" w2324 {
                      tunnel: w2314 -> [w2334 w2342]
                      tunnel: w2325 -> [w2331 _]
                      tunnel: [w2330 w2341] -> w2323
                      tunnel: w2313 -> [_ w2339]
                      tunnel: w2322 -> [_ w2337]
                      frame False {
                        n1370 = local read "New: Mobility-Sat"() -> (w2327:dbl)
                        n1371 = Divide(x=w2331, y=3) -> (x/y=w2333:dbl)
                        n1372 = To Word Integer(number=w2333) -> (16bit integer=w2332:i16)
                        n1373 = Format Value(format string="%#g", value (0)=w2327) -> (output string=w2328:string)  [unwired: 1 in]
                        n1374 = Replace Array Subset(array=w2334, new element=w2328, index (row)=w2332, index (col)=1) -> (w2330:string[][])
                      }
                      frame True {
                        n1375 = local read "New: Mobility-Sat"() -> (w2343:dbl)
                        n1376 = Search 1D Array(1D array=w2339, element="Mobility (cm^2/Vs):") -> (index of element=w2346:i32)  [unwired: 1 in]
                        n1377 = Divide(x=w2346, y=3) -> (x/y=w2347:dbl)
                        n1378 = To Word Integer(number=w2347) -> (16bit integer=w2338:i16)
                        n1379 = Format Value(format string="%#g", value (0)=w2343) -> (output string=w2340:string)  [unwired: 1 in]
                        n1380 = Build Array(w2337, w2340) -> (w2345:string[])
                        n1381 = Replace Array Subset(array=w2342, new element=w2345, index (row)=w2338) -> (w2341:string[][])  [unwired: 1 in]
                      }
                    }
                    n1382 = local write "Save1 Array"(w2323) -> ()
                  }
                  frame #6 {
                    w2359 = "Mobility-Lin (cm^2/Vs):"
                    n1383 = local read "Save1 Array"() -> (w2350:string[][])
                    n1384 = Array Size(array=w2350) -> (size(s)=w2356:i32[])
                    n1385 = Array Subset(array=w2350, index (row)=0, index (col)=0, length (col)=3) -> (w2352:string[][])  [unwired: 1 in]
                    n1386 = Index Array(array=w2356, index=0) -> (element=w2358:i32)
                    n1387 = Reshape Array(w2352, w2358) -> (w2351:string[])
                    n1388 = Search 1D Array(1D array=w2351, element=w2359) -> (index of element=w2362:i32)  [unwired: 1 in]
                    n1389 = Equal?(x=w2362, y=-1) -> (x = y?=w2361:bool)
                    n1390 = case shown="True" w2361 {
                      tunnel: w2350 -> [w2371 w2377]
                      tunnel: w2362 -> [w2368 _]
                      tunnel: [w2367 w2376] -> w2360
                      tunnel: w2351 -> [_ w2375]
                      tunnel: w2359 -> [_ w2374]
                      frame False {
                        n1391 = local read "Calc: Mobility-Lin"() -> (w2364:dbl)
                        n1392 = Divide(x=w2368, y=3) -> (x/y=w2370:dbl)
                        n1393 = To Word Integer(number=w2370) -> (16bit integer=w2369:i16)
                        n1394 = Format Value(format string="%#g", value (0)=w2364) -> (output string=w2365:string)  [unwired: 1 in]
                        n1395 = Replace Array Subset(array=w2371, new element=w2365, index (row)=w2369, index (col)=1) -> (w2367:string[][])
                      }
                      frame True {
                        n1396 = local read "Calc: Mobility-Lin"() -> (w2378:dbl)
                        n1397 = Search 1D Array(1D array=w2375, element="Mobility-Sat (cm^2/Vs):") -> (index of element=w2383:i32)  [unwired: 1 in]
                        n1398 = Divide(x=w2383, y=3) -> (x/y=w2384:dbl)
                        n1399 = To Word Integer(number=w2384) -> (16bit integer=w2382:i16)
                        n1400 = Format Value(format string="%#g", value (0)=w2378) -> (output string=w2387:string)  [unwired: 1 in]
                        n1401 = Build Array(w2374, w2387) -> (w2380:string[])
                        n1402 = Increment(x=w2382) -> (x+1=w2381:i16)
                        n1403 = Insert Into Array(array=w2377, index (row)=w2381, new element=w2380) -> (w2376:string[][])  [unwired: 1 in]
                      }
                    }
                    n1404 = local write "Save1 Array"(w2360) -> ()
                  }
                  frame #7 {
                    w2397 = "On/Off I-Sat:"
                    n1405 = local read "Save1 Array"() -> (w2388:string[][])
                    n1406 = Array Size(array=w2388) -> (size(s)=w2394:i32[])
                    n1407 = Array Subset(array=w2388, index (row)=0, index (col)=0, length (col)=3) -> (w2390:string[][])  [unwired: 1 in]
                    n1408 = Index Array(array=w2394, index=0) -> (element=w2396:i32)
                    n1409 = Reshape Array(w2390, w2396) -> (w2389:string[])
                    n1410 = Search 1D Array(1D array=w2389, element=w2397) -> (index of element=w2400:i32)  [unwired: 1 in]
                    n1411 = Equal?(x=w2400, y=-1) -> (x = y?=w2399:bool)
                    n1412 = case shown="True" w2399 {
                      tunnel: w2388 -> [w2409 w2416]
                      tunnel: w2400 -> [w2406 _]
                      tunnel: [w2405 w2417] -> w2398
                      tunnel: w2389 -> [_ w2414]
                      tunnel: w2397 -> [_ w2412]
                      frame False {
                        n1413 = local read "Calc: On/Off"() -> (w2402:dbl)
                        n1414 = Divide(x=w2406, y=3) -> (x/y=w2408:dbl)
                        n1415 = To Word Integer(number=w2408) -> (16bit integer=w2407:i16)
                        n1416 = Format Value(format string="%#g", value (0)=w2402) -> (output string=w2403:string)  [unwired: 1 in]
                        n1417 = Replace Array Subset(array=w2409, new element=w2403, index (row)=w2407, index (col)=1) -> (w2405:string[][])
                      }
                      frame True {
                        n1418 = local read "Calc: On/Off"() -> (w2418:dbl)
                        n1419 = Search 1D Array(1D array=w2414, element="On/Off Current:") -> (index of element=w2421:i32)  [unwired: 1 in]
                        n1420 = Divide(x=w2421, y=3) -> (x/y=w2422:dbl)
                        n1421 = To Word Integer(number=w2422) -> (16bit integer=w2413:i16)
                        n1422 = Format Value(format string="%#g", value (0)=w2418) -> (output string=w2415:string)  [unwired: 1 in]
                        n1423 = Build Array(w2412, w2415) -> (w2420:string[])
                        n1424 = Replace Array Subset(array=w2416, new element=w2420, index (row)=w2413) -> (w2417:string[][])  [unwired: 1 in]
                      }
                    }
                    n1425 = local write "Save1 Array"(w2398) -> ()
                  }
                  frame #8 {
                    w2434 = "Off I-Sat (A):"
                    n1426 = local read "Save1 Array"() -> (w2425:string[][])
                    n1427 = Array Size(array=w2425) -> (size(s)=w2431:i32[])
                    n1428 = Array Subset(array=w2425, index (row)=0, index (col)=0, length (col)=3) -> (w2427:string[][])  [unwired: 1 in]
                    n1429 = Index Array(array=w2431, index=0) -> (element=w2433:i32)
                    n1430 = Reshape Array(w2427, w2433) -> (w2426:string[])
                    n1431 = Search 1D Array(1D array=w2426, element=w2434) -> (index of element=w2437:i32)  [unwired: 1 in]
                    n1432 = Equal?(x=w2437, y=-1) -> (x = y?=w2436:bool)
                    n1433 = case shown="True" w2436 {
                      tunnel: w2425 -> [w2446 w2452]
                      tunnel: w2437 -> [w2443 _]
                      tunnel: [w2442 w2451] -> w2435
                      tunnel: w2426 -> [_ w2450]
                      tunnel: w2434 -> [_ w2449]
                      frame False {
                        n1434 = local read "Calc: Off I-Sat"() -> (w2441:dbl)
                        n1435 = Divide(x=w2443, y=3) -> (x/y=w2445:dbl)
                        n1436 = Format Value(format string="%#g", value (0)=w2441) -> (output string=w2439:string)  [unwired: 1 in]
                        n1437 = To Word Integer(number=w2445) -> (16bit integer=w2444:i16)
                        n1438 = Replace Array Subset(array=w2446, new element=w2439, index (row)=w2444, index (col)=1) -> (w2442:string[][])
                      }
                      frame True {
                        n1439 = local read "Calc: Off I-Sat"() -> (w2453:dbl)
                        n1440 = Search 1D Array(1D array=w2450, element="On/Off I-Sat:") -> (index of element=w2458:i32)  [unwired: 1 in]
                        n1441 = Divide(x=w2458, y=3) -> (x/y=w2459:dbl)
                        n1442 = To Word Integer(number=w2459) -> (16bit integer=w2457:i16)
                        n1443 = Format Value(format string="%#g", value (0)=w2453) -> (output string=w2462:string)  [unwired: 1 in]
                        n1444 = Build Array(w2449, w2462) -> (w2455:string[])
                        n1445 = Increment(x=w2457) -> (x+1=w2456:i16)
                        n1446 = Insert Into Array(array=w2452, index (row)=w2456, new element=w2455) -> (w2451:string[][])  [unwired: 1 in]
                      }
                    }
                    n1447 = local write "Save1 Array"(w2435) -> ()
                  }
                  frame #9 {
                    w2464 = "Vt-Sat (V):"
                    n1448 = local read "Save1 Array"() -> (w2465:string[][])
                    n1449 = Array Size(array=w2465) -> (size(s)=w2470:i32[])
                    n1450 = Array Subset(array=w2465, index (row)=0, index (col)=0, length (col)=3) -> (w2466:string[][])  [unwired: 1 in]
                    n1451 = Index Array(array=w2470, index=0) -> (element=w2472:i32)
                    n1452 = Reshape Array(w2466, w2472) -> (w2463:string[])
                    n1453 = Search 1D Array(1D array=w2463, element=w2464) -> (index of element=w2475:i32)  [unwired: 1 in]
                    n1454 = Equal?(x=w2475, y=-1) -> (x = y?=w2474:bool)
                    n1455 = case shown="True" w2474 {
                      tunnel: w2465 -> [w2482 w2491]
                      tunnel: w2475 -> [w2478 _]
                      tunnel: [w2477 w2490] -> w2473
                      tunnel: w2464 -> [_ w2489]
                      tunnel: w2463 -> [_ w2488]
                      frame False {
                        n1456 = local read "New: VT-Sat"() -> (w2484:dbl)
                        n1457 = Number To Fractional String(number=w2484) -> (F-format string=w2479:string)  [unwired: 3 in]
                        n1458 = Divide(x=w2478, y=3) -> (x/y=w2481:dbl)
                        n1459 = To Word Integer(number=w2481) -> (16bit integer=w2480:i16)
                        n1460 = Replace Array Subset(array=w2482, new element=w2479, index (row)=w2480, index (col)=1) -> (w2477:string[][])
                      }
                      frame True {
                        n1461 = local read "New: VT-Sat"() -> (w2492:dbl)
                        n1462 = Search 1D Array(1D array=w2488, element="Threshold V (V):") -> (index of element=w2487:i32)  [unwired: 1 in]
                        n1463 = Divide(x=w2487, y=3) -> (x/y=w2495:dbl)
                        n1464 = To Word Integer(number=w2495) -> (16bit integer=w2486:i16)
                        n1465 = Format Value(format string="%#g", value (0)=w2492) -> (output string=w2498:string)  [unwired: 1 in]
                        n1466 = Build Array(w2489, w2498) -> (w2494:string[])
                        n1467 = Replace Array Subset(array=w2491, new element=w2494, index (row)=w2486) -> (w2490:string[][])  [unwired: 1 in]
                      }
                    }
                    n1468 = local write "Save1 Array"(w2473) -> ()
                  }
                  frame #10 {
                    n1469 = local read "Save1 Array"() -> (w2499:string[][])
                    n1470 = Array Size(array=w2499) -> (size(s)=w2505:i32[])
                    n1471 = Array Subset(array=w2499, index (row)=0, index (col)=0, length (col)=3) -> (w2501:string[][])  [unwired: 1 in]
                    n1472 = Index Array(array=w2505, index=0) -> (element=w2507:i32)
                    n1473 = Reshape Array(w2501, w2507) -> (w2500:string[])
                    n1474 = Search 1D Array(1D array=w2500, element="VT-Lin (V):") -> (index of element=w2510:i32)  [unwired: 1 in]
                    n1475 = Equal?(x=w2510, y=-1) -> (x = y?=w2509:bool)
                    n1476 = case shown="False" w2509 {
                      tunnel: w2499 -> [w2520 w2523]
                      tunnel: w2510 -> [w2517 _]
                      tunnel: [w2516 w2523] -> w2508
                      frame False {
                        n1477 = local read "New: VT-Lin"() -> (w2514:dbl)
                        n1478 = Divide(x=w2517, y=3) -> (x/y=w2519:dbl)
                        n1479 = Format Value(format string="%#g", value (0)=w2514) -> (output string=w2513:string)  [unwired: 1 in]
                        n1480 = To Word Integer(number=w2519) -> (16bit integer=w2518:i16)
                        n1481 = Replace Array Subset(array=w2520, new element=w2513, index (row)=w2518, index (col)=1) -> (w2516:string[][])
                      }
                      frame True {
                      }
                    }
                    n1482 = local write "Save1 Array"(w2508) -> ()
                  }
                  frame #11 {
                    w2524 = "STS-Sat (V/decade):"
                    n1483 = local read "Save1 Array"() -> (w2526:string[][])
                    n1484 = Array Size(array=w2526) -> (size(s)=w2531:i32[])
                    n1485 = Array Subset(array=w2526, index (row)=0, index (col)=0, length (col)=3) -> (w2527:string[][])  [unwired: 1 in]
                    n1486 = Index Array(array=w2531, index=0) -> (element=w2533:i32)
                    n1487 = Reshape Array(w2527, w2533) -> (w2525:string[])
                    n1488 = Search 1D Array(1D array=w2525, element=w2524) -> (index of element=w2536:i32)  [unwired: 1 in]
                    n1489 = Equal?(x=w2536, y=-1) -> (x = y?=w2535:bool)
                    n1490 = case shown="True" w2535 {
                      tunnel: w2526 -> [w2545 w2551]
                      tunnel: w2536 -> [w2542 _]
                      tunnel: [w2541 w2552] -> w2534
                      tunnel: w2525 -> [_ w2550]
                      tunnel: w2524 -> [_ w2549]
                      frame False {
                        n1491 = local read "New: STS"() -> (w2539:dbl)
                        n1492 = Divide(x=w2542, y=3) -> (x/y=w2544:dbl)
                        n1493 = Format Value(format string="%#g", value (0)=w2539) -> (output string=w2538:string)  [unwired: 1 in]
                        n1494 = To Word Integer(number=w2544) -> (16bit integer=w2543:i16)
                        n1495 = Replace Array Subset(array=w2545, new element=w2538, index (row)=w2543, index (col)=1) -> (w2541:string[][])
                      }
                      frame True {
                        n1496 = local read "New: STS"() -> (w2553:dbl)
                        n1497 = Search 1D Array(1D array=w2550, element="S.T.S. (V/decade):") -> (index of element=w2556:i32)  [unwired: 1 in]
                        n1498 = Divide(x=w2556, y=3) -> (x/y=w2557:dbl)
                        n1499 = To Word Integer(number=w2557) -> (16bit integer=w2548:i16)
                        n1500 = Format Value(format string="%#g", value (0)=w2553) -> (output string=w2560:string)  [unwired: 1 in]
                        n1501 = Build Array(w2549, w2560) -> (w2555:string[])
                        n1502 = Replace Array Subset(array=w2551, new element=w2555, index (row)=w2548) -> (w2552:string[][])  [unwired: 1 in]
                      }
                    }
                    n1503 = local write "Save1 Array"(w2534) -> ()
                  }
                  frame #12 {
                    w2561 = "Trap Density-VT (Traps/Vcm^2):"
                    n1504 = local read "Save1 Array"() -> (w2563:string[][])
                    n1505 = Array Size(array=w2563) -> (size(s)=w2568:i32[])
                    n1506 = Array Subset(array=w2563, index (row)=0, index (col)=0, length (col)=3) -> (w2564:string[][])  [unwired: 1 in]
                    n1507 = Index Array(array=w2568, index=0) -> (element=w2570:i32)
                    n1508 = Reshape Array(w2564, w2570) -> (w2562:string[])
                    n1509 = Search 1D Array(1D array=w2562, element=w2561) -> (index of element=w2573:i32)  [unwired: 1 in]
                    n1510 = Equal?(x=w2573, y=-1) -> (x = y?=w2572:bool)
                    n1511 = case shown="True" w2572 {
                      tunnel: w2563 -> [w2582 w2587]
                      tunnel: w2573 -> [w2578 _]
                      tunnel: [w2577 w2588] -> w2571
                      tunnel: w2562 -> [_ w2586]
                      tunnel: w2561 -> [_ w2585]
                      frame False {
                        n1512 = local read "New: Trap Density-VT"() -> (w2576:dbl)
                        n1513 = Format Value(format string="%#g", value (0)=w2576) -> (output string=w2579:string)  [unwired: 1 in]
                        n1514 = Divide(x=w2578, y=3) -> (x/y=w2581:dbl)
                        n1515 = To Word Integer(number=w2581) -> (16bit integer=w2580:i16)
                        n1516 = Replace Array Subset(array=w2582, new element=w2579, index (row)=w2580, index (col)=1) -> (w2577:string[][])
                      }
                      frame True {
                        n1517 = local read "New: Trap Density-VT"() -> (w2598:dbl)
                        n1518 = Search 1D Array(1D array=w2586, element="STS-Sat (V/decade):") -> (index of element=w2593:i32)  [unwired: 1 in]
                        n1519 = Divide(x=w2593, y=3) -> (x/y=w2592:dbl)
                        n1520 = To Word Integer(number=w2592) -> (16bit integer=w2594:i16)
                        n1521 = Format Value(format string="%#g", value (0)=w2598) -> (output string=w2589:string)  [unwired: 1 in]
                        n1522 = Build Array(w2585, w2589) -> (w2596:string[])
                        n1523 = Increment(x=w2594) -> (x+1=w2595:i16)
                        n1524 = Insert Into Array(array=w2587, index (row)=w2595, new element=w2596) -> (w2588:string[][])  [unwired: 1 in]
                      }
                    }
                    n1525 = local write "Save1 Array"(w2571) -> ()
                  }
                  frame #13 {
                    w2600 = "Trap Density-STS (Traps/Vcm^2):"
                    n1526 = local read "Save1 Array"() -> (w2602:string[][])
                    n1527 = Array Size(array=w2602) -> (size(s)=w2607:i32[])
                    n1528 = Array Subset(array=w2602, index (row)=0, index (col)=0, length (col)=3) -> (w2603:string[][])  [unwired: 1 in]
                    n1529 = Index Array(array=w2607, index=0) -> (element=w2609:i32)
                    n1530 = Reshape Array(w2603, w2609) -> (w2601:string[])
                    n1531 = Search 1D Array(1D array=w2601, element=w2600) -> (index of element=w2611:i32)  [unwired: 1 in]
                    n1532 = Equal?(x=w2611, y=-1) -> (x = y?=w2610:bool)
                    n1533 = case shown="True" w2610 {
                      tunnel: w2602 -> [w2620 w2625]
                      tunnel: w2611 -> [w2617 _]
                      tunnel: [w2616 w2626] -> w2599
                      tunnel: w2601 -> [_ w2624]
                      tunnel: w2600 -> [_ w2623]
                      frame False {
                        n1534 = local read "New: Trap Density-STS"() -> (w2614:dbl)
                        n1535 = Divide(x=w2617, y=3) -> (x/y=w2619:dbl)
                        n1536 = To Word Integer(number=w2619) -> (16bit integer=w2618:i16)
                        n1537 = Format Value(format string="%#g", value (0)=w2614) -> (output string=w2613:string)  [unwired: 1 in]
                        n1538 = Replace Array Subset(array=w2620, new element=w2613, index (row)=w2618, index (col)=1) -> (w2616:string[][])
                      }
                      frame True {
                        n1539 = local read "New: Trap Density-STS"() -> (w2627:dbl)
                        n1540 = Search 1D Array(1D array=w2624, element="Trap Density-VT (Traps/Vcm^2):") -> (index of element=w2632:i32)  [unwired: 1 in]
                        n1541 = Divide(x=w2632, y=3) -> (x/y=w2633:dbl)
                        n1542 = To Word Integer(number=w2633) -> (16bit integer=w2631:i16)
                        n1543 = Format Value(format string="%#g", value (0)=w2627) -> (output string=w2636:string)  [unwired: 1 in]
                        n1544 = Build Array(w2623, w2636) -> (w2629:string[])
                        n1545 = Increment(x=w2631) -> (x+1=w2630:i16)
                        n1546 = Insert Into Array(array=w2625, index (row)=w2630, new element=w2629) -> (w2626:string[][])  [unwired: 1 in]
                      }
                    }
                    n1547 = local write "Save1 Array"(w2599) -> ()
                  }
                }
                n1548 = String To Path(string=w2173) -> (path=w2156:path)
                "No Image 2" <- w2156
              }
              frame #1 {
                n1549 = Equal?(x=w2640, y=w2639) -> (x = y?=w2638:bool)
                n1550 = case shown="False" w2638 {
                  tunnel: w2640 -> [w2644 _]
                  tunnel: w2639 -> [w2643 _]
                  frame False {
                    n1551 = Move(source path=w2644, 9:TRUE, 10:w2643) -> ()  [unwired: 2 in, 3 out]
                  }
                  frame True {
                  }
                }
              }
              frame #2 {
                n1552 = local write "Transfer File"(w2646) -> ()
                n1553 = call-poly <vilib>:"Write To Spreadsheet File.vi"("2D data"=w2645, "file path (dialog if empty)"=w2646) -> ()  [unwired: 6 in, 1 out]
              }
              frame #3 {
                w2672 = 0
                w2779 = 0
                # "Moves to next file and displays new image/data"
                n1554 = property on="Image Out" class="ImageControl"() -> (error out=w2742:errorcluster, "Image Center Position"=w2746:cluster{"X":u32, "Y":u32})  [unwired: 2 in, 1 out]
                n1555 = local read "Transfer File"() -> (w2649:path)
                n1556 = Strip Path(path=w2649) -> (stripped path=w2677:path, name=w2791:string)
                n1557 = Unbundle(w2746) -> ("X"=w2744:u32)  [unwired: 1 out]
                n1558 = local write "Transfer Folder"(w2677) -> ()
                n1559 = Bundle("X"=w2744, 0) -> (w2745:cluster{"X":u32, i32})  [unwired: 1 in]
                n1560 = local read "Transport Style Controls"() -> (w2648:T4)
                n1561 = property on="Image Out" class="ImageControl"(error in=w2742, "Image Center Position"=w2745) -> ()  [unwired: 1 in, 2 out]
                n1562 = List Folder(path=w2677) -> (filenames=w2788:string[])  [unwired: 3 in, 3 out]
                n1563 = call "TRF to TSP Plot.vi"("Transport Graph Properties"=w2648, "Transfer File"=w2649) -> ("Transport"=w2647:cluster{ext[], ext[]}[])  [unwired: 7 in, 2 out]
                n1564 = Search 1D Array(1D array=w2788, element=w2791) -> (index of element=w2785:i32)  [unwired: 1 in]
                n1565 = Array Size(array=w2788) -> (size(s)=w2784:i32)
                n1566 = Decrement(x=w2784) -> (x-1=w2786:i32)
                n1567 = local write "Transport"(w2647) -> ()
                n1568 = Equal?(x=w2785, y=w2786) -> (x = y?=w2787:bool)
                n1569 = local read "Folder Index"() -> (w2738:dbl)
                n1570 = case shown="False" w2787 {
                  tunnel: w2738 -> [w2916 _]
                  tunnel: [w2915 0] -> w2737
                  frame False {
                    n1571 = Increment(x=w2916) -> (x+1=w2915:dbl)
                  }
                  frame True {
                  }
                }
                n1572 = invoke on="Image Out" class="ImageControl" method="Clear ROI"() -> ()  [unwired: 3 in, 3 out]
                n1573 = local write "Folder Index"(w2737) -> ()
                n1574 = Path To String(path=w2677) -> (string=w2792:string)
                n1575 = Index Array(array=w2788, index=w2737) -> (element=w2676:string)
                n1576 = local write "Data Name:"(w2676) -> ()
                n1577 = Concatenate Strings(w2792, "\\", w2676) -> (w2790:string)
                n1578 = String To Path(string=w2790) -> (path=w2650:path)
                n1579 = call "Recorded Values.vi"("Path"=w2650) -> ("Recorded Char"=w2693:T7, "Recorded Prop"=w2694:T8, "Fabrication Prop"=w2692:T9)  [unwired: 8 in]
                n1580 = Unbundle By Name(w2693) -> ("Mobility-Sat"=w2706:dbl, "Moblitity-Lin"=w2707:dbl, "On/Off"=w2708:dbl, "Off Current"=w2709:dbl, "Vt-Sat"=w2686:dbl, "STS"=w2710:dbl, "Trap Density-VT"=w2711:dbl, "Trap Density-STS"=w2712:dbl)
                n1581 = Unbundle By Name(w2694) -> ("Date Recorded"=w2702:string, "Index"=w2703:string, "Length"=w2704:dbl, "Width"=w2705:dbl, "Sample Temp"=w2689:dbl)
                n1582 = Unbundle By Name(w2692) -> ("Date Created"=w2713:string, "Material"=w2695:string, "Solvent"=w2696:string, "Concentration"=w2697:dbl, "Method"=w2698:string, "Dielectric (nm)"=w2699:dbl, "Treatment"=w2700:string, "Comments"=w2701:string)
                n1583 = local write "Rec: Off I-Sat"(w2709) -> ()
                n1584 = local write "Rec: Comments"(w2701) -> ()
                n1585 = local write "Rec: VT-Sat"(w2686) -> ()
                n1586 = local write "Date Created"(w2713) -> ()
                n1587 = local write "Rec: Material"(w2695) -> ()
                n1588 = local write "Rec: Solvent"(w2696) -> ()
                n1589 = local write "Rec: Concentration"(w2697) -> ()
                n1590 = local write "Rec: Method"(w2698) -> ()
                n1591 = local write "Rec: Dielectric (d)"(w2699) -> ()
                n1592 = local write "Surface Treatment:"(w2700) -> ()
                n1593 = local write "Index"(w2703) -> ()
                n1594 = local write "Rec: Mobility-Sat"(w2706) -> ()
                n1595 = local write "Rec: Mobility-Lin"(w2707) -> ()
                n1596 = local write "Rec: On/Off"(w2708) -> ()
                n1597 = local write "Rec: STS"(w2710) -> ()
                n1598 = local write "Rec: Trap Density-VT"(w2711) -> ()
                n1599 = local write "Rec: Trap Density-STS"(w2712) -> ()
                n1600 = local write "Date Recorded"(w2702) -> ()
                n1601 = local write "Rec: Length"(w2704) -> ()
                n1602 = local write "Rec: Width"(w2705) -> ()
                n1603 = local write "Rec: Temp"(w2689) -> ()
                n1604 = Equal To 0?(x=w2689) -> (x = 0?=w2690:bool)
                n1605 = case shown="False" w2690 {
                  tunnel: [w2793 w2794] -> w2687
                  tunnel: w2689 -> [w2793 _]
                  frame False {
                  }
                  frame True {
                    n1606 = local read "Room Temp"() -> (w2794:dbl)
                  }
                }
                n1607 = local read "NumPoints Log"() -> (w2734:dbl)
                n1608 = local write "Transfer File"(w2650) -> ()
                n1609 = local read "Num Pts"() -> (w2723:dbl)
                n1610 = local read "Num Pts"() -> (w2735:dbl)
                n1611 = call-poly <vilib>:"Read From Spreadsheet File.vi"("file path (dialog if empty)"=w2650) -> ("all rows"=w2781:string[][])  [unwired: 6 in, 4 out]
                n1612 = call "Mobility-Vt Calculator-File.vi"("NumPts"=w2735, "Path"=w2650) -> ("Graph Cluster"=w2683:T11, "Output"=w2736:T12, 4:w2716, 5:w2722)  [unwired: 4 in, 2 out]
                n1613 = Unbundle By Name(w2683) -> ("Raw Sat"=w2680:cluster{dbl[], dbl[]}[], "Sqrt Sat"=w2682:cluster{dbl[], dbl[]}[], "Raw Lin"=w2679:cluster{dbl[], dbl[]}[], "Sqrt Lin"=w2681:cluster{dbl[], dbl[]}[], "Log Lin"=w2678:cluster{dbl[], dbl[]}[])  [unwired: 1 out]
                n1614 = Decimate 1D Array(w2681) -> (w2730:cluster{dbl[], dbl[]}[])  [unwired: 1 out]
                n1615 = Array To Cluster(array=w2730) -> (cluster=w2728:T13)
                n1616 = Unbundle(w2728) -> ("[0]"=w2729:cluster{dbl[], dbl[]})  [unwired: 8 out]
                n1617 = Unbundle(w2729) -> (w2727:dbl[], w2726:dbl[])
                n1618 = Array Subset(array=w2726, index=w2722, length=w2723) -> (w2724:dbl[])
                n1619 = Array Subset(array=w2727, index=w2722, length=w2723) -> (w2725:dbl[])
                n1620 = call "STS Calculator-File.vi"("NumPts"=w2734, "Path"=w2650) -> ("Used Points"=w2733:T10, "XY Graph-Sat"=w2732:cluster{dbl[], dbl[]}[], "Ouput"=w2731:cluster{"STS-Sat":dbl, "STS-Lin":dbl})  [unwired: 6 in, 1 out]
                n1621 = local read "New: Dielectric"() -> (w2718:dbl)
                n1622 = local write "Sat-Trans Slider"(w2716) -> ()
                n1623 = local write "Lin Id-Used"(w2724) -> ()
                n1624 = local write "Lin-Vg Array-Used"(w2725) -> ()
                n1625 = local write "MobVi Index"(w2716) -> ()
                n1626 = local write "Index 2"(w2733) -> ()
                n1627 = local write "Sqrt-Sat"(w2682) -> ()
                n1628 = local write "Sat-Log"(w2732) -> ()
                n1629 = Unbundle By Name(w2736) -> ("Mobility-Sat"=w2721:dbl, "Vt-Sat"=w2684:dbl, "Mobility-Lin"=w2720:dbl, "Mobility-Lin"=w2719:dbl, "Off I-Sat"=w2714:dbl, "On/Off I-Sat"=w2685:dbl)
                n1630 = local write "Sqrt-Lin"(w2681) -> ()
                n1631 = Array Size(array=w2781) -> (size(s)=w2780:i32[])
                n1632 = local write "Raw- Sat"(w2680) -> ()
                n1633 = local write "New: Temp"(w2687) -> ()
                n1634 = Unbundle By Name(w2731) -> ("STS-Sat"=w2717:dbl)
                n1635 = call "Trap Density_STS.vi"("Temp (T) [K]"=w2687, "S.T.S. (S)"=w2717, "Dielectric"=w2718) -> ("Trap Density (N)"=w2691:dbl)  [unwired: 8 in]
                n1636 = local write "Calc: Mobility-Lin"(w2720) -> ()
                n1637 = local write "Raw- Lin"(w2679) -> ()
                n1638 = local write "Calc: Mobility-Sat"(w2721) -> ()
                n1639 = local write "Log-Lin"(w2678) -> ()
                n1640 = local write "Calc: Off I-Sat"(w2714) -> ()
                n1641 = local write "Calc: VT-Sat"(w2684) -> ()
                n1642 = local write "New: VT-Lin"(w2719) -> ()
                n1643 = local write "New: Trap Density-STS"(w2691) -> ()
                n1644 = local write "Calc: Trap Density-STS"(w2691) -> ()
                n1645 = local read "Image Folder"() -> (w2770:path)
                n1646 = local read "New: Dielectric"() -> (w2715:dbl)
                n1647 = Decimate 1D Array(w2682) -> (w2765:cluster{dbl[], dbl[]}[])  [unwired: 1 out]
                n1648 = Decimate 1D Array(w2732) -> (w2755:cluster{dbl[], dbl[]}[])  [unwired: 1 out]
                n1649 = Index Array(array=w2780, index=w2779) -> (element=w2761:i32)
                n1650 = Array Subset(array=w2781, index (row)=w2779, index (col)=w2779, length (col)=3) -> (w2782:string[][])  [unwired: 1 in]
                n1651 = local write "Calc: STS"(w2717) -> ()
                n1652 = local write "New: VT-Sat"(w2684) -> ()
                n1653 = local write "New: Mobility-Sat"(w2721) -> ()
                n1654 = local write "Calc: On/Off"(w2685) -> ()
                n1655 = local write "New: Mobility-Lin"(w2720) -> ()
                n1656 = List Folder(path=w2770) -> (filenames=w2775:string[])  [unwired: 3 in, 3 out]
                n1657 = local write "New: VT-Lin"(w2719) -> ()
                n1658 = Array To Cluster(array=w2765) -> (cluster=w2767:T13)
                n1659 = Array To Cluster(array=w2755) -> (cluster=w2753:T13)
                n1660 = Reshape Array(w2782, w2761) -> (w2768:string[])
                n1661 = Subtract(x=w2761, y=20) -> (x-y=w2760:i32)
                n1662 = local write "New: STS"(w2717) -> ()
                n1663 = property on="Sat-Trans Slider" class="Slide (strict)"("Scale.Maximum"=w2760) -> ()  [unwired: 2 in, 2 out]
                n1664 = call "Trap Density_VT.vi"("VT"=w2684, "Dielectric"=w2715) -> ("Trap Density-VT"=w2688:dbl)
                n1665 = Unbundle(w2767) -> ("[0]"=w2766:cluster{dbl[], dbl[]})  [unwired: 8 out]
                n1666 = Unbundle(w2753) -> ("[0]"=w2754:cluster{dbl[], dbl[]})  [unwired: 8 out]
                n1667 = Search 1D Array(1D array=w2768, element="Index:") -> (index of element=w2776:i32)  [unwired: 1 in]
                n1668 = local write "New: Trap Density-VT"(w2688) -> ()
                n1669 = local write "Calc: Trap Density-VT"(w2688) -> ()
                n1670 = call-poly <vilib>:"Read From Spreadsheet File.vi"("file path (dialog if empty)"=w2650) -> ("all rows"=w2654:string[][])  [unwired: 6 in, 4 out]
                n1671 = Unbundle(w2766) -> (w2757:dbl[], w2756:dbl[])
                n1672 = Unbundle(w2754) -> (w2752:dbl[], w2751:dbl[])
                n1673 = Increment(x=w2776) -> (x+1=w2777:i32)
                n1674 = Array Size(array=w2654) -> (size(s)=w2673:i32[])
                n1675 = Array Subset(array=w2757, index=w2716, length=w2735) -> (w2764:dbl[])
                n1676 = Array Subset(array=w2756, index=w2716, length=w2735) -> (w2763:dbl[])
                n1677 = Array Subset(array=w2752, index=w2733, length=w2734) -> (w2759:dbl[])
                n1678 = Array Subset(array=w2751, index=w2733, length=w2734) -> (w2758:dbl[])
                n1679 = Index Array(array=w2768, index=w2777) -> (element=w2773:string)
                n1680 = local write "Vg Array-Log-Used"(w2758) -> ()
                n1681 = local write "Sat Id-Log-Used"(w2759) -> ()
                n1682 = local write "Sat Id-Used"(w2763) -> ()
                n1683 = local write "Index"(w2773) -> ()
                n1684 = Index Array(array=w2673, index=0) -> (element=w2671:i32)
                n1685 = local write "Sat Vg Array-Used"(w2764) -> ()
                n1686 = while {
                  tunnel: w2775 -> [w2802]
                  tunnel: w2773 -> [w2800]
                  tunnel: [w2799] -> _
                  tunnel: [w2799] -> w2774
                  tunnel: w2761 -> [w2798]
                  i -> [w2799]
                  stop <- w2795 stop-if-true
                  n1687 = Index Array(array=w2802, index=w2799) -> (element=w2803:string)
                  n1688 = xnode "Match Regular Expression"("input string"=w2803, "regular expression"=w2800) -> ("whole match"=w2801:string)  [unwired: 4 in, 4 out]
                  n1689 = Equal?(x=w2801, y=w2800) -> (x = y?=w2797:bool)
                  n1690 = Equal?(x=w2798, y=w2799) -> (x = y?=w2796:bool)
                  n1691 = Or(x=w2797, y=w2796) -> (x .or. y?=w2795:bool)
                }
                n1692 = Array Subset(array=w2654, index (row)=w2672, index (col)=w2672, length (col)=3) -> (w2674:string[][])  [unwired: 1 in]
                n1693 = Reshape Array(w2674, w2671) -> (w2656:string[])
                n1694 = Search 1D Array(1D array=w2656, element="Vg") -> (index of element=w2660:i32)  [unwired: 1 in]
                n1695 = Add(x=w2660, y=3) -> (x+y=w2658:i32)
                n1696 = Divide(x=w2658, y=3) -> (x/y=w2665:dbl)
                n1697 = Array Subset(array=w2654, index (row)=w2665, index (col)=0, length (col)=1) -> (w2664:string[][])  [unwired: 1 in]
                n1698 = Fract/Exp String To Number(string=w2664) -> (number=w2668:dbl[][])  [unwired: 3 in, 1 out]
                n1699 = Array Size(array=w2668) -> (size(s)=w2655:i32[])
                n1700 = Index Array(array=w2655, index=0) -> (element=w2666:i32)
                n1701 = Decrement(x=w2666) -> (x-1=w2669:i32)
                n1702 = Reshape Array(w2668, w2669) -> (w2653:dbl[])
                n1703 = local write "Data Length"(w2669) -> ()
                n1704 = local write "Vg Column"(w2653) -> ()
                n1705 = Array Max & Min(array=w2653) -> (max value=w2652:dbl, min value=w2651:dbl)  [unwired: 2 out]
                n1706 = Path To String(path=w2770) -> (string=w2772:string)
                n1707 = Index Array(array=w2775, index=w2774) -> (element=w2749:string)
                n1708 = local write "Image Name"(w2749) -> ()
                n1709 = property on="Sat-Trans Slider" class="Slide (strict)"("Scale.Maximum"=w2652, "Scale.Minimum"=w2651) -> ()  [unwired: 2 in, 2 out]
                n1710 = Empty String/Path?(string/path=w2749) -> (empty?=w2750:bool)
                n1711 = Concatenate Strings(w2772, "\\", w2749) -> (w2771:string)
                n1712 = String To Path(string=w2771) -> (path=w2748:path)
                n1713 = local read "No Image File"() -> (w2747:path)
                n1714 = Select(t=w2747, s=w2750, f=w2748) -> (s? t:f=w2741:path)
                n1715 = local write "Image File"(w2741) -> ()
                n1716 = local read "Image Out"() -> (w2739:T2)
                n1717 = call "IMAQ ReadFile"("File Path"=w2741, "Image"=w2739) -> ("Image Out"=w2740:T2)  [unwired: 5 in, 4 out]
                n1718 = local write "Image Out"(w2740) -> ()
                n1719 = local write "Image Out 2"(w2740) -> ()
              }
              frame #4 {
                # "Output ROI data"
                n1720 = local read "Image Folder"() -> (w2918:path)
                n1721 = Build Path(base path=w2918, name or relative path="ROI") -> (appended path=w2920:path)
                n1722 = local read "Index"() -> (w2919:string)
                n1723 = Build Path(base path=w2920, name or relative path=w2919) -> (appended path=w2925:path)
                n1724 = invoke on="Image Out" class="ImageControl" method="Clear ROI"() -> (error out=w2924:errorcluster)  [unwired: 3 in, 2 out]
                n1725 = call <vilib>:"Check if File or Folder Exists.vi"("error in (no error)"=w2924, "path"=w2925) -> ("file or folder exists?"=w2922:bool, "dup path"=w2923:path)  [unwired: 7 in, 1 out]
                n1726 = case shown="True" w2922 {
                  tunnel: w2923 -> [_ w2926]
                  frame False {
                  }
                  frame True {
                    n1727 = Read from Text File(file (use dialog)=w2926) -> (text=w2930:string)  [unwired: 3 in, 3 out]
                    n1728 = property on="Image Out" class="ImageControl"() -> ("ROI"=w2927:T15)  [unwired: 2 in, 2 out]
                    n1729 = Unflatten From String(type=w2927, binary string=w2930) -> (value=w2928:T15, error out=w2929:errorcluster)  [unwired: 3 in, 1 out]
                    n1730 = property on="Image Out" class="ImageControl"(error in=w2929, "ROI"=w2928) -> ()  [unwired: 1 in, 2 out]
                  }
                }
              }
            }
            n1731 = flat-sequence {
              tunnel: [w2113] -> w2100
              tunnel: w2100 -> [w2127]
              frame #0 {
                # "Makes Empty File for Transformer Data"
                n1732 = local read "Transfer Folder"() -> (w2102:path)
                n1733 = Build Path(base path=w2102, name or relative path="Stats") -> (appended path=w2104:path)
                n1734 = call <vilib>:"Check if File or Folder Exists.vi"("path"=w2104) -> ("file or folder exists?"=w2105:bool, "dup path"=w2106:path)  [unwired: 8 in, 1 out]
                n1735 = case shown="False" w2105 {
                  tunnel: [w2110 w2112] -> w2107
                  tunnel: w2106 -> [w2111 w2112]
                  frame False {
                    n1736 = Create Folder(path (use dialog)=w2111) -> (created path=w2110:path)  [unwired: 2 in, 2 out]
                  }
                  frame True {
                  }
                }
                n1737 = Build Path(base path=w2107, name or relative path="Tranformer Data.txt") -> (appended path=w2109:path)
                n1738 = call-poly <vilib>:"Write To Spreadsheet File.vi"("append to file? (new file:F)"=TRUE, "file path (dialog if empty)"=w2109) -> ()  [unwired: 6 in, 1 out]
              }
              frame #1 {
                # "Adds Headers if they don't exist"
                n1739 = local read "Transfer Folder"() -> (w2119:path)
                n1740 = Concatenate Strings("Stats\\", "Tranformer Data.txt") -> (w2120:string)
                n1741 = Build Path(base path=w2119, name or relative path=w2120) -> (appended path=w2113:path)
                n1742 = call-poly <vilib>:"Read From Spreadsheet File.vi"("file path (dialog if empty)"=w2113) -> ("first row"=w2118:string[])  [unwired: 6 in, 4 out]
                n1743 = Search 1D Array(1D array=w2118, element="DeviceID") -> (index of element=w2116:i32)  [unwired: 1 in]
                n1744 = Equal?(x=w2116, y=0) -> (x = y?=w2114:bool)
                n1745 = case shown="False" w2114 {
                  tunnel: w2113 -> [w2124 _]
                  frame False {
                    n1746 = local read "Transformer \nHeaders"() -> (w2123:string[])
                    n1747 = call-poly <vilib>:"Write To Spreadsheet File.vi"("1D data"=w2123, "file path (dialog if empty)"=w2124) -> ()  [unwired: 6 in, 1 out]
                  }
                  frame True {
                  }
                }
              }
              frame #2 {
                # "Adds current device if it doesn't exist"
                n1748 = local read "Current \nRecord"() -> (w2130:string[])
                n1749 = Index Array(array=w2130, index=0) -> (element=w2129:string)
                n1750 = local read "Transfer Folder"() -> (w2132:path)
                n1751 = Concatenate Strings("Stats\\", "Tranformer Data.txt") -> (w2133:string)
                n1752 = local write "Current Device ID"(w2129) -> ()
                n1753 = local read "Current Device ID"() -> (w2139:string)
                n1754 = Build Path(base path=w2132, name or relative path=w2133) -> (appended path=w2131:path)
                n1755 = call-poly <vilib>:"Read From Spreadsheet File.vi"("file path (dialog if empty)"=w2131) -> ("all rows"=w2126:string[][])  [unwired: 6 in, 4 out]
                n1756 = Index Array(array=w2126, index (col)=0) -> (element=w2137:string[])  [unwired: 1 in]
                n1757 = Search 1D Array(1D array=w2137, element=w2139) -> (index of element=w2125:i32)  [unwired: 1 in]
                n1758 = Equal?(x=w2125, y=-1) -> (x = y?=w2128:bool)
                n1759 = case shown="False" w2128 {
                  tunnel: w2127 -> [w2141 w2154]
                  tunnel: w2125 -> [w2146 _]
                  tunnel: w2126 -> [w2147 _]
                  frame False {
                    n1760 = local read "Current \nRecord"() -> (w2145:string[])
                    n1761 = Replace Array Subset(array=w2147, new element=w2145, index (row)=w2146) -> (w2142:string[][])  [unwired: 1 in]
                    n1762 = flat-sequence {
                      tunnel: [w2148] -> _
                      tunnel: [w2149] -> _
                      tunnel: [w2149] -> w2144
                      tunnel: [w2148] -> w2143
                      tunnel: w2142 -> [w2149]
                      tunnel: w2141 -> [w2148]
                      tunnel: w2144 -> [w2151]
                      tunnel: w2143 -> [w2150]
                      frame #0 {
                        n1763 = Delete(path (use dialog)=w2148) -> ()  [unwired: 4 in, 3 out]
                      }
                      frame #1 {
                        n1764 = call-poly <vilib>:"Write To Spreadsheet File.vi"("append to file? (new file:F)"=TRUE, "2D data"=w2151, "file path (dialog if empty)"=w2150) -> ()  [unwired: 5 in, 1 out]
                      }
                    }
                  }
                  frame True {
                    n1765 = local read "Current \nRecord"() -> (w2153:string[])
                    n1766 = call-poly <vilib>:"Write To Spreadsheet File.vi"("append to file? (new file:F)"=TRUE, "1D data"=w2153, "file path (dialog if empty)"=w2154) -> ()  [unwired: 5 in, 1 out]
                  }
                }
              }
            }
          }
          event "Export": Mouse Down {
            n1767 = event-data() -> ()  [unwired: 1 in, 7 out]
            n1768 = flat-sequence {
              frame #0 {
                n1769 = stacked-sequence {
                  frame #0 {
                    n1770 = local read "Independant Variable"() -> (w2932:string)
                    n1771 = Equal?(x=w2932, y="Length (um):") -> (x = y?=w2933:bool)
                    n1772 = case shown="True" w2933 {
                      frame False {
                      }
                      frame True {
                        n1773 = local write "X Axis Display Type"("1") -> ()
                        n1774 = local write "Opj X Axis"("2") -> ()
                      }
                    }
                  }
                  frame #1 {
                    n1775 = local read "Independant Variable"() -> (w2937:string)
                    n1776 = Equal?(x=w2937, y="Sample Temp (K):") -> (x = y?=w2938:bool)
                    n1777 = case shown="True" w2938 {
                      frame False {
                      }
                      frame True {
                        n1778 = local write "X Axis Display Type"("1") -> ()
                        n1779 = local write "Opj X Axis"("1") -> ()
                      }
                    }
                  }
                  frame #2 {
                    n1780 = local read "Independant Variable"() -> (w2942:string)
                    n1781 = Equal?(x=w2942, y="Mobility-Sat (cm^2/Vs):") -> (x = y?=w2943:bool)
                    n1782 = case shown="True" w2943 {
                      frame False {
                      }
                      frame True {
                        n1783 = local write "X Axis Display Type"("2") -> ()
                        n1784 = local write "Opj X Axis"("2") -> ()
                      }
                    }
                  }
                  frame #3 {
                    n1785 = local read "Independant Variable"() -> (w2947:string)
                    n1786 = Equal?(x=w2947, y="Mobility-Lin (cm^2/Vs):") -> (x = y?=w2948:bool)
                    n1787 = case shown="True" w2948 {
                      frame False {
                      }
                      frame True {
                        n1788 = local write "X Axis Display Type"("2") -> ()
                        n1789 = local write "Opj X Axis"("2") -> ()
                      }
                    }
                  }
                  frame #4 {
                    n1790 = local read "Independant Variable"() -> (w2952:string)
                    n1791 = Equal?(x=w2952, y="On/Off I-Sat:") -> (x = y?=w2953:bool)
                    n1792 = case shown="True" w2953 {
                      frame False {
                      }
                      frame True {
                        n1793 = local write "X Axis Display Type"("2") -> ()
                        n1794 = local write "Opj X Axis"("2") -> ()
                      }
                    }
                  }
                  frame #5 {
                    n1795 = local read "Independant Variable"() -> (w2957:string)
                    n1796 = Equal?(x=w2957, y="Off I-Sat (A):") -> (x = y?=w2958:bool)
                    n1797 = case shown="True" w2958 {
                      frame False {
                      }
                      frame True {
                        n1798 = local write "X Axis Display Type"("2") -> ()
                        n1799 = local write "Opj X Axis"("2") -> ()
                      }
                    }
                  }
                  frame #6 {
                    n1800 = local read "Independant Variable"() -> (w2962:string)
                    n1801 = Equal?(x=w2962, y="Vt-Sat (V):") -> (x = y?=w2963:bool)
                    n1802 = case shown="True" w2963 {
                      frame False {
                      }
                      frame True {
                        n1803 = local write "X Axis Display Type"("1") -> ()
                        n1804 = local write "Opj X Axis"("1") -> ()
                      }
                    }
                  }
                  frame #7 {
                    n1805 = local read "Independant Variable"() -> (w2967:string)
                    n1806 = Equal?(x=w2967, y="STS-Sat (V/decade):") -> (x = y?=w2968:bool)
                    n1807 = case shown="True" w2968 {
                      frame False {
                      }
                      frame True {
                        n1808 = local write "X Axis Display Type"("1") -> ()
                        n1809 = local write "Opj X Axis"("1") -> ()
                      }
                    }
                  }
                  frame #8 {
                    n1810 = local read "Independant Variable"() -> (w2972:string)
                    n1811 = Equal?(x=w2972, y="Trap Density-VT (Traps/Vcm^2):") -> (x = y?=w2973:bool)
                    n1812 = case shown="True" w2973 {
                      frame False {
                      }
                      frame True {
                        n1813 = local write "X Axis Display Type"("2") -> ()
                        n1814 = local write "Opj X Axis"("2") -> ()
                      }
                    }
                  }
                  frame #9 {
                    n1815 = local read "Independant Variable"() -> (w2977:string)
                    n1816 = Equal?(x=w2977, y="Trap Density-STS (Traps/Vcm^2):") -> (x = y?=w2978:bool)
                    n1817 = case shown="True" w2978 {
                      frame False {
                      }
                      frame True {
                        n1818 = local write "X Axis Display Type"("2") -> ()
                        n1819 = local write "Opj X Axis"("2") -> ()
                      }
                    }
                  }
                }
              }
              frame #1 {
                n1820 = local read "Transfer Folder"() -> (w2986:path)
                n1821 = Build Path(base path=w2986, name or relative path="Stats") -> (appended path=w2987:path)
                n1822 = local read "Origin Project File"() -> (w2998:path)
                n1823 = call <vilib>:"Check if File or Folder Exists.vi"("path"=w2987) -> ("file or folder exists?"=w3002:bool, "dup path"=w3001:path)  [unwired: 8 in, 1 out]
                n1824 = call <userlib>:"OA_ConnectToOrigin.vi"() -> ("error out"=w2999:errorcluster, "Origin.IOApplication"=w3000:refnum<k7>)  [unwired: 8 in]
                n1825 = case shown="False" w3002 {
                  tunnel: w3001 -> [w3175 w3176]
                  tunnel: [w3174 w3176] -> w2985
                  frame False {
                    n1826 = Create Folder(path (use dialog)=w3175) -> (created path=w3174:path)  [unwired: 2 in, 2 out]
                  }
                  frame True {
                  }
                }
                n1827 = call <userlib>:"OA_Load.vi"("error in (no error)"=w2999, "Path"=w2998, "Origin.IOApplication"=w3000) -> ("error out"=w2996:errorcluster, "Origin.IOApplication"=w2997:refnum<k7>)  [unwired: 1 out]
                n1828 = call "OAExecute.vi"("script"="document -m 3;", "Error IO"=w2996, "Origin.IOApplication"=w2997) -> ("Error IO Out"=w2994:errorcluster, "Origin.IOApplication"=w2995:refnum<k7>)  [unwired: 1 in, 1 out]
                n1829 = call "File Dialog"("start path"=w2987) -> ("selected path"=w2989:path)  [unwired: 11 in, 3 out]
                n1830 = local read "Independant Variable"() -> (w2982:string)
                n1831 = stacked-sequence {
                  tunnel: w2986 -> [w3013 w3043 w3055 w3077 w3097 w3118 w3139 w3162]
                  tunnel: w2985 -> [w3014 w3042 w3056 w3076 w3098 w3119 w3140 w3163]
                  tunnel: w2995 -> [w3016 w3040 w3058 w3079 w3100 w3121 w3142 w3165]
                  tunnel: w2994 -> [w3015 w3041 w3057 w3078 w3099 w3120 w3141 w3164]
                  tunnel: [_ _ _ _ _ _ _ w3160] -> w2984
                  tunnel: [_ _ _ _ _ _ _ w3161] -> w2983
                  tunnel: w2982 -> [w3012 w3033 w3054 w3075 w3096 w3117 w3138 w3159]
                  frame #0 {
                    n1832 = local read "X Axis Display Type"() -> (w3004:string)
                    n1833 = local read "Opj X Axis"() -> (w3009:string)
                    n1834 = Concatenate Strings("window -a MOBLGraph;\nlayer.x.type=", w3009, "; layer.x.label.numFormat = ", w3004, "; Y3 = 1; X3 = 1;", "window -a MOBLTable;\nwindow -s TV;") -> (w3007:string)
                    n1835 = call "Param_Analysis_7_24b_JW.vi"("Independant Variable"=w3012, "error in (no error)"=w3015, "Data Folder"=w3013, "Parameter String"="Mobility-Lin (cm^2/Vs):", "Parameter Name"="Mobility-Lin", "Stats Folder"=w3014) -> ("error out"=w3018:errorcluster, "Output Array"=w3020:string[][], "Variables"=w3011:T20)  [unwired: 2 in, 1 out]
                    n1836 = call "Origin_Export_7_27a_JW.vi"("Input Conditions"=w3011, "Analysis Array"=w3020, "error in (no error)"=w3018, "Parameter Worksheet Name"="[MOBLTable]Mobilities", "Parameter Folder Script"="pe_cd \"Mobility-Lin\";", "Origin.IOApplication"=w3016) -> ("error out"=w3017:errorcluster, "reference out"=w3019:refnum<k7>)  [unwired: 3 in, 1 out]
                    n1837 = call "OAExecute.vi"("script"=w3007, "Error IO"=w3017, "Origin.IOApplication"=w3019) -> ()  [unwired: 1 in, 3 out]
                  }
                  frame #1 {
                    n1838 = local read "X Axis Display Type"() -> (w3025:string)
                    n1839 = local read "Opj X Axis"() -> (w3030:string)
                    n1840 = Concatenate Strings("window -a MOBSGraph;\nlayer.x.type=", w3030, "; layer.x.label.numFormat = ", w3025, "; Y3 = 1; X3 = 1;", "window -a MOBSTable;\nwindow -s TV;") -> (w3028:string)
                    n1841 = call "Param_Analysis_7_24b_JW.vi"("Independant Variable"=w3033, "error in (no error)"=w3041, "Data Folder"=w3043, "Parameter String"="Mobility-Sat (cm^2/Vs):", "Parameter Name"="Mobility-Sat", "Stats Folder"=w3042) -> ("error out"=w3036:errorcluster, "Output Array"=w3034:string[][], "Variables"=w3032:T20)  [unwired: 2 in, 1 out]
                    n1842 = call "Origin_Export_7_27a_JW.vi"("Input Conditions"=w3032, "Analysis Array"=w3034, "error in (no error)"=w3036, "Parameter Worksheet Name"="[MOBSTable]Mobilities", "Parameter Folder Script"="pe_cd \"Mobility-Sat\";", "Origin.IOApplication"=w3040) -> ("error out"=w3035:errorcluster, "reference out"=w3037:refnum<k7>)  [unwired: 3 in, 1 out]
                    n1843 = call "OAExecute.vi"("script"=w3028, "Error IO"=w3035, "Origin.IOApplication"=w3037) -> ()  [unwired: 1 in, 3 out]
                  }
                  frame #2 {
                    n1844 = local read "X Axis Display Type"() -> (w3046:string)
                    n1845 = local read "Opj X Axis"() -> (w3051:string)
                    n1846 = Concatenate Strings("window -a NSTSGraph;\nlayer.x.type=", w3051, "; layer.x.label.numFormat = ", w3046, "; Y3 = 1; X3 = 1;", "window -a NSTSTable;\nwindow -s TV;") -> (w3049:string)
                    n1847 = call "Param_Analysis_7_24b_JW.vi"("Independant Variable"=w3054, "error in (no error)"=w3057, "Data Folder"=w3055, "Parameter String"="Trap Density-STS (Traps/Vcm^2):", "Parameter Name"="Trap Density-STS", "Stats Folder"=w3056) -> ("error out"=w3061:errorcluster, "Output Array"=w3059:string[][], "Variables"=w3053:T20)  [unwired: 2 in, 1 out]
                    n1848 = call "Origin_Export_7_27a_JW.vi"("Input Conditions"=w3053, "Analysis Array"=w3059, "error in (no error)"=w3061, "Parameter Worksheet Name"="[NSTSTable]Trap Densities", "Parameter Folder Script"="pe_cd \"N-STS\";", "Origin.IOApplication"=w3058) -> ("error out"=w3060:errorcluster, "reference out"=w3062:refnum<k7>)  [unwired: 3 in, 1 out]
                    n1849 = call "OAExecute.vi"("script"=w3049, "Error IO"=w3060, "Origin.IOApplication"=w3062) -> ()  [unwired: 1 in, 3 out]
                  }
                  frame #3 {
                    n1850 = local read "X Axis Display Type"() -> (w3067:string)
                    n1851 = local read "Opj X Axis"() -> (w3072:string)
                    n1852 = call "Param_Analysis_7_24b_JW.vi"("Independant Variable"=w3075, "error in (no error)"=w3078, "Data Folder"=w3077, "Parameter String"="Trap Density-VT (Traps/Vcm^2):", "Parameter Name"="Trap Density-Vt", "Stats Folder"=w3076) -> ("error out"=w3082:errorcluster, "Output Array"=w3080:string[][], "Variables"=w3074:T20)  [unwired: 2 in, 1 out]
                    n1853 = Concatenate Strings("window -a NVtGraph;\nlayer.x.type=", w3072, "; layer.x.label.numFormat = ", w3067, "; Y3 = 1; X3 = 1;", "window -a NVtTable;\nwindow -s TV;") -> (w3070:string)
                    n1854 = call "Origin_Export_7_27a_JW.vi"("Input Conditions"=w3074, "Analysis Array"=w3080, "error in (no error)"=w3082, "Parameter Worksheet Name"="[NVTTable]Trap Densities", "Parameter Folder Script"="pe_cd \"N-Vt\";", "Origin.IOApplication"=w3079) -> ("error out"=w3081:errorcluster, "reference out"=w3083:refnum<k7>)  [unwired: 3 in, 1 out]
                    n1855 = call "OAExecute.vi"("script"=w3070, "Error IO"=w3081, "Origin.IOApplication"=w3083) -> ()  [unwired: 1 in, 3 out]
                  }
                  frame #4 {
                    n1856 = local read "X Axis Display Type"() -> (w3088:string)
                    n1857 = local read "Opj X Axis"() -> (w3093:string)
                    n1858 = Concatenate Strings("window -a OffIGraph;\nlayer.x.type=", w3093, "; layer.x.label.numFormat = ", w3088, "; Y3 = 1; X3 = 1;", "window -a OffITable;\nwindow -s TV;") -> (w3091:string)
                    n1859 = call "Param_Analysis_7_24b_JW.vi"("Independant Variable"=w3096, "error in (no error)"=w3099, "Data Folder"=w3097, "Parameter String"="Off I-Sat (A):", "Parameter Name"="Off I-Sat", "Stats Folder"=w3098) -> ("error out"=w3103:errorcluster, "Output Array"=w3101:string[][], "Variables"=w3095:T20)  [unwired: 2 in, 1 out]
                    n1860 = call "Origin_Export_7_27a_JW.vi"("Input Conditions"=w3095, "Analysis Array"=w3101, "error in (no error)"=w3103, "Parameter Worksheet Name"="[OffItable]OffCurrents", "Parameter Folder Script"="pe_cd \"OffI-Sat\";", "Origin.IOApplication"=w3100) -> ("error out"=w3102:errorcluster, "reference out"=w3104:refnum<k7>)  [unwired: 3 in, 1 out]
                    n1861 = call "OAExecute.vi"("script"=w3091, "Error IO"=w3102, "Origin.IOApplication"=w3104) -> ()  [unwired: 1 in, 3 out]
                  }
                  frame #5 {
                    n1862 = local read "X Axis Display Type"() -> (w3109:string)
                    n1863 = local read "Opj X Axis"() -> (w3114:string)
                    n1864 = Concatenate Strings("window -a OnOffGraph;\nlayer.x.type=", w3114, "; layer.x.label.numFormat = ", w3109, "; Y3 = 1; X3 = 1;", "window -a OnOffTable;\nwindow -s TV;") -> (w3112:string)
                    n1865 = call "Param_Analysis_7_24b_JW.vi"("Independant Variable"=w3117, "error in (no error)"=w3120, "Data Folder"=w3118, "Parameter String"="On/Off I-Sat:", "Parameter Name"="OnOff Ratio", "Stats Folder"=w3119) -> ("error out"=w3124:errorcluster, "Output Array"=w3122:string[][], "Variables"=w3116:T20)  [unwired: 2 in, 1 out]
                    n1866 = call "Origin_Export_7_27a_JW.vi"("Input Conditions"=w3116, "Analysis Array"=w3122, "error in (no error)"=w3124, "Parameter Worksheet Name"="[OnOffTable]On/Off Ratios", "Parameter Folder Script"="pe_cd \"OnOff-Ratio\";", "Origin.IOApplication"=w3121) -> ("error out"=w3123:errorcluster, "reference out"=w3125:refnum<k7>)  [unwired: 3 in, 1 out]
                    n1867 = call "OAExecute.vi"("script"=w3112, "Error IO"=w3123, "Origin.IOApplication"=w3125) -> ()  [unwired: 1 in, 3 out]
                  }
                  frame #6 {
                    n1868 = local read "X Axis Display Type"() -> (w3130:string)
                    n1869 = local read "Opj X Axis"() -> (w3135:string)
                    n1870 = call "Param_Analysis_7_24b_JW.vi"("Independant Variable"=w3138, "error in (no error)"=w3141, "Data Folder"=w3139, "Parameter String"="STS-Sat (V/decade):", "Parameter Name"="STS-Sat", "Stats Folder"=w3140) -> ("error out"=w3145:errorcluster, "Output Array"=w3143:string[][], "Variables"=w3137:T20)  [unwired: 2 in, 1 out]
                    n1871 = Concatenate Strings("window -a SGraph;\nlayer.x.type=", w3135, "; layer.x.label.numFormat = ", w3130, "; Y3 = 1; X3 = 1;", "window -a STable;\nwindow -s TV;") -> (w3133:string)
                    n1872 = call "Origin_Export_7_27a_JW.vi"("Input Conditions"=w3137, "Analysis Array"=w3143, "error in (no error)"=w3145, "Parameter Worksheet Name"="[STable]Threshold Swing", "Parameter Folder Script"="pe_cd \"STS-Sat\";", "Origin.IOApplication"=w3142) -> ("error out"=w3144:errorcluster, "reference out"=w3146:refnum<k7>)  [unwired: 3 in, 1 out]
                    n1873 = call "OAExecute.vi"("script"=w3133, "Error IO"=w3144, "Origin.IOApplication"=w3146) -> ()  [unwired: 1 in, 3 out]
                  }
                  frame #7 {
                    n1874 = local read "X Axis Display Type"() -> (w3151:string)
                    n1875 = local read "Opj X Axis"() -> (w3156:string)
                    n1876 = Concatenate Strings("window -a VtGraph;\nlayer.x.type=", w3156, "; layer.x.label.numFormat = ", w3151, "; Y3 = 1; X3 = 1;", "window -a VtTable;\nwindow -s TV;") -> (w3154:string)
                    n1877 = call "Param_Analysis_7_24b_JW.vi"("Independant Variable"=w3159, "error in (no error)"=w3164, "Data Folder"=w3162, "Parameter String"="Vt-Sat (V):", "Parameter Name"="Vt-Sat", "Stats Folder"=w3163) -> ("error out"=w3168:errorcluster, "Output Array"=w3166:string[][], "Variables"=w3158:T20)  [unwired: 2 in, 1 out]
                    n1878 = call "Origin_Export_7_27a_JW.vi"("Input Conditions"=w3158, "Analysis Array"=w3166, "error in (no error)"=w3168, "Parameter Worksheet Name"="[VtTable]Threshold Voltages", "Parameter Folder Script"="pe_cd \"Vt-Sat\";", "Origin.IOApplication"=w3165) -> ("error out"=w3167:errorcluster, "reference out"=w3169:refnum<k7>)  [unwired: 3 in, 1 out]
                    n1879 = call "OAExecute.vi"("script"=w3154, "Error IO"=w3167, "Origin.IOApplication"=w3169) -> ("Error IO Out"=w3160:errorcluster, "Origin.IOApplication"=w3161:refnum<k7>)  [unwired: 1 in, 1 out]
                  }
                }
                n1880 = Path To String(path=w2989) -> (string=w2988:string)
                n1881 = call "OAExecute.vi"("script"="pe_cd /; ", "Error IO"=w2984, "Origin.IOApplication"=w2983) -> ("Error IO Out"=w2990:errorcluster, "Origin.IOApplication"=w2991:refnum<k7>)  [unwired: 1 in, 1 out]
                n1882 = call <userlib>:"OASaveProject.vi"("path"=w2988, "Error IO"=w2990, "Origin.IOApplication"=w2991) -> ()  [unwired: 3 out]
              }
            }
          }
          event "Blank Button": Mouse Down {
            n1883 = event-data() -> ()  [unwired: 1 in, 7 out]
            n1884 = local read "Transfer File"() -> (w3184:path)
            n1885 = disable-structure shown="Disabled" {
              frame Disabled {
                n1886 = local read "Folder Index"() -> (w3185:dbl)
                n1887 = Decrement(x=w3185) -> (x-1=w3186:dbl)
                n1888 = local write "Folder Index"(w3186) -> ()
              }
              frame Enabled {
              }
            }
            n1889 = Strip Path(path=w3184) -> (stripped path=w3180:path, name=w3182:string)
            n1890 = Path To String(path=w3180) -> (string=w3179:string)
            n1891 = Concatenate Strings(w3179, "\\", "X_", w3182) -> (w3178:string)
            n1892 = String To Path(string=w3178) -> (path=w3177:path)
            n1893 = Move(source path=w3184, 10:w3177) -> ()  [unwired: 3 in, 3 out]
            n1894 = local write "Transfer File"(w3177) -> ()
          }
          event "Cancel Button": Mouse Down {
            (unwired) 6
            n1895 = event-data() -> ()  [unwired: 1 in, 7 out]
            n1896 = call "Simulate_Keyboard.vi"("Action"=2, "Virtual Key"=162) -> ()  [unwired: 7 in, 1 out]
          }
        }
        n1897 = Multiply(x=w175, y=10) -> (x*y=w177:sgl)
        n1898 = Subtract(x=w191, y=w194) -> (x-y=w192:dbl)
        n1899 = Add(x=w192, y=w188) -> (x+y=w206:dbl)
        n1900 = Add(x=w193, y=w189) -> (x+y=w207:dbl)
        n1901 = case shown="\"0\"" w216 {
          tunnel: w190 -> [w355 w361 w365 w367 w371 w373 w375 w377 w379 w381 w383 w385 w387 w389 w391 w393 w395 w397 w399 w401 w403 w405 w407 w409 w411 w413 w415 w417 w419 w421 w423 w425 w427 w429 w431 w433 w435 w437 w439 w441 w443 w445 w447 w449 w451 w453 w455 w457 w459 w461 w463 w465 w467 w469 w471 w473 w475 w477 w479 w481 w483 w485 w487 w489 w491 w493 w495 w497 w499 w501 w503 w505 w507 w509 w511 w513 w515 w517 w519 w521 w523 w525 w527 w529 w531 w533 w535 w537 w539 w541 w543 w545 w547 w549 w551 w553 w555 w557 w559 w561 w563 w565 w567 w569 w571]
          tunnel: [w355 w360 w364 w367 w371 w373 w375 w377 w379 w381 w383 w385 w387 w389 w391 w393 w395 w397 w399 w401 w403 w405 w407 w409 w411 w413 w415 w417 w419 w421 w423 w425 w427 w429 w431 w433 w435 w437 w439 w441 w443 w445 w447 w449 w451 w453 w455 w457 w459 w461 w463 w465 w467 w469 w471 w473 w475 w477 w479 w481 w483 w485 w487 w489 w491 w493 w495 w497 w499 w501 w503 w505 w507 w509 w511 w513 w515 w517 w519 w521 w523 w525 w527 w529 w531 w533 w535 w537 w539 w541 w543 w545 w547 w549 w551 w553 w555 w557 w559 w561 w563 w565 w567 w569 w571] -> w215
          tunnel: w191 -> [w357 w359 w363 w369 w370 w372 w374 w376 w378 w380 w382 w384 w386 w388 w390 w392 w394 w396 w398 w400 w402 w404 w406 w408 w410 w412 w414 w416 w418 w420 w422 w424 w426 w428 w430 w432 w434 w436 w438 w440 w442 w444 w446 w448 w450 w452 w454 w456 w458 w460 w462 w464 w466 w468 w470 w472 w474 w476 w478 w480 w482 w484 w486 w488 w490 w492 w494 w496 w498 w500 w502 w504 w506 w508 w510 w512 w514 w516 w518 w520 w522 w524 w526 w528 w530 w532 w534 w536 w538 w540 w542 w544 w546 w548 w550 w552 w554 w556 w558 w560 w562 w564 w566 w568 w570]
          tunnel: [w356 w359 w363 w368 w370 w372 w374 w376 w378 w380 w382 w384 w386 w388 w390 w392 w394 w396 w398 w400 w402 w404 w406 w408 w410 w412 w414 w416 w418 w420 w422 w424 w426 w428 w430 w432 w434 w436 w438 w440 w442 w444 w446 w448 w450 w452 w454 w456 w458 w460 w462 w464 w466 w468 w470 w472 w474 w476 w478 w480 w482 w484 w486 w488 w490 w492 w494 w496 w498 w500 w502 w504 w506 w508 w510 w512 w514 w516 w518 w520 w522 w524 w526 w528 w530 w532 w534 w536 w538 w540 w542 w544 w546 w548 w550 w552 w554 w556 w558 w560 w562 w564 w566 w568 w570] -> w214
          tunnel: w177 -> [w354 w358 w362 w366 _ _ _ _ _ _ _ _ _ _ _ _ _ _ _ _ _ _ _ _ _ _ _ _ _ _ _ _ _ _ _ _ _ _ _ _ _ _ _ _ _ _ _ _ _ _ _ _ _ _ _ _ _ _ _ _ _ _ _ _ _ _ _ _ _ _ _ _ _ _ _ _ _ _ _ _ _ _ _ _ _ _ _ _ _ _ _ _ _ _ _ _ _ _ _ _ _ _ _ _ _]
          frame "DOWN" {
            n1902 = Add(x=w357, y=w354) -> (x+y=w356:sgl)
          }
          frame "LEFT" {
            n1903 = Subtract(x=w361, y=w358) -> (x-y=w360:sgl)
          }
          frame "RIGHT" {
            n1904 = Add(x=w365, y=w362) -> (x+y=w364:sgl)
          }
          frame "UP" {
            n1905 = Subtract(x=w369, y=w366) -> (x-y=w368:sgl)
          }
          frame "ENTER (num pad)" {
          }
          frame "' (quote)" {
          }
          frame "END" {
          }
          frame "EQUALS" {
          }
          frame "ESCAPE" {
          }
          frame "GRAVE (`)" {
          }
          frame "HOME" {
          }
          frame "INSERT" {
          }
          frame "LBRACKET" {
          }
          frame "LCONTROL" {
          }
          frame "L ALT" {
          }
          frame "LSHIFT" {
          }
          frame "LWIN" {
          }
          frame "MINUS" {
          }
          frame "MULTIPLY" {
          }
          frame "NEXT" {
          }
          frame "NUMLOCK" {
          }
          frame "NUMPAD_0" {
          }
          frame "NUMPAD_1" {
          }
          frame "NUMPAD_2" {
          }
          frame "NUMPAD_3" {
          }
          frame "NUMPAD_4" {
          }
          frame "NUMPAD_5" {
          }
          frame "NUMPAD_6" {
          }
          frame "NUMPAD_7" {
          }
          frame "NUMPAD_8" {
          }
          frame "NUMPAD_9" {
          }
          frame "PAUSE" {
          }
          frame "PERIOD" {
          }
          frame "PRIOR (PG UP)" {
          }
          frame "RBRACKET" {
          }
          frame "RCONTROL" {
          }
          frame "RETURN" {
          }
          frame "R ALT" {
          }
          frame "RSHIFT" {
          }
          frame "RWIN" {
          }
          frame "SCROLL" {
          }
          frame "SEMICOLON" {
          }
          frame "SLASH" {
          }
          frame "SPACE" {
          }
          frame "SUBTRACT" {
          }
          frame "TAB" {
          }
          frame "DIVIDE" {
          }
          frame "DELETE" {
          }
          frame "DECIMAL" {
          }
          frame "COMMA" {
          }
          frame "CAPITAL" {
          }
          frame "BACKSLASH" {
          }
          frame "BACK" {
          }
          frame "ADD" {
          }
          frame "F15" {
          }
          frame "F14" {
          }
          frame "F13" {
          }
          frame "F12" {
          }
          frame "F11" {
          }
          frame "F10" {
          }
          frame "F9" {
          }
          frame "F8" {
          }
          frame "F7" {
          }
          frame "F6" {
          }
          frame "F5" {
          }
          frame "F4" {
          }
          frame "F3" {
          }
          frame "F2" {
          }
          frame "F1" {
          }
          frame "Z" {
          }
          frame "Y" {
          }
          frame "X" {
          }
          frame "W" {
          }
          frame "V" {
          }
          frame "U" {
          }
          frame "T" {
          }
          frame "S" {
          }
          frame "R" {
          }
          frame "Q" {
          }
          frame "P" {
          }
          frame "O" {
          }
          frame "N" {
          }
          frame "M" {
          }
          frame "L" {
          }
          frame "K" {
          }
          frame "J" {
          }
          frame "I" {
          }
          frame "H" {
          }
          frame "G" {
          }
          frame "F" {
          }
          frame "E" {
          }
          frame "D" {
          }
          frame "C" {
          }
          frame "B" {
          }
          frame "A" {
          }
          frame "9" {
          }
          frame "8" {
          }
          frame "7" {
          }
          frame "6" {
          }
          frame "5" {
          }
          frame "4" {
          }
          frame "3" {
          }
          frame "2" {
          }
          frame "1" {
          }
          frame "0" {
          }
        }
        n1906 = Bundle(w193, w192, w207, w206, 0.0) -> (w205:cluster{dbl, dbl, dbl, dbl, dbl})  [unwired: 1 in]
        n1907 = Bundle("X"=w215, "Y"=w214) -> (w209:cluster{"X":sgl, "Y":sgl})  [unwired: 1 in]
        n1908 = Divide(x=20, y=w176) -> (x/y=w179:sgl)
        n1909 = call "IMAQ Convert Rectangle to ROI (Polygon)"("Rectangle"=w205) -> ("ROI Descriptor"=w203:T5)  [unwired: 7 in, 2 out]
        n1910 = property on="Image Out" class="ImageControl"("Image Center Position"=w209) -> ()  [unwired: 2 in, 2 out]
        n1911 = property on="Image Out 2" class="ImageControl"("ROI"=w203) -> ()  [unwired: 2 in, 2 out]
        n1912 = Bundle("Application Font", w179, w183, w183, w183, w183, w183, TRUE, w181) -> (w185:T21)  [unwired: 1 in]
        n1913 = Bundle(w181, w185, w181, w181) -> (w184:T22)  [unwired: 1 in]
        n1914 = property on="Image Out" class="ImageControl"() -> ("ROI"=w168:T15)  [unwired: 2 in, 2 out]
        n1915 = local read "Image Out"() -> (w187:T2)
        n1916 = local write "ROI Descriptor"(w168) -> ()
        n1917 = property on="Image Out" class="ImageControl"() -> ("ZoomInteger"=w211:cluster{"X":i32, "Y":i32})  [unwired: 2 in, 2 out]
        n1918 = Unbundle By Name(w168) -> ("Contours"=w232:T16)
        n1919 = Unbundle(w211) -> ("X"=w210:i32)  [unwired: 1 out]
        n1920 = call "IMAQ Clear Overlay"("Image"=w187) -> ("Image Out"=w186:T2)  [unwired: 9 in, 1 out]
        n1921 = Initialize Array(0) -> (w230:i32[])  [unwired: 1 in]
        n1922 = Array Size(array=w232) -> (size(s)=w231:i32)
        n1923 = local write "Zoom"(w210) -> ()
        n1924 = local read "Magnification"() -> (w221:u16)
        n1925 = Build Array(0.505025, 0.252522, 0.127742, 0.050345, 0.031129) -> (w222:dbl[])
        n1926 = Array Subset(array=w222, index=w221, length=1) -> (w219:dbl[])
        n1927 = To Double Precision Float(number=w219) -> (double precision float=w218:dbl[])
        n1928 = for {
          N: w231 -> [_]
          shift-right: [w594] -> _
          shift-left: w232 -> [w594]
          shift-right: [w592] -> w217
          shift-left: w230 -> [w591]
          tunnel: w218 -> [w590]
          shift-right: [w587] -> _
          shift-left: w186 -> [w589]
          tunnel: w184 -> [w582]
          i -> [w586]
          n1929 = Index Array(array=w594, index=w586) -> (element=w603:T23)
          n1930 = Unbundle(w603) -> ("Points"=w602:i32[])  [unwired: 2 out]
          n1931 = Array To Cluster(array=w602) -> (cluster=w601:T24)
          n1932 = Unbundle(w601) -> ("Points[0]"=w581:i32, "Points[1]"=w578:i32, "Points[2]"=w593:i32, "Points[3]"=w599:i32)  [unwired: 5 out]
          n1933 = Add(x=w581, y=10) -> (x+y=w579:i32)
          n1934 = Subtract(x=w578, y=w599) -> (x-y=w598:i32)
          n1935 = Subtract(x=w581, y=w593) -> (x-y=w600:i32)
          n1936 = Square(x=w598) -> (x^2=w596:i32)
          n1937 = Square(x=w600) -> (x^2=w597:i32)
          n1938 = Add(x=w597, y=w596) -> (x+y=w595:i32)
          n1939 = Square Root(x=w595) -> (sqrt(x)=w572:dbl)
          n1940 = Multiply(x=w572, y=0.5) -> (x*y=w575:dbl)
          n1941 = Add(x=w575, y=w578) -> (x+y=w577:dbl)
          n1942 = Bundle(w579, w577) -> (w588:cluster{i32, dbl})  [unwired: 1 in]
          n1943 = Multiply(x=w572, y=w590) -> (x*y=w585:dbl[])
          n1944 = Index Array(array=w585) -> (element=w584:dbl)  [unwired: 1 in]
          n1945 = Number To Fractional String(number=w584) -> (F-format string=w583:string)  [unwired: 3 in]
          n1946 = call "IMAQ Overlay Text"("BG Color (Transparent)"=u32 0, "Text Color (black)"=u32 16448250, "Font, Size & Style"=w582, "String"=w583, "Origin"=w588, "Image"=w589) -> ("Image Out"=w587:T2)  [unwired: 4 in, 1 out]
          n1947 = Build Array (concatenate)(w591, w585) -> (w592:dbl[])
        }
        n1948 = Add Array Elements(numeric array=w217) -> (sum=w228:dbl)
        n1949 = local write "Total Width"(w228) -> ()
        n1950 = local write "Distances"(w217) -> ()
        n1951 = local read "Manual-Width"() -> (w134:bool)
        n1952 = local read "Total Width"() -> (w171:dbl)
        n1953 = local read "Rec: Width"() -> (w169:dbl)
        n1954 = case shown="False" w134 {
          frame False {
            n1955 = property on="New: Width" class="DigNum (strict)"("DisabledEnum"=1) -> ()  [unwired: 2 in, 2 out]
          }
          frame True {
            n1956 = property on="New: Width" class="DigNum (strict)"("DisabledEnum"=0) -> ()  [unwired: 2 in, 2 out]
          }
        }
        n1957 = Not(x=w134) -> (.not. x?=w166:bool)
        n1958 = Equal To 0?(x=w171) -> (x = 0?=w167:bool)
        n1959 = Or(x=w167, y=w134) -> (x .or. y?=w170:bool)
        n1960 = And(x=w167, y=w166) -> (x .and. y?=w165:bool)
        n1961 = case shown="True" w165 {
          tunnel: w169 -> [_ w330]
          frame False {
          }
          frame True {
            n1962 = local write "New: Width"(w330) -> ()
          }
        }
        n1963 = case shown="False" w170 {
          tunnel: w171 -> [w332 _]
          frame False {
            n1964 = local write "New: Width"(w332) -> ()
            n1965 = property on="New: Width" class="DigNum (strict)"("DisabledEnum"=1) -> ()  [unwired: 2 in, 2 out]
          }
          frame True {
            n1966 = property on="New: Width" class="DigNum (strict)"("DisabledEnum"=0) -> ()  [unwired: 2 in, 2 out]
          }
        }
        n1967 = local read "Manual Comments"() -> (w135:bool)
        n1968 = local read "Rec: Comments"() -> (w136:string)
        n1969 = local read "Manuel-Dielectric"() -> (w162:bool)
        n1970 = local read "Rec: Dielectric (d)"() -> (w161:dbl)
        n1971 = local read "Manuel-Length"() -> (w163:bool)
        n1972 = local read "Rec: Length"() -> (w164:dbl)
        n1973 = case shown="True" w135 {
          tunnel: w136 -> [w313 _]
          frame False {
            n1974 = local write "Comments:"(w313) -> ()
            n1975 = property on="Comments:" class="Str"("DisabledEnum"=1) -> ()  [unwired: 2 in, 2 out]
          }
          frame True {
            n1976 = property on="Comments:" class="Str"("DisabledEnum"=0) -> ()  [unwired: 2 in, 2 out]
          }
        }
        n1977 = case shown="True" w163 {
          tunnel: w164 -> [w328 _]
          frame False {
            n1978 = local write "New: Length"(w328) -> ()
            n1979 = property on="New: Length" class="DigNum (strict)"("DisabledEnum"=1) -> ()  [unwired: 2 in, 2 out]
          }
          frame True {
            n1980 = property on="New: Length" class="DigNum (strict)"("DisabledEnum"=0) -> ()  [unwired: 2 in, 2 out]
          }
        }
        n1981 = case shown="True" w162 {
          tunnel: w161 -> [w325 _]
          frame False {
            n1982 = local write "New: Dielectric"(w325) -> ()
            n1983 = property on="New: Dielectric" class="DigNum (strict)"("DisabledEnum"=1) -> ()  [unwired: 2 in, 2 out]
          }
          frame True {
            n1984 = property on="New: Dielectric" class="DigNum (strict)"("DisabledEnum"=0) -> ()  [unwired: 2 in, 2 out]
          }
        }
      }
    }
  }
  n1985 = disable-structure shown="Disabled" {
    frame Disabled {
      # "Transformer Work"
      n1986 = Build Array("DeviceID", "Fabricator", "Deposition", "Date", "Sample", "Row", "Column", "L (um)", "W (um)", "Material", "Treatment", "TC (mM)", "Solvent", "C (%)", "ST (C)", "Drops", "Wait (s)", "RT (F)", "RH (%)", "Ramp (s)", "RPM", "Accel (RPM/s)", "Time (s)", "Mobility", "On/Off", "Vt", "S.T.S") -> (→"Transformer \nHeaders":string[])
    }
    frame Enabled {
    }
  }
